vi "HandleObservationAsync.vi"(8 "error in (no error)":errorcluster, 10 "Acquisition.lvclass In":refnum<class "Acquisition.lvclass">, 11 "S4ACS_GUI in":refnum<class "S4GUI.lvclass">) -> (0 "error out":errorcluster, 2 "Acquisition.lvclass Out":refnum<class "Acquisition.lvclass">, 3 "S4ACS_GUI out":refnum<class "S4GUI.lvclass">)   [LabVIEW 2018, in "S4GUI.lvclass"]
uses:
  S4GUI.lvclass
  Acquisition/Acquisition.lvclass
  S4GUI.lvclass/S4GUI.ctl
  Instrument/Instrument.lvclass/Instrument.ctl
  Device/Optics/Optics.lvclass/Optics.ctl
  Interface/Interface.lvclass/Interface.ctl
  Server/Server.lvclass/Server.ctl
  Device/Optics/Opt_Selector/Opt_Selector.lvclass
  Instrument/Instrument.lvclass
  StateMachine/State Machine.lvclass
  SyncBox/Sync Box.lvclass
  Trigger/Trigger.lvclass
  Channel/Channel.lvclass
  Interface/Interface.lvclass
  TelFocus/TelFocus.lvclass
  SecMirror/SecMirror.lvclass
  Device/Optics/Optics.lvclass
  Server/Server.lvclass
panel:
  out "time308":u32
  out "time307":u32
  out "time9":u32
  out "delay 89":u32
  out "time 10":u32
  out "time elapsed 2":u32
  out "time 8":u32
  out "delay 78":u32
  out "time7":u32
  out "time6":u32
  out "time5":u32
  out "delay 3-4":u32
  out "time4":u32
  out "time3":u32
  out "time 2":u32
  out "time1":u32
  # "ACS DELAY"
  # "WAVEPLATE DURATION"
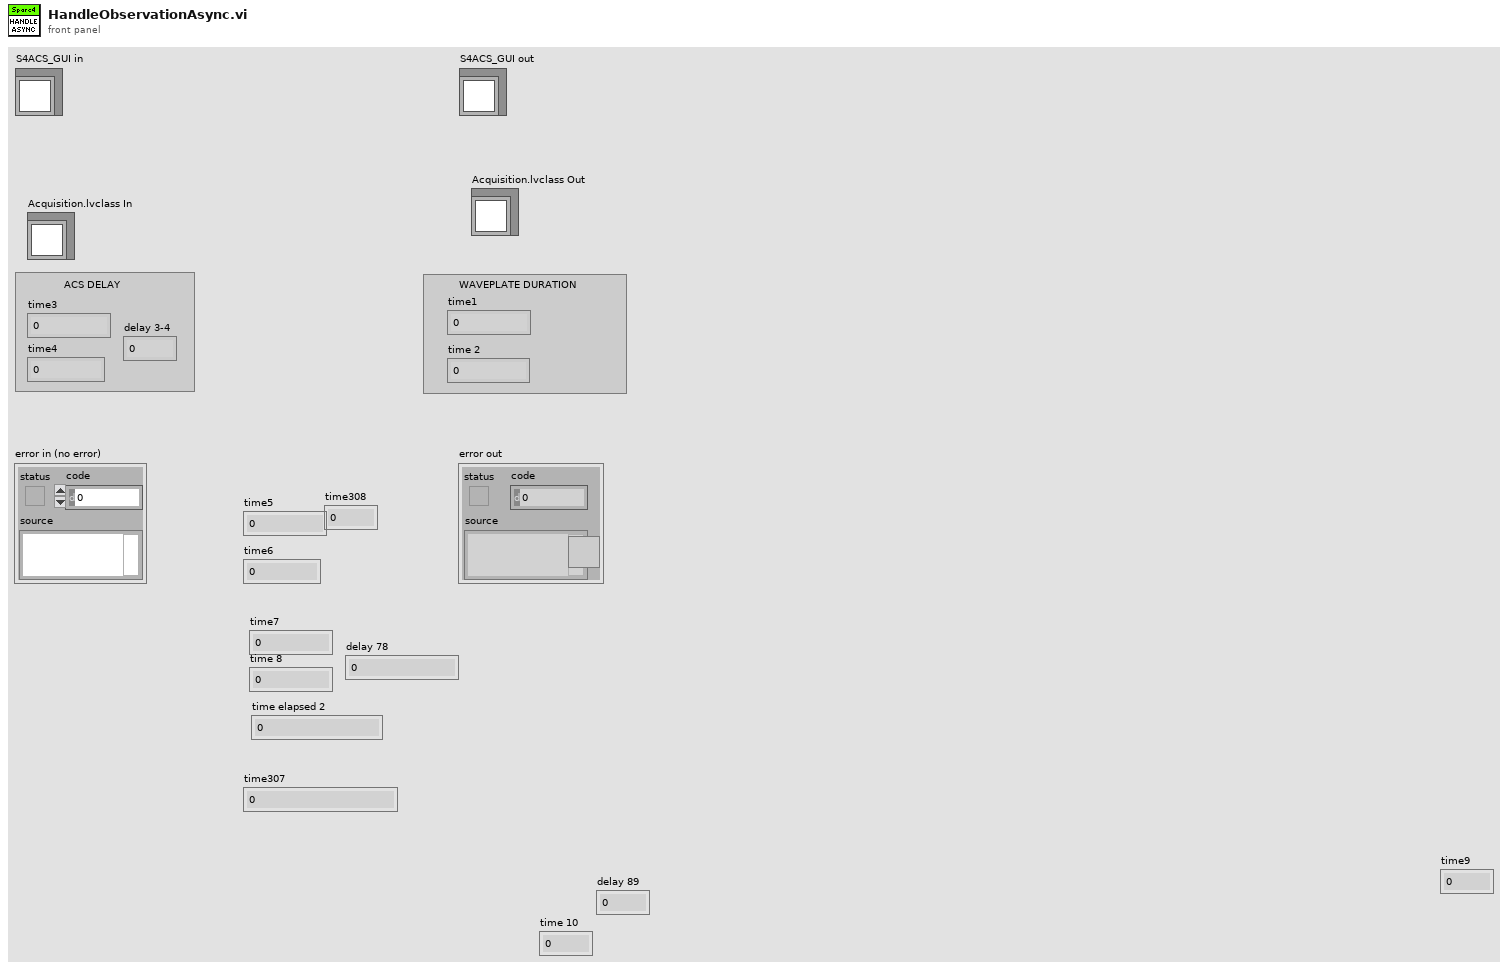
[diagram p1: front panel]
types:
  T1 = cluster{"ACQUISITION_MODE":u8, "TRIGGER_MODE":u8, "READ_MODE":u8, "PREAMP":u8, "READOUT_RATE":u8, "VERTICAL_SHIFT_SPEED":u8, "EM_MODE":u8, "EM_GAIN":u16, "SHUTTER_MODE":u8, "SHUTTER_TTL":u8, "SHUTTER_OPENING_TIME":u16, "SHUTTER_CLOSING_TIME":u16, "VBIN":u16, "HBIN":u16, "INITIAL_LINE":u16, "INITIAL_COLUMN":u16, "FINAL_LINE":u16, "FINAL_COLUMN":u16, "FRAME_TRANSFER":bool, "VERTICAL_CLOCK_VOLTAGE":u8, "AD_CHANNEL":u32}
  T2 = cluster{"Texp":dbl, "Nimages":u32, "InitialLine":u32, "FinalLine":u32, "InitialColumn":u32, "FinalColumn":u32, "EmGain":u32, "Cooler Off":bool, "CyclesDone":u32, "SequesDone":u32, "UsedDiskSpace":u16, "Error":bool}
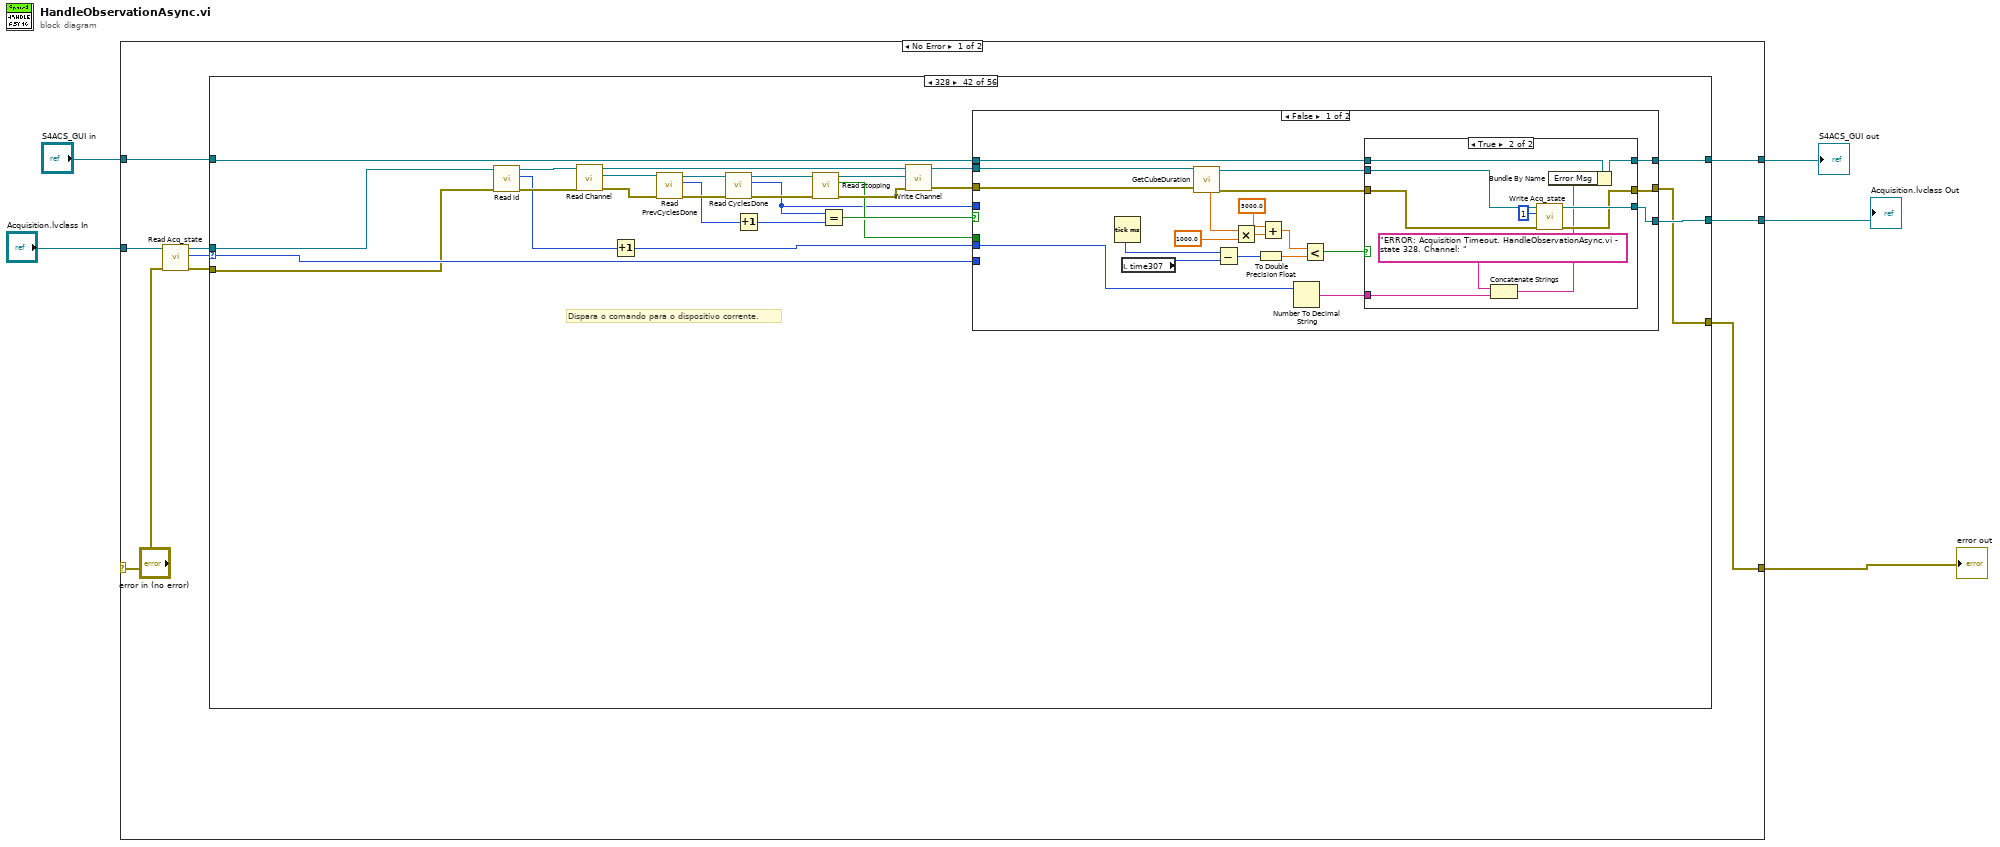
[diagram p0: block diagram]
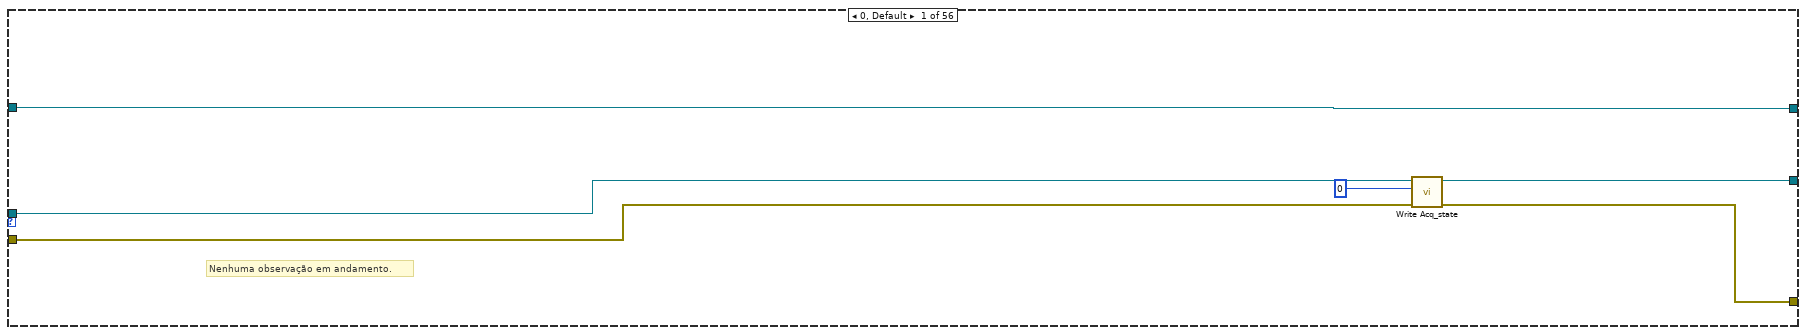
[diagram p2: hidden frame]
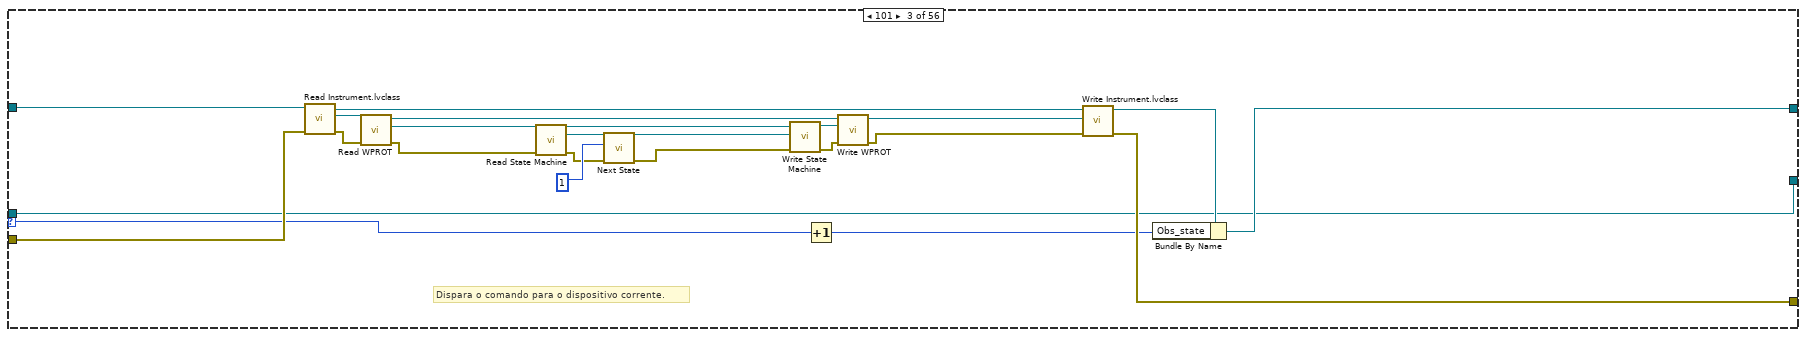
[diagram p4: hidden frame]
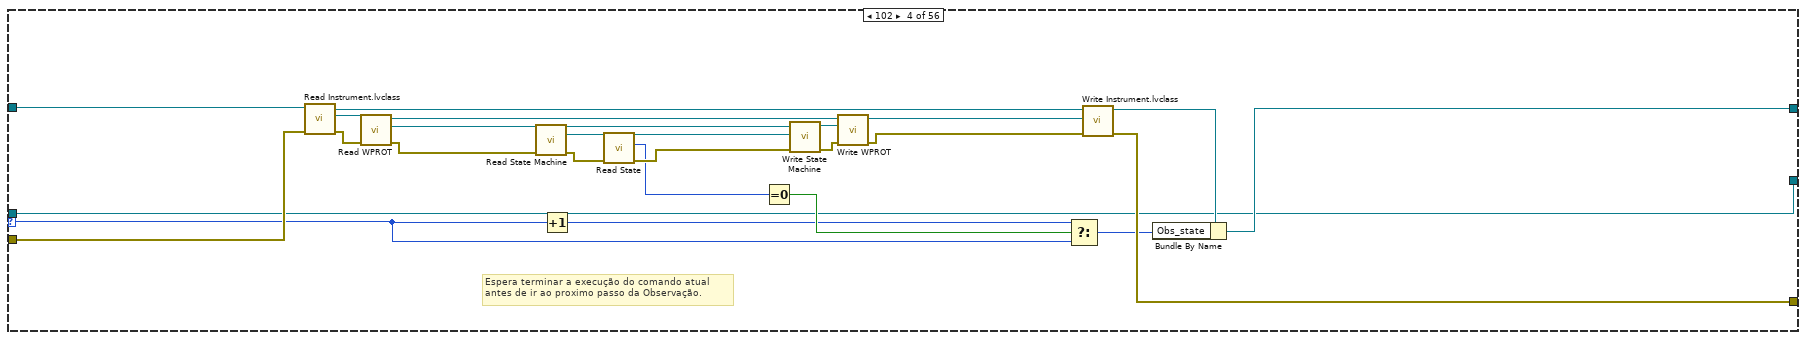
[diagram p5: hidden frame]
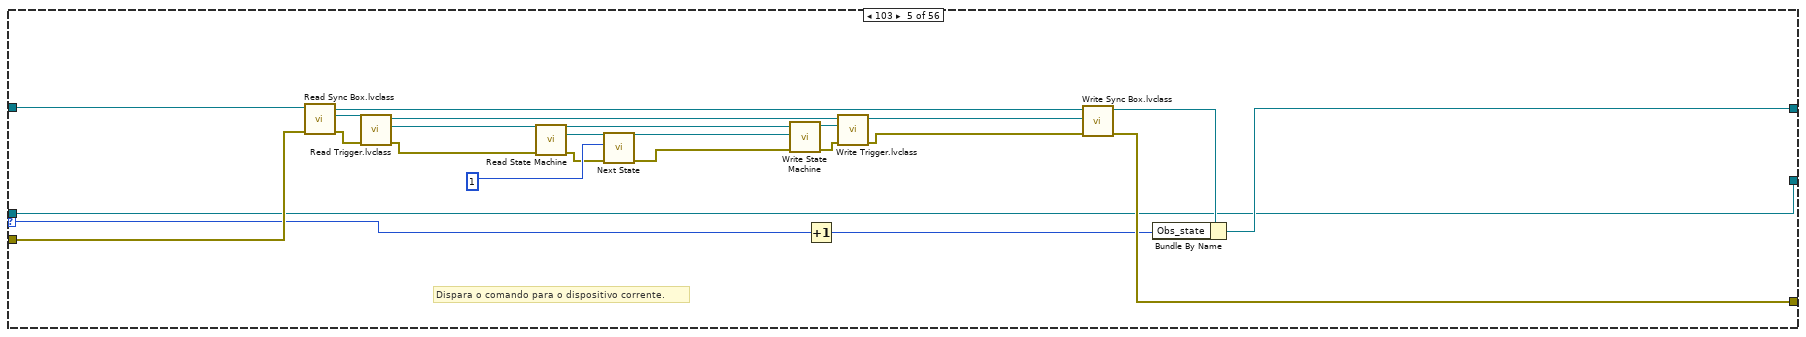
[diagram p6: hidden frame]
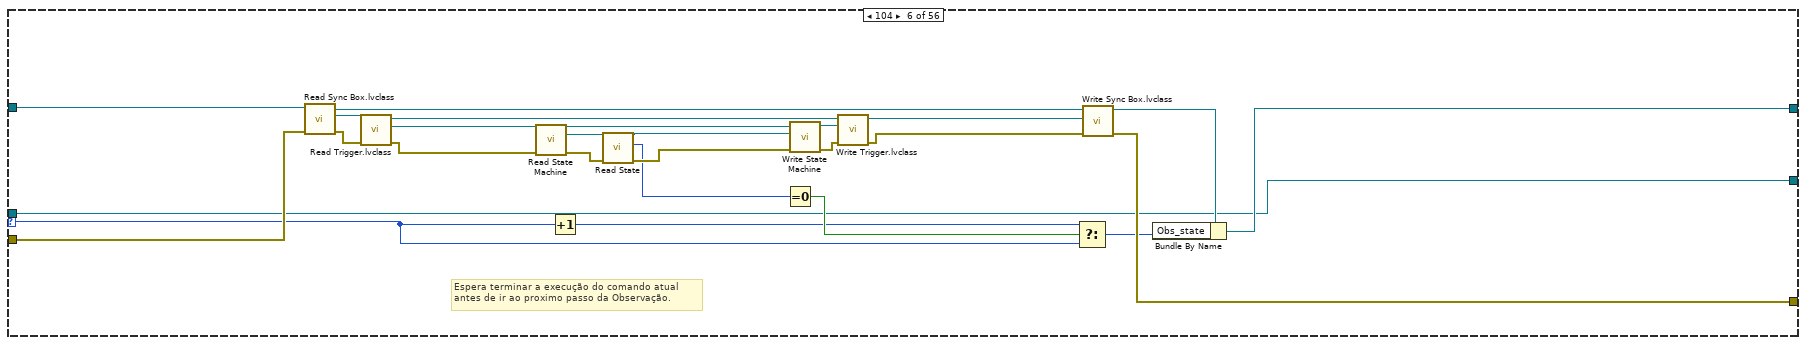
[diagram p7: hidden frame]
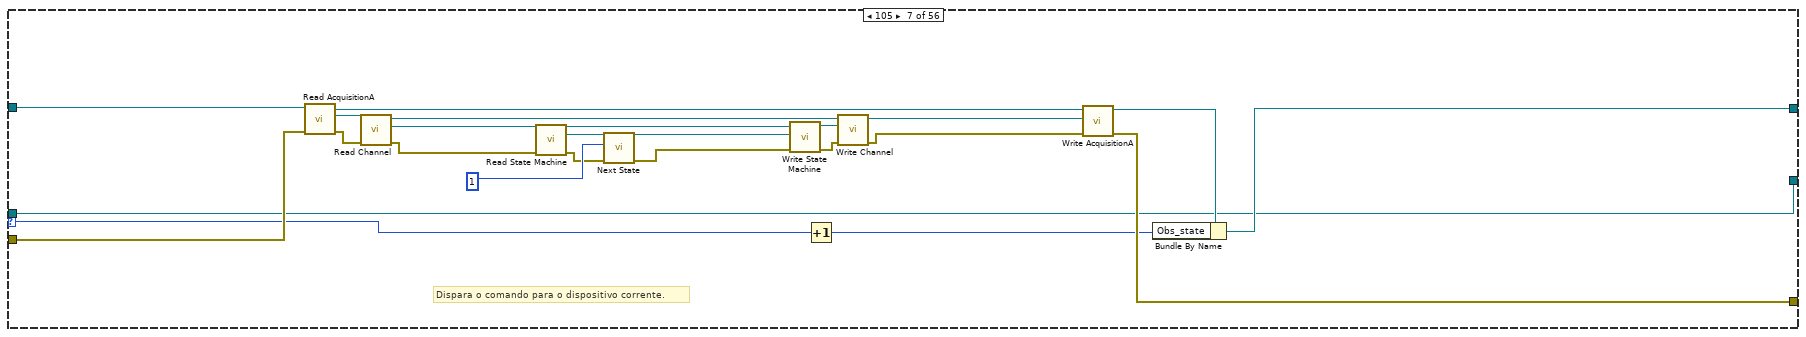
[diagram p8: hidden frame]
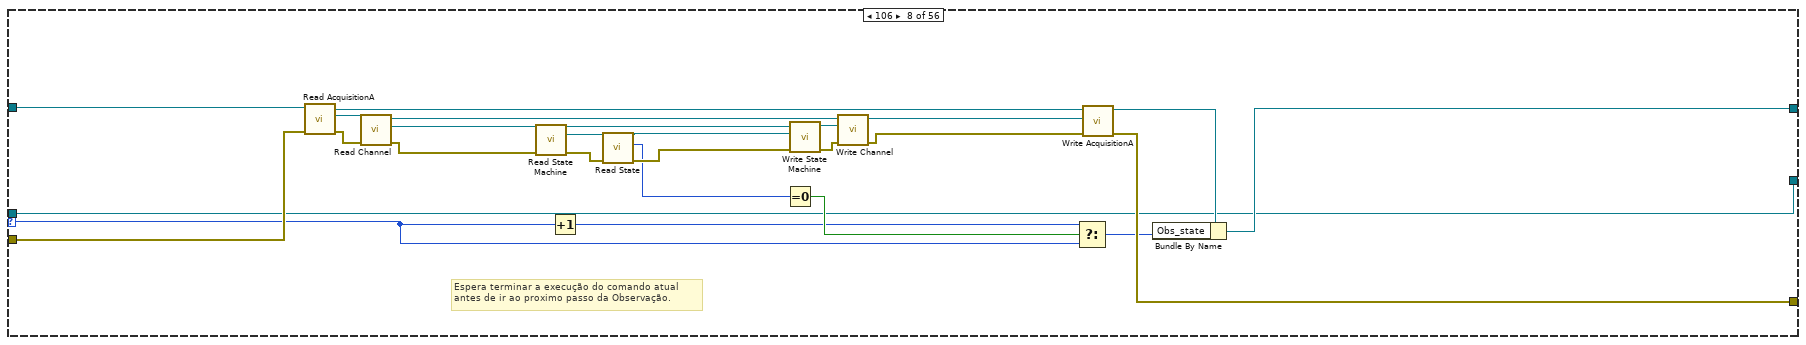
[diagram p9: hidden frame]
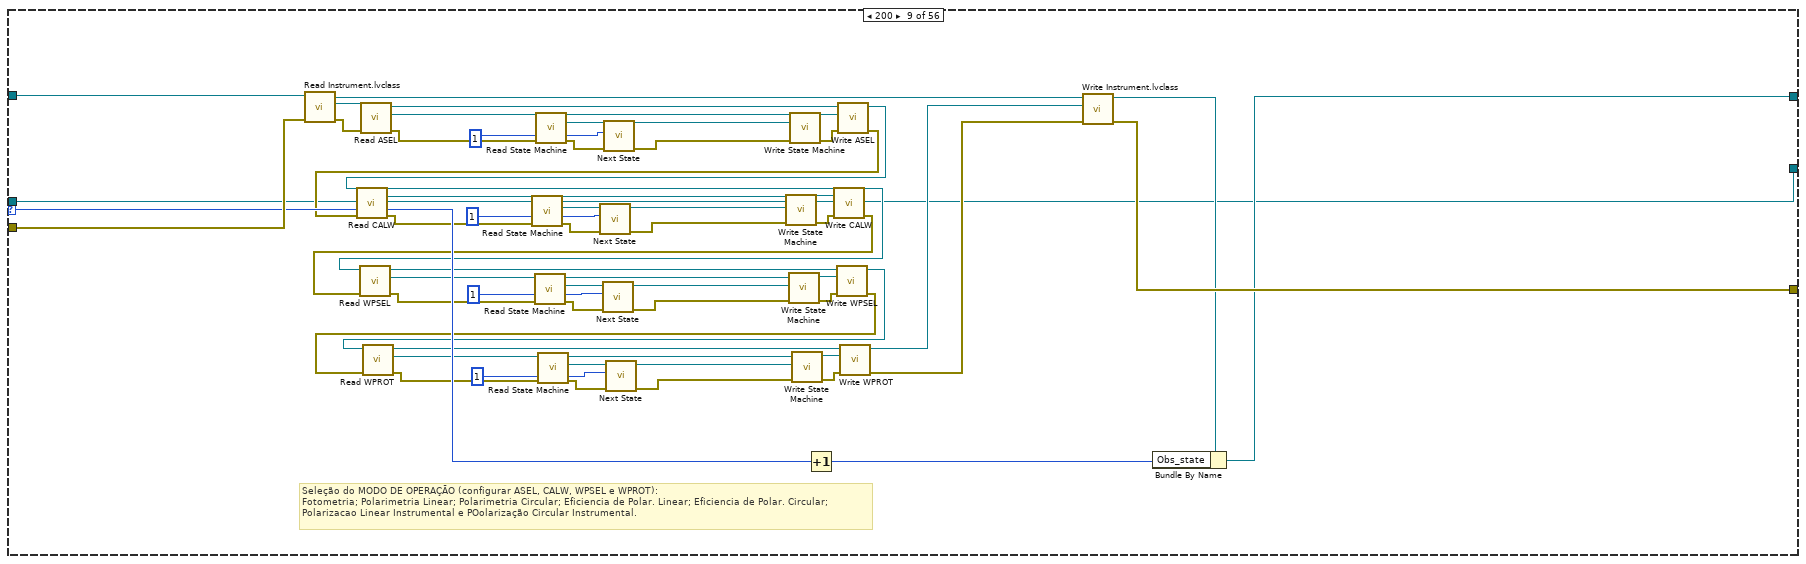
[diagram p10: hidden frame]
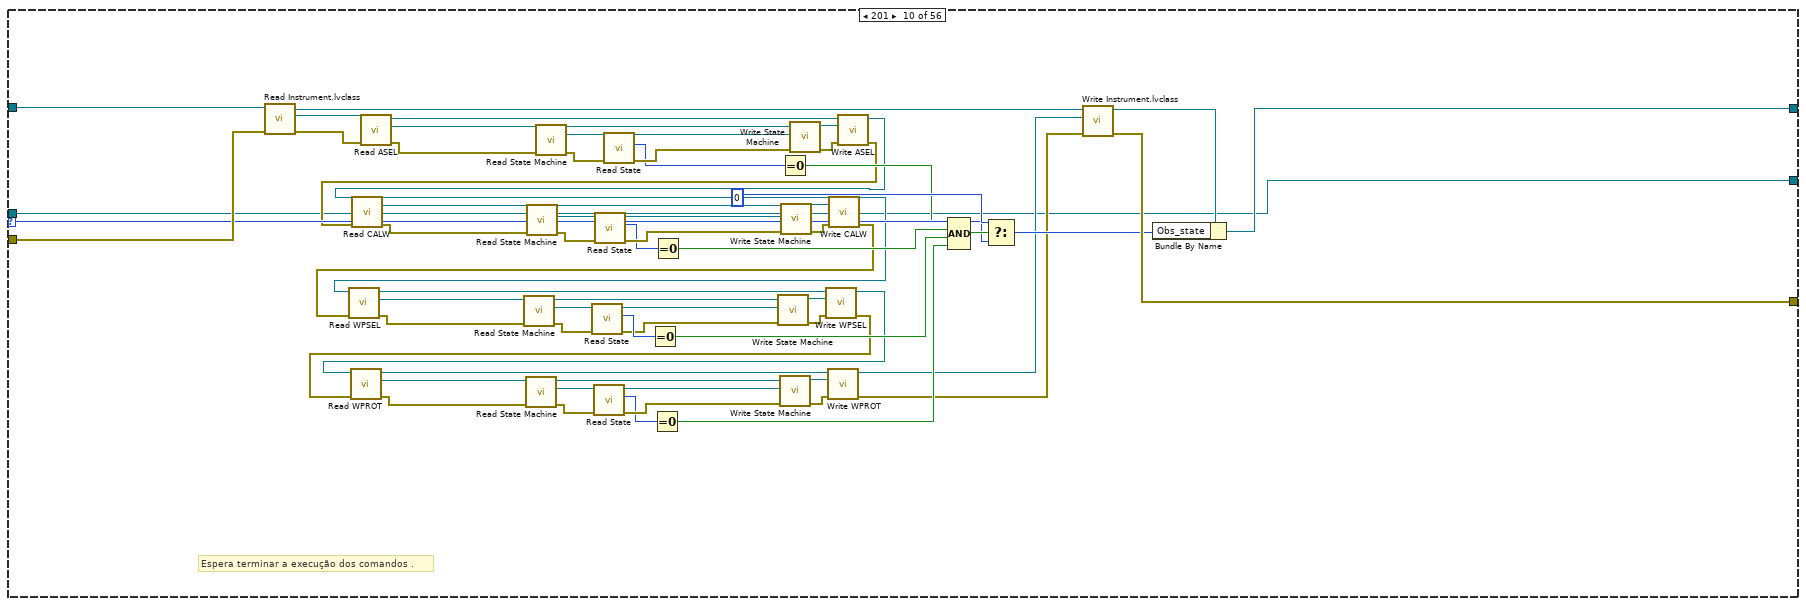
[diagram p11: hidden frame]
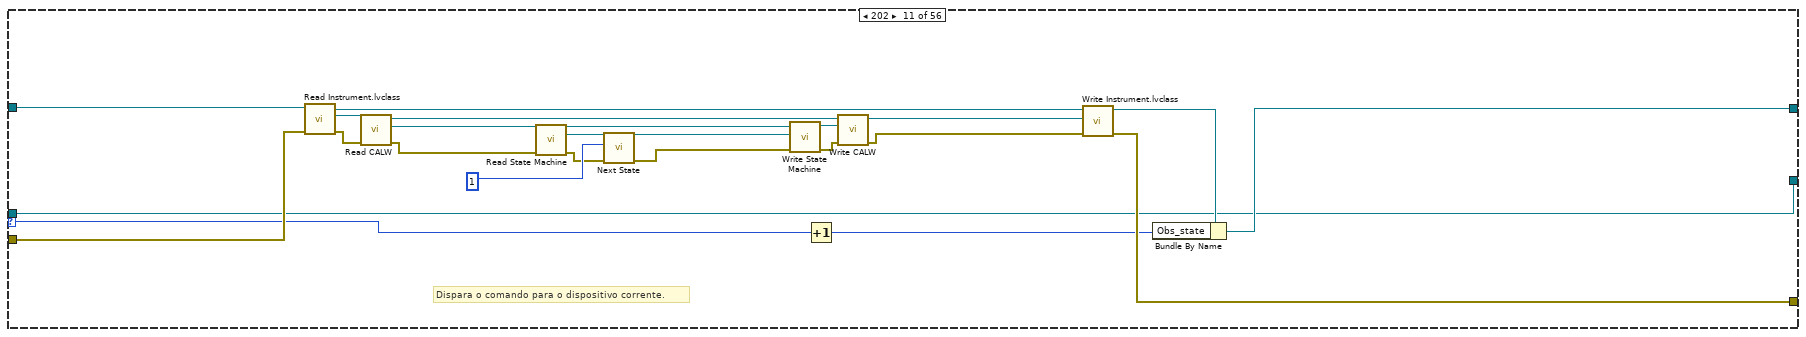
[diagram p12: hidden frame]
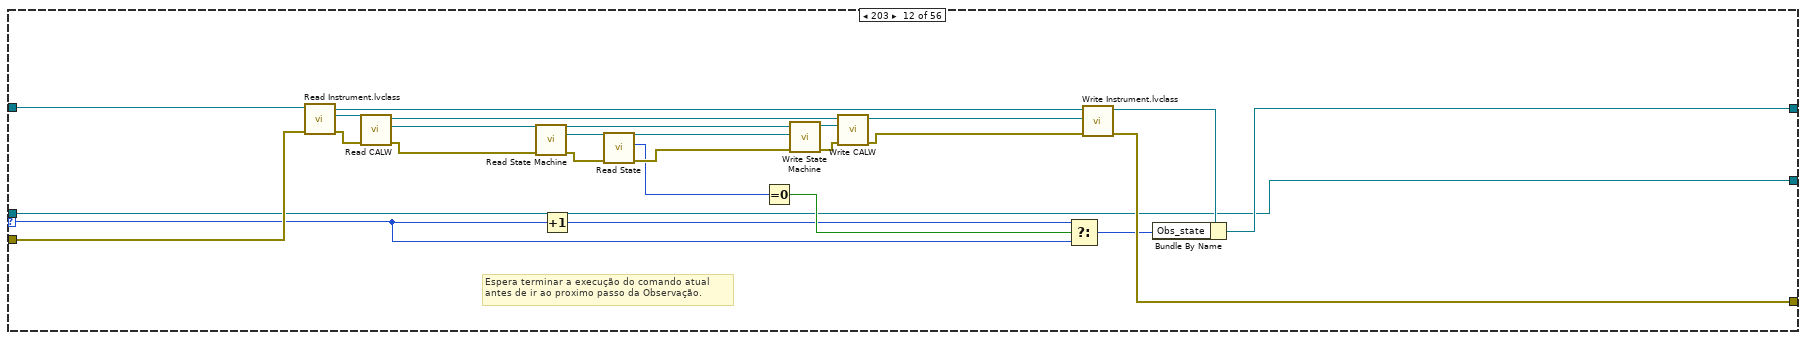
[diagram p13: hidden frame]
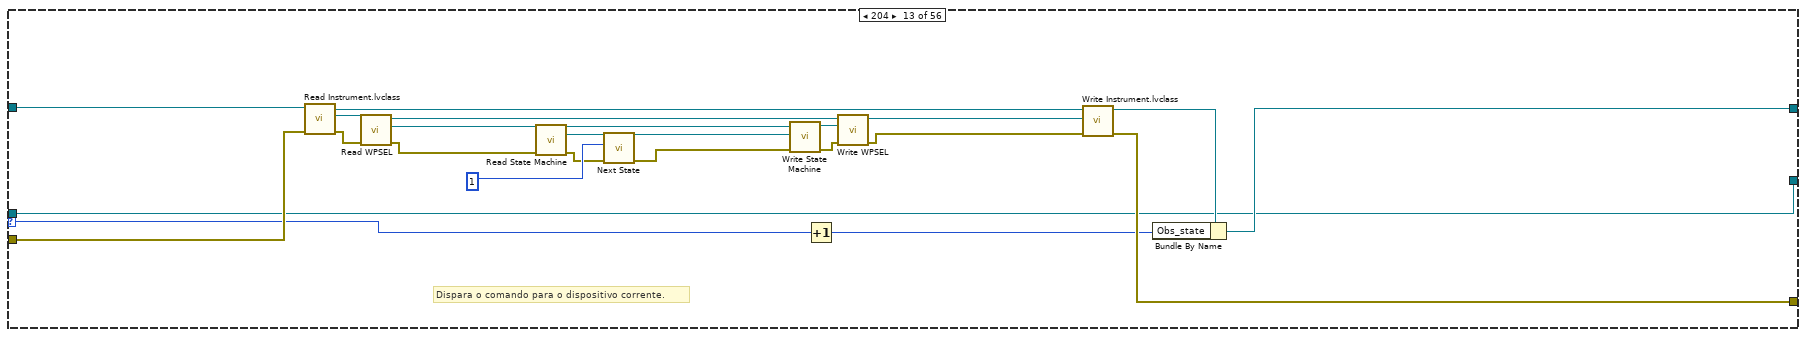
[diagram p14: hidden frame]
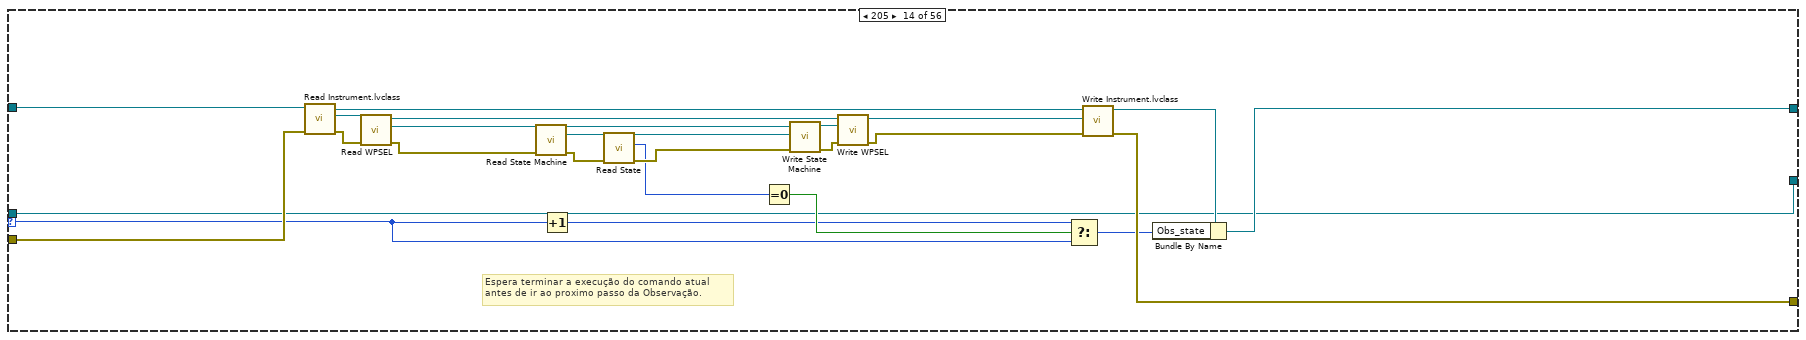
[diagram p15: hidden frame]
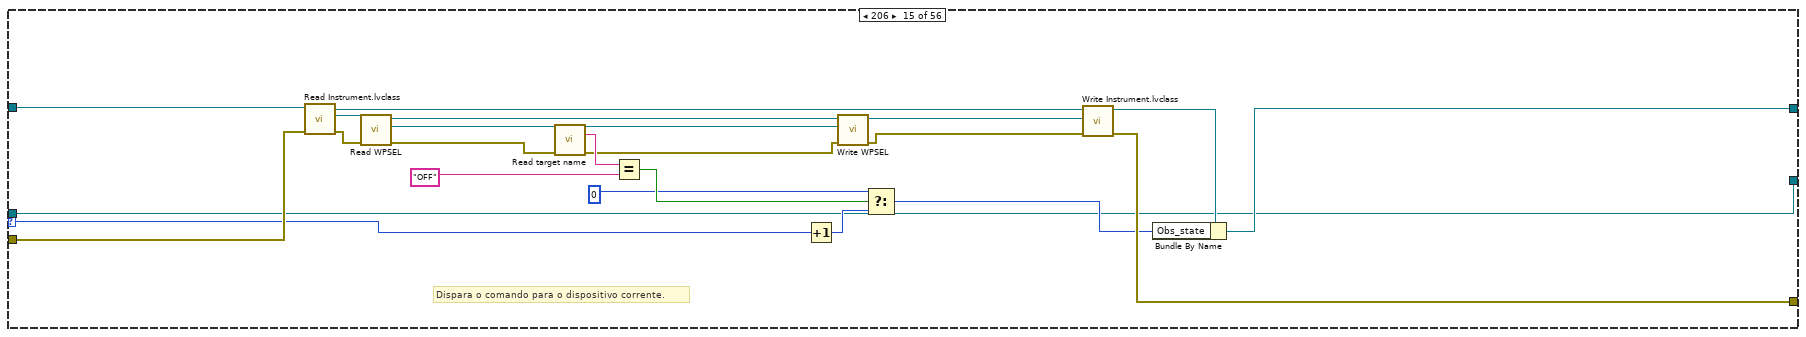
[diagram p16: hidden frame]
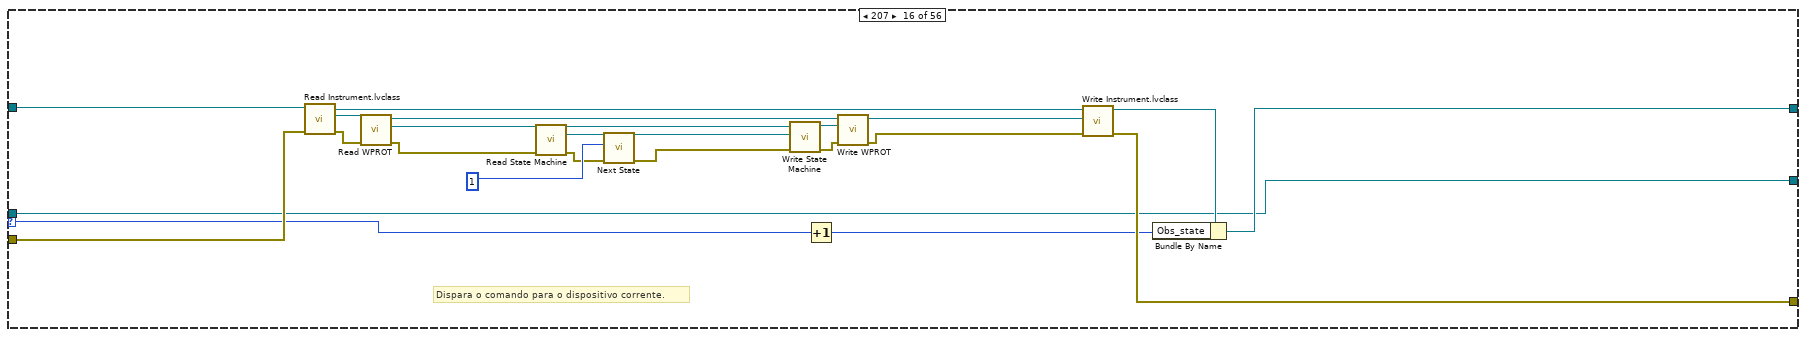
[diagram p17: hidden frame]
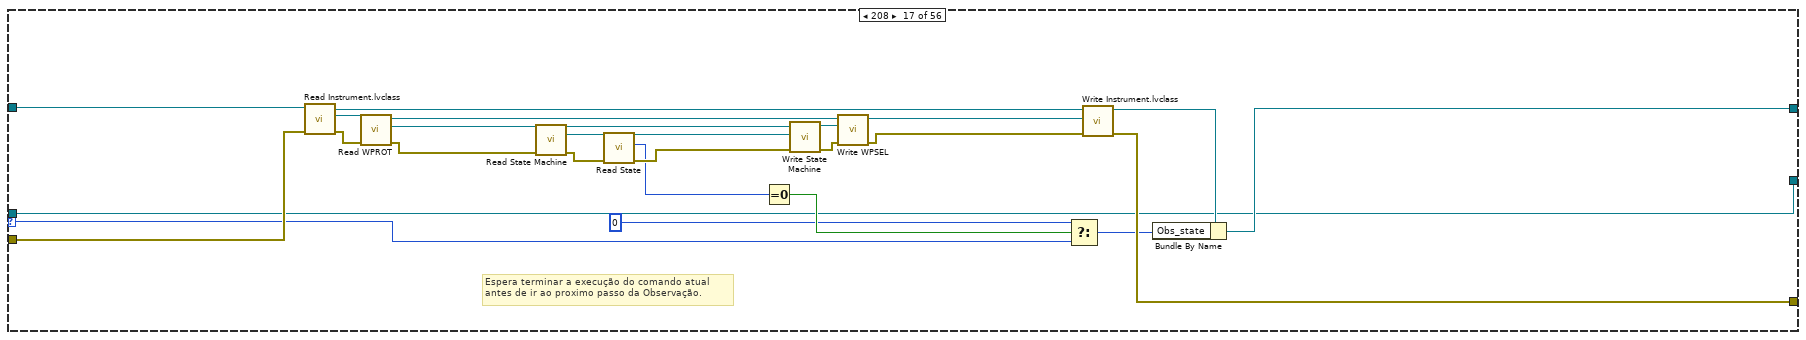
[diagram p18: hidden frame]
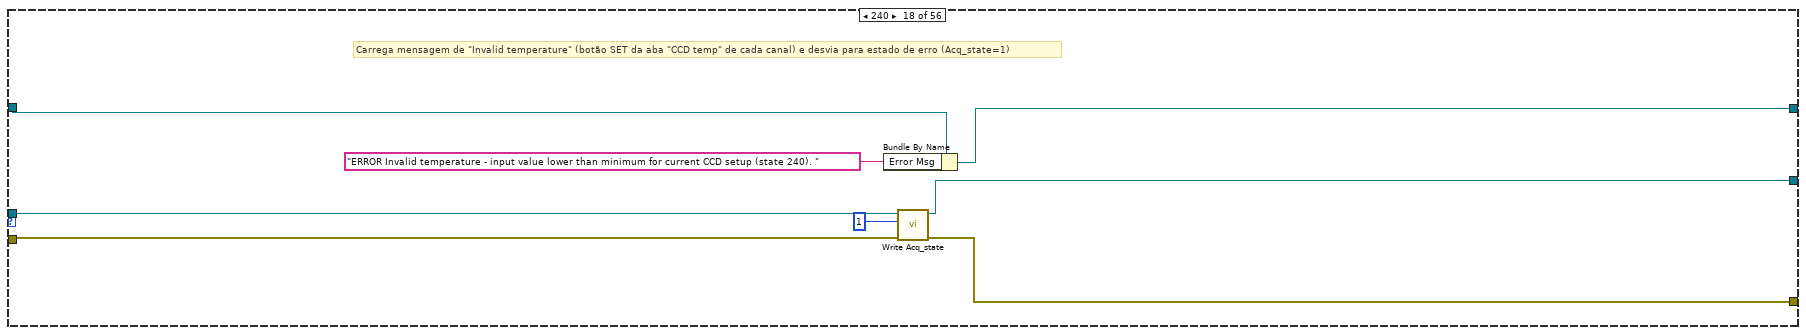
[diagram p19: hidden frame]
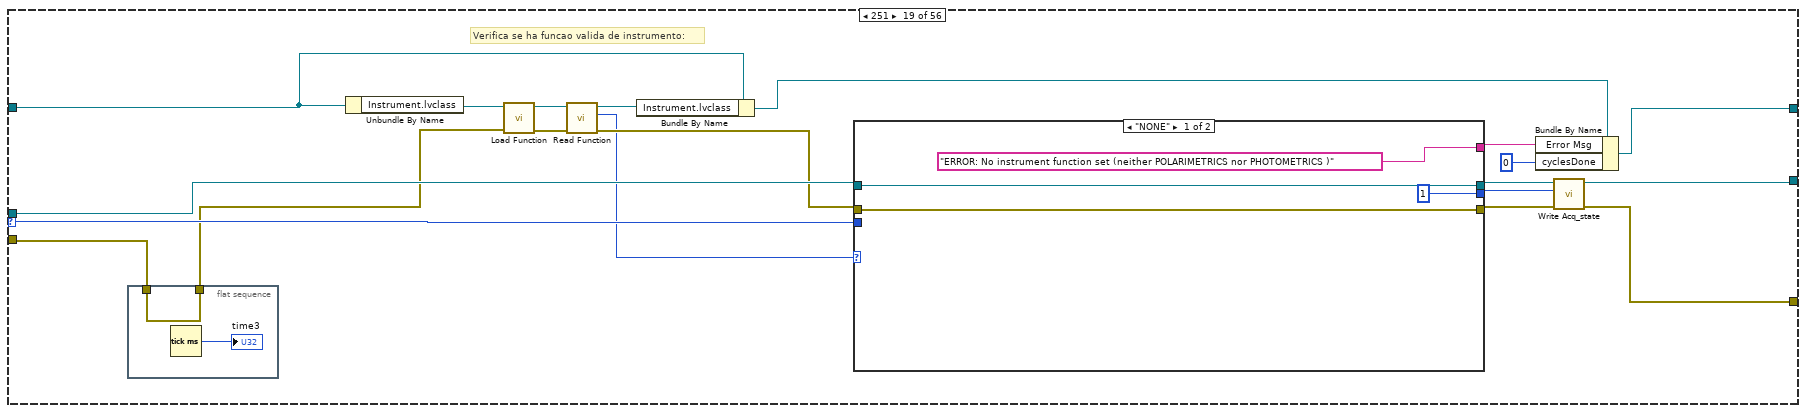
[diagram p20: hidden frame]
diagram:
  n1 = case shown="No Error" "error in (no error)" {
    selector: "error in (no error)" -> [w9 w1903]
    tunnel: [w15 w1903] -> w5
    tunnel: [w14 w1902] -> w3
    tunnel: "S4ACS_GUI in" -> [w13 w1902]
    tunnel: "Acquisition.lvclass In" -> [w12 w1901]
    tunnel: [w7 w1901] -> w1
    frame No Error {
      n2 = call-dynamic "Read Acq_state.vi"("error in (no error)"=w9, "Acquisition in"=w12) -> ("error out"=w8:errorcluster, "Acq_state"=w10:u32, "Acquisition out"=w11:refnum<class "Acquisition.lvclass">)  [unwired: 7 in]
      n3 = case shown="328" w10 {
        selector: w10 -> [_ _ w28 w51 w78 w101 w128 w151 w220 w284 w310 w333 w360 w383 w419 w433 w456 _ w507 w538 w611 w618 w661 w674 _ w766 w776 w840 w889 w951 w975 w1017 w1063 _ w1162 w1172 w1200 w1240 w1276 w1311 w1367 w1451 _ w1553 _ w1640 w1689 w1738 w1761 w1777 w1802 w1821 w1846 _ _ _]
        tunnel: w13 -> [w16 w24 w42 w68 w92 w118 w142 w168 w234 w302 w324 w350 w374 w400 w423 w447 w473 w482 w492 w536 w581 w625 w642 w672 w741 w751 w775 w841 w925 w947 w965 w1006 w1066 w1099 w1152 w1171 w1191 w1218 w1268 w1306 w1362 w1446 w1513 w1552 w1626 w1642 w1691 w1734 w1752 w1783 w1798 w1812 w1839 w1872 w1880 w1883]
        tunnel: [w16 w24 w26 w55 w76 w109 w126 w159 w218 w289 w308 w337 w358 w387 w418 w431 w460 w483 w498 w535 w581 w625 w645 w671 w727 w756 w775 w808 w898 w947 w963 w996 w1065 w1098 w1150 w1171 w1190 w1217 w1270 w1305 w1363 w1447 w1509 w1552 w1626 w1639 w1675 w1734 w1756 w1783 w1798 w1816 w1839 w1867 w1880 w1885] -> w14
        tunnel: w8 -> [w20 w23 w41 w67 w91 w117 w141 w167 w233 w301 w323 w349 w373 w399 w422 w446 w472 w484 w500 w548 w582 w619 w648 w684 w732 w750 w789 w805 w913 w952 w973 w1001 w1072 w1103 w1160 w1185 w1188 w1214 w1261 w1296 w1347 w1431 w1524 w1556 w1620 w1641 w1690 w1736 w1766 w1780 w1800 w1829 w1859 w1871 w1879 w1882]
        tunnel: [w17 w23 w40 w66 w90 w116 w140 w166 w232 w300 w322 w348 w372 w398 w421 w445 w471 w485 w501 w549 w615 w620 w649 w685 w734 w760 w787 w807 w917 w949 w968 w1020 w1070 w1100 w1155 w1183 w1194 w1238 w1271 w1316 w1350 w1434 w1529 w1554 w1627 w1633 w1671 w1727 w1762 w1781 w1794 w1825 w1855 w1865 w1879 w1884] -> w15
        tunnel: w11 -> [w19 w22 w25 w49 w75 w99 w125 w149 w175 w238 w307 w331 w357 w381 w407 w430 w454 w487 w506 w553 w614 w626 w653 w689 w726 w765 w790 w795 w897 w953 w974 w987 w1073 w1102 w1161 w1186 w1199 w1216 w1266 w1299 w1348 w1432 w1525 w1557 w1621 w1637 w1674 w1737 w1767 w1778 w1801 w1830 w1860 w1870 w1878 w1881]
        tunnel: [w18 w22 w25 w49 w75 w99 w125 w149 w175 w238 w307 w331 w357 w381 w407 w430 w454 w486 w503 w550 w616 w621 w650 w686 w733 w761 w788 w806 w916 w948 w969 w1021 w1071 w1101 w1156 w1184 w1198 w1239 w1275 w1317 w1366 w1450 w1530 w1555 w1628 w1636 w1672 w1731 w1763 w1782 w1795 w1826 w1856 w1866 w1878 w1881] -> w7
        frame 0, Default {
          # "Nenhuma observação em andamento."
          n4 = call-dynamic "Write Acq_state.vi"("error in (no error)"=w20, "Acq_state"=u32 0 ("Obs_state"), "Acquisition in"=w19) -> ("error out"=w17:errorcluster, "Acquisition out"=w18:refnum<class "Acquisition.lvclass">)  [unwired: 7 in]
        }
        frame 1 {
          # "Estado de erro!\nFica aqui até acionar STOP ou ABORT."
          # "Nenhuma observação em andamento."
        }
        frame 101 {
          # "Dispara o comando para o dispositivo corrente."
          n5 = call "Read Instrument.lvclass.vi"("error in (no error)"=w41, "S4ACS_GUI in"=w42) -> ("error out"=w47:errorcluster, "Instrument.lvclass"=w48:refnum<class "Instrument.lvclass">, "S4ACS_GUI out"=w44:refnum<class "S4GUI.lvclass">)  [unwired: 7 in]
          n6 = call "Read WPROT.vi"("error in (no error)"=w47, "Instrument in"=w48) -> ("error out"=w34:errorcluster, "Opt_Selector.lvclass"=w33:refnum<class "Opt_Selector.lvclass">, "Instrument out"=w46:refnum<class "Instrument.lvclass">)  [unwired: 7 in]
          n7 = call-dynamic "Read State Machine.vi"("error in (no error)"=w34, "Device in"=w33) -> ("error out"=w37:errorcluster, "State Machine.lvclass"=w39:refnum<class "State Machine.lvclass">, "Device out"=w31:refnum<class "Opt_Selector.lvclass">)  [unwired: 7 in]
          n8 = call "Next State.vi"("error in (no error)"=w37, "New_State"=1, "State Machine in"=w39) -> ("error out"=w36:errorcluster, "State Machine out"=w35:refnum<class "State Machine.lvclass">)  [unwired: 7 in]
          n9 = call-dynamic "Write State Machine.vi"("error in (no error)"=w36, "State Machine.lvclass"=w35, "Device in"=w31) -> ("error out"=w30:errorcluster, "Device out"=w32:refnum<class "Opt_Selector.lvclass">)  [unwired: 7 in]
          n10 = Increment(x=w28) -> (x+1=w27:u32)
          n11 = call "Write WPROT.vi"("error in (no error)"=w30, "Opt_Selector.lvclass"=w32, "Instrument in"=w46) -> ("error out"=w43:errorcluster, "Instrument out"=w45:refnum<class "Instrument.lvclass">)  [unwired: 7 in]
          n12 = call "Write Instrument.lvclass.vi"("error in (no error)"=w43, "Instrument.lvclass"=w45, "S4ACS_GUI in"=w44) -> ("error out"=w40:errorcluster, "S4ACS_GUI out"=w29:refnum<class "S4GUI.lvclass">)  [unwired: 7 in]
          n13 = Bundle By Name(cluster=w29, "Obs_state"=w27) -> (w26:refnum<class "S4GUI.lvclass">)
        }
        frame 102 {
          # "Espera terminar a execução do comando atual \nantes de ir ao proximo passo da Observação."
          n14 = call "Read Instrument.lvclass.vi"("error in (no error)"=w67, "S4ACS_GUI in"=w68) -> ("error out"=w73:errorcluster, "Instrument.lvclass"=w74:refnum<class "Instrument.lvclass">, "S4ACS_GUI out"=w70:refnum<class "S4GUI.lvclass">)  [unwired: 7 in]
          n15 = call "Read WPROT.vi"("error in (no error)"=w73, "Instrument in"=w74) -> ("error out"=w61:errorcluster, "Opt_Selector.lvclass"=w60:refnum<class "Opt_Selector.lvclass">, "Instrument out"=w72:refnum<class "Instrument.lvclass">)  [unwired: 7 in]
          n16 = call-dynamic "Read State Machine.vi"("error in (no error)"=w61, "Device in"=w60) -> ("error out"=w64:errorcluster, "State Machine.lvclass"=w65:refnum<class "State Machine.lvclass">, "Device out"=w58:refnum<class "Opt_Selector.lvclass">)  [unwired: 7 in]
          n17 = Increment(x=w51) -> (x+1=w50:u32)
          n18 = call-dynamic "Read State.vi"("error in (no error)"=w64, "State Machine in"=w65) -> ("error out"=w63:errorcluster, "State"=w53:i32, "State Machine out"=w62:refnum<class "State Machine.lvclass">)  [unwired: 7 in]
          n19 = Equal To 0?(x=w53) -> (x = 0?=w54:bool)
          n20 = call-dynamic "Write State Machine.vi"("error in (no error)"=w63, "State Machine.lvclass"=w62, "Device in"=w58) -> ("error out"=w57:errorcluster, "Device out"=w59:refnum<class "Opt_Selector.lvclass">)  [unwired: 7 in]
          n21 = call "Write WPROT.vi"("error in (no error)"=w57, "Opt_Selector.lvclass"=w59, "Instrument in"=w72) -> ("error out"=w69:errorcluster, "Instrument out"=w71:refnum<class "Instrument.lvclass">)  [unwired: 7 in]
          n22 = Select(t=w50, s=w54, f=w51) -> (s? t:f=w52:u32)
          n23 = call "Write Instrument.lvclass.vi"("error in (no error)"=w69, "Instrument.lvclass"=w71, "S4ACS_GUI in"=w70) -> ("error out"=w66:errorcluster, "S4ACS_GUI out"=w56:refnum<class "S4GUI.lvclass">)  [unwired: 7 in]
          n24 = Bundle By Name(cluster=w56, "Obs_state"=w52) -> (w55:refnum<class "S4GUI.lvclass">)
        }
        frame 103 {
          # "Dispara o comando para o dispositivo corrente."
          n25 = call-dynamic "Read Sync Box.lvclass.vi"("error in (no error)"=w91, "SPARC4_AC in"=w92) -> ("error out"=w97:errorcluster, "Sync Box.lvclass"=w98:refnum<class "Sync Box.lvclass">, "SPARC4_AC out"=w94:refnum<class "S4GUI.lvclass">)  [unwired: 7 in]
          n26 = call-dynamic "Read Trigger.lvclass.vi"("error in (no error)"=w97, "Sync Box in"=w98) -> ("error out"=w84:errorcluster, "Trigger.lvclass"=w83:refnum<class "Trigger.lvclass">, "Sync Box out"=w96:refnum<class "Sync Box.lvclass">)  [unwired: 7 in]
          n27 = call-dynamic "Read State Machine.vi"("error in (no error)"=w84, "Device in"=w83) -> ("error out"=w87:errorcluster, "State Machine.lvclass"=w89:refnum<class "State Machine.lvclass">, "Device out"=w81:refnum<class "Trigger.lvclass">)  [unwired: 7 in]
          n28 = call "Next State.vi"("error in (no error)"=w87, "New_State"=1, "State Machine in"=w89) -> ("error out"=w86:errorcluster, "State Machine out"=w85:refnum<class "State Machine.lvclass">)  [unwired: 7 in]
          n29 = call-dynamic "Write State Machine.vi"("error in (no error)"=w86, "State Machine.lvclass"=w85, "Device in"=w81) -> ("error out"=w80:errorcluster, "Device out"=w82:refnum<class "Trigger.lvclass">)  [unwired: 7 in]
          n30 = Increment(x=w78) -> (x+1=w77:u32)
          n31 = call-dynamic "Write Trigger.lvclass.vi"("error in (no error)"=w80, "Trigger.lvclass"=w82, "Sync Box in"=w96) -> ("error out"=w93:errorcluster, "Sync Box out"=w95:refnum<class "Sync Box.lvclass">)  [unwired: 7 in]
          n32 = call-dynamic "Write Sync Box.lvclass.vi"("error in (no error)"=w93, "Sync Box.lvclass"=w95, "SPARC4_AC in"=w94) -> ("error out"=w90:errorcluster, "SPARC4_AC out"=w79:refnum<class "S4GUI.lvclass">)  [unwired: 7 in]
          n33 = Bundle By Name(cluster=w79, "Obs_state"=w77) -> (w76:refnum<class "S4GUI.lvclass">)
        }
        frame 104 {
          # "Espera terminar a execução do comando atual \nantes de ir ao proximo passo da Observação."
          n34 = call-dynamic "Read Sync Box.lvclass.vi"("error in (no error)"=w117, "SPARC4_AC in"=w118) -> ("error out"=w123:errorcluster, "Sync Box.lvclass"=w124:refnum<class "Sync Box.lvclass">, "SPARC4_AC out"=w120:refnum<class "S4GUI.lvclass">)  [unwired: 7 in]
          n35 = call-dynamic "Read Trigger.lvclass.vi"("error in (no error)"=w123, "Sync Box in"=w124) -> ("error out"=w115:errorcluster, "Trigger.lvclass"=w114:refnum<class "Trigger.lvclass">, "Sync Box out"=w122:refnum<class "Sync Box.lvclass">)  [unwired: 7 in]
          n36 = call-dynamic "Read State Machine.vi"("error in (no error)"=w115, "Device in"=w114) -> ("error out"=w106:errorcluster, "State Machine.lvclass"=w108:refnum<class "State Machine.lvclass">, "Device out"=w112:refnum<class "Trigger.lvclass">)  [unwired: 7 in]
          n37 = Increment(x=w101) -> (x+1=w103:u32)
          n38 = call-dynamic "Read State.vi"("error in (no error)"=w106, "State Machine in"=w108) -> ("error out"=w105:errorcluster, "State"=w100:i32, "State Machine out"=w107:refnum<class "State Machine.lvclass">)  [unwired: 7 in]
          n39 = Equal To 0?(x=w100) -> (x = 0?=w104:bool)
          n40 = call-dynamic "Write State Machine.vi"("error in (no error)"=w105, "State Machine.lvclass"=w107, "Device in"=w112) -> ("error out"=w111:errorcluster, "Device out"=w113:refnum<class "Trigger.lvclass">)  [unwired: 7 in]
          n41 = call-dynamic "Write Trigger.lvclass.vi"("error in (no error)"=w111, "Trigger.lvclass"=w113, "Sync Box in"=w122) -> ("error out"=w119:errorcluster, "Sync Box out"=w121:refnum<class "Sync Box.lvclass">)  [unwired: 7 in]
          n42 = Select(t=w103, s=w104, f=w101) -> (s? t:f=w102:u32)
          n43 = call-dynamic "Write Sync Box.lvclass.vi"("error in (no error)"=w119, "Sync Box.lvclass"=w121, "SPARC4_AC in"=w120) -> ("error out"=w116:errorcluster, "SPARC4_AC out"=w110:refnum<class "S4GUI.lvclass">)  [unwired: 7 in]
          n44 = Bundle By Name(cluster=w110, "Obs_state"=w102) -> (w109:refnum<class "S4GUI.lvclass">)
        }
        frame 105 {
          # "Dispara o comando para o dispositivo corrente."
          n45 = call-dynamic "Read AcquisitionA.vi"("error in (no error)"=w141, "S4ACS_GUI in"=w142) -> ("error out"=w147:errorcluster, "Acquisition.lvclass"=w148:refnum<class "Acquisition.lvclass">, "S4ACS_GUI out"=w144:refnum<class "S4GUI.lvclass">)  [unwired: 7 in]
          n46 = call-dynamic "Read Channel.vi"("error in (no error)"=w147, "Acquisition in"=w148) -> ("error out"=w134:errorcluster, "Channel.lvclass"=w133:refnum<class "Channel.lvclass">, "Acquisition out"=w146:refnum<class "Acquisition.lvclass">)  [unwired: 7 in]
          n47 = call-dynamic "Read State Machine.vi"("error in (no error)"=w134, "Device in"=w133) -> ("error out"=w137:errorcluster, "State Machine.lvclass"=w139:refnum<class "State Machine.lvclass">, "Device out"=w131:refnum<class "Channel.lvclass">)  [unwired: 7 in]
          n48 = call "Next State.vi"("error in (no error)"=w137, "New_State"=1, "State Machine in"=w139) -> ("error out"=w136:errorcluster, "State Machine out"=w135:refnum<class "State Machine.lvclass">)  [unwired: 7 in]
          n49 = call-dynamic "Write State Machine.vi"("error in (no error)"=w136, "State Machine.lvclass"=w135, "Device in"=w131) -> ("error out"=w130:errorcluster, "Device out"=w132:refnum<class "Channel.lvclass">)  [unwired: 7 in]
          n50 = Increment(x=w128) -> (x+1=w127:u32)
          n51 = call-dynamic "Write Channel.vi"("error in (no error)"=w130, "Channel.lvclass"=w132, "Acquisition in"=w146) -> ("error out"=w143:errorcluster, "Acquisition out"=w145:refnum<class "Acquisition.lvclass">)  [unwired: 7 in]
          n52 = call-dynamic "Write AcquisitionA.vi"("error in (no error)"=w143, "Acquisition.lvclass"=w145, "S4ACS_GUI in"=w144) -> ("error out"=w140:errorcluster, "S4ACS_GUI out"=w129:refnum<class "S4GUI.lvclass">)  [unwired: 7 in]
          n53 = Bundle By Name(cluster=w129, "Obs_state"=w127) -> (w126:refnum<class "S4GUI.lvclass">)
        }
        frame 106 {
          # "Espera terminar a execução do comando atual \nantes de ir ao proximo passo da Observação."
          n54 = call-dynamic "Read AcquisitionA.vi"("error in (no error)"=w167, "S4ACS_GUI in"=w168) -> ("error out"=w173:errorcluster, "Acquisition.lvclass"=w174:refnum<class "Acquisition.lvclass">, "S4ACS_GUI out"=w170:refnum<class "S4GUI.lvclass">)  [unwired: 7 in]
          n55 = call-dynamic "Read Channel.vi"("error in (no error)"=w173, "Acquisition in"=w174) -> ("error out"=w165:errorcluster, "Channel.lvclass"=w164:refnum<class "Channel.lvclass">, "Acquisition out"=w172:refnum<class "Acquisition.lvclass">)  [unwired: 7 in]
          n56 = call-dynamic "Read State Machine.vi"("error in (no error)"=w165, "Device in"=w164) -> ("error out"=w156:errorcluster, "State Machine.lvclass"=w158:refnum<class "State Machine.lvclass">, "Device out"=w162:refnum<class "Channel.lvclass">)  [unwired: 7 in]
          n57 = Increment(x=w151) -> (x+1=w153:u32)
          n58 = call-dynamic "Read State.vi"("error in (no error)"=w156, "State Machine in"=w158) -> ("error out"=w155:errorcluster, "State"=w150:i32, "State Machine out"=w157:refnum<class "State Machine.lvclass">)  [unwired: 7 in]
          n59 = Equal To 0?(x=w150) -> (x = 0?=w154:bool)
          n60 = call-dynamic "Write State Machine.vi"("error in (no error)"=w155, "State Machine.lvclass"=w157, "Device in"=w162) -> ("error out"=w161:errorcluster, "Device out"=w163:refnum<class "Channel.lvclass">)  [unwired: 7 in]
          n61 = call-dynamic "Write Channel.vi"("error in (no error)"=w161, "Channel.lvclass"=w163, "Acquisition in"=w172) -> ("error out"=w169:errorcluster, "Acquisition out"=w171:refnum<class "Acquisition.lvclass">)  [unwired: 7 in]
          n62 = Select(t=w153, s=w154, f=w151) -> (s? t:f=w152:u32)
          n63 = call-dynamic "Write AcquisitionA.vi"("error in (no error)"=w169, "Acquisition.lvclass"=w171, "S4ACS_GUI in"=w170) -> ("error out"=w166:errorcluster, "S4ACS_GUI out"=w160:refnum<class "S4GUI.lvclass">)  [unwired: 7 in]
          n64 = Bundle By Name(cluster=w160, "Obs_state"=w152) -> (w159:refnum<class "S4GUI.lvclass">)
        }
        frame 200 {
          # "Seleção do MODO DE OPERAÇÃO (configurar ASEL, CALW, WPSEL e WPROT): \nFotometria; Polarimetria Linear; Polarimetria Circular; Eficiencia de Polar. Linear; Eficiencia de Polar. Circular;\nPolarizacao Linear Instrumental e POolarização Circular Instrumental."
          n65 = call "Read Instrument.lvclass.vi"("error in (no error)"=w233, "S4ACS_GUI in"=w234) -> ("error out"=w237:errorcluster, "Instrument.lvclass"=w197:refnum<class "Instrument.lvclass">, "S4ACS_GUI out"=w235:refnum<class "S4GUI.lvclass">)  [unwired: 7 in]
          n66 = call "Read ASEL.vi"("error in (no error)"=w237, "Instrument in"=w197) -> ("error out"=w226:errorcluster, "Opt_Selector.lvclass"=w225:refnum<class "Opt_Selector.lvclass">, "Instrument out"=w236:refnum<class "Instrument.lvclass">)  [unwired: 7 in]
          n67 = call-dynamic "Read State Machine.vi"("error in (no error)"=w226, "Device in"=w225) -> ("error out"=w229:errorcluster, "State Machine.lvclass"=w231:refnum<class "State Machine.lvclass">, "Device out"=w223:refnum<class "Opt_Selector.lvclass">)  [unwired: 7 in]
          n68 = call "Next State.vi"("error in (no error)"=w229, "New_State"=1, "State Machine in"=w231) -> ("error out"=w228:errorcluster, "State Machine out"=w227:refnum<class "State Machine.lvclass">)  [unwired: 7 in]
          n69 = call-dynamic "Write State Machine.vi"("error in (no error)"=w228, "State Machine.lvclass"=w227, "Device in"=w223) -> ("error out"=w222:errorcluster, "Device out"=w224:refnum<class "Opt_Selector.lvclass">)  [unwired: 7 in]
          n70 = Increment(x=w220) -> (x+1=w219:u32)
          n71 = call "Write ASEL.vi"("error in (no error)"=w222, "Opt_Selector.lvclass"=w224, "Instrument in"=w236) -> ("error out"=w178:errorcluster, "Instrument out"=w196:refnum<class "Instrument.lvclass">)  [unwired: 7 in]
          n72 = call "Read CALW.vi"("error in (no error)"=w178, "Instrument in"=w196) -> ("error out"=w213:errorcluster, "Opt_Selector.lvclass"=w214:refnum<class "Opt_Selector.lvclass">, "Instrument out"=w195:refnum<class "Instrument.lvclass">)  [unwired: 7 in]
          n73 = call-dynamic "Read State Machine.vi"("error in (no error)"=w213, "Device in"=w214) -> ("error out"=w210:errorcluster, "State Machine.lvclass"=w208:refnum<class "State Machine.lvclass">, "Device out"=w216:refnum<class "Opt_Selector.lvclass">)  [unwired: 7 in]
          n74 = call "Next State.vi"("error in (no error)"=w210, "New_State"=1, "State Machine in"=w208) -> ("error out"=w211:errorcluster, "State Machine out"=w212:refnum<class "State Machine.lvclass">)  [unwired: 7 in]
          n75 = call-dynamic "Write State Machine.vi"("error in (no error)"=w211, "State Machine.lvclass"=w212, "Device in"=w216) -> ("error out"=w217:errorcluster, "Device out"=w215:refnum<class "Opt_Selector.lvclass">)  [unwired: 7 in]
          n76 = call "Write CALW.vi"("error in (no error)"=w217, "Opt_Selector.lvclass"=w215, "Instrument in"=w195) -> ("error out"=w177:errorcluster, "Instrument out"=w194:refnum<class "Instrument.lvclass">)  [unwired: 7 in]
          n77 = call "Read WPSEL.vi"("error in (no error)"=w177, "Instrument in"=w194) -> ("error out"=w202:errorcluster, "Opt_Selector.lvclass"=w201:refnum<class "Opt_Selector.lvclass">, "Instrument out"=w193:refnum<class "Instrument.lvclass">)  [unwired: 7 in]
          n78 = call-dynamic "Read State Machine.vi"("error in (no error)"=w202, "Device in"=w201) -> ("error out"=w205:errorcluster, "State Machine.lvclass"=w207:refnum<class "State Machine.lvclass">, "Device out"=w199:refnum<class "Opt_Selector.lvclass">)  [unwired: 7 in]
          n79 = call "Next State.vi"("error in (no error)"=w205, "New_State"=1, "State Machine in"=w207) -> ("error out"=w204:errorcluster, "State Machine out"=w203:refnum<class "State Machine.lvclass">)  [unwired: 7 in]
          n80 = call-dynamic "Write State Machine.vi"("error in (no error)"=w204, "State Machine.lvclass"=w203, "Device in"=w199) -> ("error out"=w198:errorcluster, "Device out"=w200:refnum<class "Opt_Selector.lvclass">)  [unwired: 7 in]
          n81 = call "Write WPSEL.vi"("error in (no error)"=w198, "Opt_Selector.lvclass"=w200, "Instrument in"=w193) -> ("error out"=w176:errorcluster, "Instrument out"=w182:refnum<class "Instrument.lvclass">)  [unwired: 7 in]
          n82 = call "Read WPROT.vi"("error in (no error)"=w176, "Instrument in"=w182) -> ("error out"=w188:errorcluster, "Opt_Selector.lvclass"=w189:refnum<class "Opt_Selector.lvclass">, "Instrument out"=w181:refnum<class "Instrument.lvclass">)  [unwired: 7 in]
          n83 = call-dynamic "Read State Machine.vi"("error in (no error)"=w188, "Device in"=w189) -> ("error out"=w185:errorcluster, "State Machine.lvclass"=w183:refnum<class "State Machine.lvclass">, "Device out"=w191:refnum<class "Opt_Selector.lvclass">)  [unwired: 7 in]
          n84 = call "Next State.vi"("error in (no error)"=w185, "New_State"=1, "State Machine in"=w183) -> ("error out"=w186:errorcluster, "State Machine out"=w187:refnum<class "State Machine.lvclass">)  [unwired: 7 in]
          n85 = call-dynamic "Write State Machine.vi"("error in (no error)"=w186, "State Machine.lvclass"=w187, "Device in"=w191) -> ("error out"=w192:errorcluster, "Device out"=w190:refnum<class "Opt_Selector.lvclass">)  [unwired: 7 in]
          n86 = call "Write WPROT.vi"("error in (no error)"=w192, "Opt_Selector.lvclass"=w190, "Instrument in"=w181) -> ("error out"=w179:errorcluster, "Instrument out"=w180:refnum<class "Instrument.lvclass">)  [unwired: 7 in]
          n87 = call "Write Instrument.lvclass.vi"("error in (no error)"=w179, "Instrument.lvclass"=w180, "S4ACS_GUI in"=w235) -> ("error out"=w232:errorcluster, "S4ACS_GUI out"=w221:refnum<class "S4GUI.lvclass">)  [unwired: 7 in]
          n88 = Bundle By Name(cluster=w221, "Obs_state"=w219) -> (w218:refnum<class "S4GUI.lvclass">)
        }
        frame 201 {
          # "Espera terminar a execução dos comandos ."
          n89 = call "Read Instrument.lvclass.vi"("error in (no error)"=w301, "S4ACS_GUI in"=w302) -> ("error out"=w305:errorcluster, "Instrument.lvclass"=w306:refnum<class "Instrument.lvclass">, "S4ACS_GUI out"=w303:refnum<class "S4GUI.lvclass">)  [unwired: 7 in]
          n90 = call "Read ASEL.vi"("error in (no error)"=w305, "Instrument in"=w306) -> ("error out"=w295:errorcluster, "Opt_Selector.lvclass"=w294:refnum<class "Opt_Selector.lvclass">, "Instrument out"=w304:refnum<class "Instrument.lvclass">)  [unwired: 7 in]
          n91 = call-dynamic "Read State Machine.vi"("error in (no error)"=w295, "Device in"=w294) -> ("error out"=w298:errorcluster, "State Machine.lvclass"=w299:refnum<class "State Machine.lvclass">, "Device out"=w292:refnum<class "Opt_Selector.lvclass">)  [unwired: 7 in]
          n92 = call-dynamic "Read State.vi"("error in (no error)"=w298, "State Machine in"=w299) -> ("error out"=w297:errorcluster, "State"=w288:i32, "State Machine out"=w296:refnum<class "State Machine.lvclass">)  [unwired: 7 in]
          n93 = Equal To 0?(x=w288) -> (x = 0?=w283:bool)
          n94 = call-dynamic "Write State Machine.vi"("error in (no error)"=w297, "State Machine.lvclass"=w296, "Device in"=w292) -> ("error out"=w291:errorcluster, "Device out"=w293:refnum<class "Opt_Selector.lvclass">)  [unwired: 7 in]
          n95 = call "Write ASEL.vi"("error in (no error)"=w291, "Opt_Selector.lvclass"=w293, "Instrument in"=w304) -> ("error out"=w245:errorcluster, "Instrument out"=w246:refnum<class "Instrument.lvclass">)  [unwired: 7 in]
          n96 = call "Read CALW.vi"("error in (no error)"=w245, "Instrument in"=w246) -> ("error out"=w278:errorcluster, "Opt_Selector.lvclass"=w279:refnum<class "Opt_Selector.lvclass">, "Instrument out"=w249:refnum<class "Instrument.lvclass">)  [unwired: 7 in]
          n97 = call-dynamic "Read State Machine.vi"("error in (no error)"=w278, "Device in"=w279) -> ("error out"=w275:errorcluster, "State Machine.lvclass"=w274:refnum<class "State Machine.lvclass">, "Device out"=w281:refnum<class "Opt_Selector.lvclass">)  [unwired: 7 in]
          n98 = call-dynamic "Read State.vi"("error in (no error)"=w275, "State Machine in"=w274) -> ("error out"=w276:errorcluster, "State"=w273:i32, "State Machine out"=w277:refnum<class "State Machine.lvclass">)  [unwired: 7 in]
          n99 = Equal To 0?(x=w273) -> (x = 0?=w272:bool)
          n100 = call-dynamic "Write State Machine.vi"("error in (no error)"=w276, "State Machine.lvclass"=w277, "Device in"=w281) -> ("error out"=w282:errorcluster, "Device out"=w280:refnum<class "Opt_Selector.lvclass">)  [unwired: 7 in]
          n101 = call "Write CALW.vi"("error in (no error)"=w282, "Opt_Selector.lvclass"=w280, "Instrument in"=w249) -> ("error out"=w243:errorcluster, "Instrument out"=w244:refnum<class "Instrument.lvclass">)  [unwired: 7 in]
          n102 = call "Read WPSEL.vi"("error in (no error)"=w243, "Instrument in"=w244) -> ("error out"=w266:errorcluster, "Opt_Selector.lvclass"=w265:refnum<class "Opt_Selector.lvclass">, "Instrument out"=w248:refnum<class "Instrument.lvclass">)  [unwired: 7 in]
          n103 = call-dynamic "Read State Machine.vi"("error in (no error)"=w266, "Device in"=w265) -> ("error out"=w269:errorcluster, "State Machine.lvclass"=w270:refnum<class "State Machine.lvclass">, "Device out"=w263:refnum<class "Opt_Selector.lvclass">)  [unwired: 7 in]
          n104 = call-dynamic "Read State.vi"("error in (no error)"=w269, "State Machine in"=w270) -> ("error out"=w268:errorcluster, "State"=w271:i32, "State Machine out"=w267:refnum<class "State Machine.lvclass">)  [unwired: 7 in]
          n105 = Equal To 0?(x=w271) -> (x = 0?=w251:bool)
          n106 = call-dynamic "Write State Machine.vi"("error in (no error)"=w268, "State Machine.lvclass"=w267, "Device in"=w263) -> ("error out"=w262:errorcluster, "Device out"=w264:refnum<class "Opt_Selector.lvclass">)  [unwired: 7 in]
          n107 = call "Write WPSEL.vi"("error in (no error)"=w262, "Opt_Selector.lvclass"=w264, "Instrument in"=w248) -> ("error out"=w241:errorcluster, "Instrument out"=w242:refnum<class "Instrument.lvclass">)  [unwired: 7 in]
          n108 = call "Read WPROT.vi"("error in (no error)"=w241, "Instrument in"=w242) -> ("error out"=w257:errorcluster, "Opt_Selector.lvclass"=w258:refnum<class "Opt_Selector.lvclass">, "Instrument out"=w247:refnum<class "Instrument.lvclass">)  [unwired: 7 in]
          n109 = call-dynamic "Read State Machine.vi"("error in (no error)"=w257, "Device in"=w258) -> ("error out"=w254:errorcluster, "State Machine.lvclass"=w253:refnum<class "State Machine.lvclass">, "Device out"=w260:refnum<class "Opt_Selector.lvclass">)  [unwired: 7 in]
          n110 = call-dynamic "Read State.vi"("error in (no error)"=w254, "State Machine in"=w253) -> ("error out"=w255:errorcluster, "State"=w252:i32, "State Machine out"=w256:refnum<class "State Machine.lvclass">)  [unwired: 7 in]
          n111 = Equal To 0?(x=w252) -> (x = 0?=w250:bool)
          n112 = call-dynamic "Write State Machine.vi"("error in (no error)"=w255, "State Machine.lvclass"=w256, "Device in"=w260) -> ("error out"=w261:errorcluster, "Device out"=w259:refnum<class "Opt_Selector.lvclass">)  [unwired: 7 in]
          n113 = call "Write WPROT.vi"("error in (no error)"=w261, "Opt_Selector.lvclass"=w259, "Instrument in"=w247) -> ("error out"=w239:errorcluster, "Instrument out"=w240:refnum<class "Instrument.lvclass">)  [unwired: 7 in]
          n114 = Compound Arithmetic op=AND(w283, w272, w251, w250) -> (w285:bool)
          n115 = Select(t=u32 0, s=w285, f=w284) -> (s? t:f=w287:u32)
          n116 = call "Write Instrument.lvclass.vi"("error in (no error)"=w239, "Instrument.lvclass"=w240, "S4ACS_GUI in"=w303) -> ("error out"=w300:errorcluster, "S4ACS_GUI out"=w290:refnum<class "S4GUI.lvclass">)  [unwired: 7 in]
          n117 = Bundle By Name(cluster=w290, "Obs_state"=w287) -> (w289:refnum<class "S4GUI.lvclass">)
        }
        frame 202 {
          # "Dispara o comando para o dispositivo corrente."
          n118 = call "Read Instrument.lvclass.vi"("error in (no error)"=w323, "S4ACS_GUI in"=w324) -> ("error out"=w329:errorcluster, "Instrument.lvclass"=w330:refnum<class "Instrument.lvclass">, "S4ACS_GUI out"=w326:refnum<class "S4GUI.lvclass">)  [unwired: 7 in]
          n119 = call "Read CALW.vi"("error in (no error)"=w329, "Instrument in"=w330) -> ("error out"=w316:errorcluster, "Opt_Selector.lvclass"=w315:refnum<class "Opt_Selector.lvclass">, "Instrument out"=w328:refnum<class "Instrument.lvclass">)  [unwired: 7 in]
          n120 = call-dynamic "Read State Machine.vi"("error in (no error)"=w316, "Device in"=w315) -> ("error out"=w319:errorcluster, "State Machine.lvclass"=w321:refnum<class "State Machine.lvclass">, "Device out"=w313:refnum<class "Opt_Selector.lvclass">)  [unwired: 7 in]
          n121 = call "Next State.vi"("error in (no error)"=w319, "New_State"=1, "State Machine in"=w321) -> ("error out"=w318:errorcluster, "State Machine out"=w317:refnum<class "State Machine.lvclass">)  [unwired: 7 in]
          n122 = call-dynamic "Write State Machine.vi"("error in (no error)"=w318, "State Machine.lvclass"=w317, "Device in"=w313) -> ("error out"=w312:errorcluster, "Device out"=w314:refnum<class "Opt_Selector.lvclass">)  [unwired: 7 in]
          n123 = Increment(x=w310) -> (x+1=w309:u32)
          n124 = call "Write CALW.vi"("error in (no error)"=w312, "Opt_Selector.lvclass"=w314, "Instrument in"=w328) -> ("error out"=w325:errorcluster, "Instrument out"=w327:refnum<class "Instrument.lvclass">)  [unwired: 7 in]
          n125 = call "Write Instrument.lvclass.vi"("error in (no error)"=w325, "Instrument.lvclass"=w327, "S4ACS_GUI in"=w326) -> ("error out"=w322:errorcluster, "S4ACS_GUI out"=w311:refnum<class "S4GUI.lvclass">)  [unwired: 7 in]
          n126 = Bundle By Name(cluster=w311, "Obs_state"=w309) -> (w308:refnum<class "S4GUI.lvclass">)
        }
        frame 203 {
          # "Espera terminar a execução do comando atual \nantes de ir ao proximo passo da Observação."
          n127 = call "Read Instrument.lvclass.vi"("error in (no error)"=w349, "S4ACS_GUI in"=w350) -> ("error out"=w355:errorcluster, "Instrument.lvclass"=w356:refnum<class "Instrument.lvclass">, "S4ACS_GUI out"=w352:refnum<class "S4GUI.lvclass">)  [unwired: 7 in]
          n128 = call "Read CALW.vi"("error in (no error)"=w355, "Instrument in"=w356) -> ("error out"=w343:errorcluster, "Opt_Selector.lvclass"=w342:refnum<class "Opt_Selector.lvclass">, "Instrument out"=w354:refnum<class "Instrument.lvclass">)  [unwired: 7 in]
          n129 = call-dynamic "Read State Machine.vi"("error in (no error)"=w343, "Device in"=w342) -> ("error out"=w346:errorcluster, "State Machine.lvclass"=w347:refnum<class "State Machine.lvclass">, "Device out"=w340:refnum<class "Opt_Selector.lvclass">)  [unwired: 7 in]
          n130 = Increment(x=w333) -> (x+1=w332:u32)
          n131 = call-dynamic "Read State.vi"("error in (no error)"=w346, "State Machine in"=w347) -> ("error out"=w345:errorcluster, "State"=w335:i32, "State Machine out"=w344:refnum<class "State Machine.lvclass">)  [unwired: 7 in]
          n132 = Equal To 0?(x=w335) -> (x = 0?=w336:bool)
          n133 = call-dynamic "Write State Machine.vi"("error in (no error)"=w345, "State Machine.lvclass"=w344, "Device in"=w340) -> ("error out"=w339:errorcluster, "Device out"=w341:refnum<class "Opt_Selector.lvclass">)  [unwired: 7 in]
          n134 = call "Write CALW.vi"("error in (no error)"=w339, "Opt_Selector.lvclass"=w341, "Instrument in"=w354) -> ("error out"=w351:errorcluster, "Instrument out"=w353:refnum<class "Instrument.lvclass">)  [unwired: 7 in]
          n135 = Select(t=w332, s=w336, f=w333) -> (s? t:f=w334:u32)
          n136 = call "Write Instrument.lvclass.vi"("error in (no error)"=w351, "Instrument.lvclass"=w353, "S4ACS_GUI in"=w352) -> ("error out"=w348:errorcluster, "S4ACS_GUI out"=w338:refnum<class "S4GUI.lvclass">)  [unwired: 7 in]
          n137 = Bundle By Name(cluster=w338, "Obs_state"=w334) -> (w337:refnum<class "S4GUI.lvclass">)
        }
        frame 204 {
          # "Dispara o comando para o dispositivo corrente."
          n138 = call "Read Instrument.lvclass.vi"("error in (no error)"=w373, "S4ACS_GUI in"=w374) -> ("error out"=w379:errorcluster, "Instrument.lvclass"=w380:refnum<class "Instrument.lvclass">, "S4ACS_GUI out"=w376:refnum<class "S4GUI.lvclass">)  [unwired: 7 in]
          n139 = call "Read WPSEL.vi"("error in (no error)"=w379, "Instrument in"=w380) -> ("error out"=w366:errorcluster, "Opt_Selector.lvclass"=w365:refnum<class "Opt_Selector.lvclass">, "Instrument out"=w378:refnum<class "Instrument.lvclass">)  [unwired: 7 in]
          n140 = call-dynamic "Read State Machine.vi"("error in (no error)"=w366, "Device in"=w365) -> ("error out"=w369:errorcluster, "State Machine.lvclass"=w371:refnum<class "State Machine.lvclass">, "Device out"=w363:refnum<class "Opt_Selector.lvclass">)  [unwired: 7 in]
          n141 = call "Next State.vi"("error in (no error)"=w369, "New_State"=1, "State Machine in"=w371) -> ("error out"=w368:errorcluster, "State Machine out"=w367:refnum<class "State Machine.lvclass">)  [unwired: 7 in]
          n142 = call-dynamic "Write State Machine.vi"("error in (no error)"=w368, "State Machine.lvclass"=w367, "Device in"=w363) -> ("error out"=w362:errorcluster, "Device out"=w364:refnum<class "Opt_Selector.lvclass">)  [unwired: 7 in]
          n143 = Increment(x=w360) -> (x+1=w359:u32)
          n144 = call "Write WPSEL.vi"("error in (no error)"=w362, "Opt_Selector.lvclass"=w364, "Instrument in"=w378) -> ("error out"=w375:errorcluster, "Instrument out"=w377:refnum<class "Instrument.lvclass">)  [unwired: 7 in]
          n145 = call "Write Instrument.lvclass.vi"("error in (no error)"=w375, "Instrument.lvclass"=w377, "S4ACS_GUI in"=w376) -> ("error out"=w372:errorcluster, "S4ACS_GUI out"=w361:refnum<class "S4GUI.lvclass">)  [unwired: 7 in]
          n146 = Bundle By Name(cluster=w361, "Obs_state"=w359) -> (w358:refnum<class "S4GUI.lvclass">)
        }
        frame 205 {
          # "Espera terminar a execução do comando atual \nantes de ir ao proximo passo da Observação."
          n147 = call "Read Instrument.lvclass.vi"("error in (no error)"=w399, "S4ACS_GUI in"=w400) -> ("error out"=w405:errorcluster, "Instrument.lvclass"=w406:refnum<class "Instrument.lvclass">, "S4ACS_GUI out"=w402:refnum<class "S4GUI.lvclass">)  [unwired: 7 in]
          n148 = call "Read WPSEL.vi"("error in (no error)"=w405, "Instrument in"=w406) -> ("error out"=w393:errorcluster, "Opt_Selector.lvclass"=w392:refnum<class "Opt_Selector.lvclass">, "Instrument out"=w404:refnum<class "Instrument.lvclass">)  [unwired: 7 in]
          n149 = call-dynamic "Read State Machine.vi"("error in (no error)"=w393, "Device in"=w392) -> ("error out"=w396:errorcluster, "State Machine.lvclass"=w397:refnum<class "State Machine.lvclass">, "Device out"=w390:refnum<class "Opt_Selector.lvclass">)  [unwired: 7 in]
          n150 = Increment(x=w383) -> (x+1=w382:u32)
          n151 = call-dynamic "Read State.vi"("error in (no error)"=w396, "State Machine in"=w397) -> ("error out"=w395:errorcluster, "State"=w385:i32, "State Machine out"=w394:refnum<class "State Machine.lvclass">)  [unwired: 7 in]
          n152 = Equal To 0?(x=w385) -> (x = 0?=w386:bool)
          n153 = call-dynamic "Write State Machine.vi"("error in (no error)"=w395, "State Machine.lvclass"=w394, "Device in"=w390) -> ("error out"=w389:errorcluster, "Device out"=w391:refnum<class "Opt_Selector.lvclass">)  [unwired: 7 in]
          n154 = call "Write WPSEL.vi"("error in (no error)"=w389, "Opt_Selector.lvclass"=w391, "Instrument in"=w404) -> ("error out"=w401:errorcluster, "Instrument out"=w403:refnum<class "Instrument.lvclass">)  [unwired: 7 in]
          n155 = Select(t=w382, s=w386, f=w383) -> (s? t:f=w384:u32)
          n156 = call "Write Instrument.lvclass.vi"("error in (no error)"=w401, "Instrument.lvclass"=w403, "S4ACS_GUI in"=w402) -> ("error out"=w398:errorcluster, "S4ACS_GUI out"=w388:refnum<class "S4GUI.lvclass">)  [unwired: 7 in]
          n157 = Bundle By Name(cluster=w388, "Obs_state"=w384) -> (w387:refnum<class "S4GUI.lvclass">)
        }
        frame 206 {
          # "Dispara o comando para o dispositivo corrente."
          n158 = call "Read Instrument.lvclass.vi"("error in (no error)"=w422, "S4ACS_GUI in"=w423) -> ("error out"=w428:errorcluster, "Instrument.lvclass"=w429:refnum<class "Instrument.lvclass">, "S4ACS_GUI out"=w425:refnum<class "S4GUI.lvclass">)  [unwired: 7 in]
          n159 = call "Read WPSEL.vi"("error in (no error)"=w428, "Instrument in"=w429) -> ("error out"=w416:errorcluster, "Opt_Selector.lvclass"=w417:refnum<class "Opt_Selector.lvclass">, "Instrument out"=w427:refnum<class "Instrument.lvclass">)  [unwired: 7 in]
          n160 = call "Read target name.vi"("error in (no error)"=w416, "Optics in"=w417) -> ("error out"=w410:errorcluster, "target name"=w415:string, "Optics out"=w409:refnum<class "Opt_Selector.lvclass">)  [unwired: 7 in]
          n161 = Equal?(x=w415, y="OFF") -> (x = y?=w413:bool)
          n162 = Increment(x=w419) -> (x+1=w411:u32)
          n163 = call "Write WPSEL.vi"("error in (no error)"=w410, "Opt_Selector.lvclass"=w409, "Instrument in"=w427) -> ("error out"=w424:errorcluster, "Instrument out"=w426:refnum<class "Instrument.lvclass">)  [unwired: 7 in]
          n164 = Select(t=u32 0, s=w413, f=w411) -> (s? t:f=w408:u32)
          n165 = call "Write Instrument.lvclass.vi"("error in (no error)"=w424, "Instrument.lvclass"=w426, "S4ACS_GUI in"=w425) -> ("error out"=w421:errorcluster, "S4ACS_GUI out"=w420:refnum<class "S4GUI.lvclass">)  [unwired: 7 in]
          n166 = Bundle By Name(cluster=w420, "Obs_state"=w408) -> (w418:refnum<class "S4GUI.lvclass">)
        }
        frame 207 {
          # "Dispara o comando para o dispositivo corrente."
          n167 = call "Read Instrument.lvclass.vi"("error in (no error)"=w446, "S4ACS_GUI in"=w447) -> ("error out"=w452:errorcluster, "Instrument.lvclass"=w453:refnum<class "Instrument.lvclass">, "S4ACS_GUI out"=w449:refnum<class "S4GUI.lvclass">)  [unwired: 7 in]
          n168 = call "Read WPROT.vi"("error in (no error)"=w452, "Instrument in"=w453) -> ("error out"=w439:errorcluster, "Opt_Selector.lvclass"=w438:refnum<class "Opt_Selector.lvclass">, "Instrument out"=w451:refnum<class "Instrument.lvclass">)  [unwired: 7 in]
          n169 = call-dynamic "Read State Machine.vi"("error in (no error)"=w439, "Device in"=w438) -> ("error out"=w442:errorcluster, "State Machine.lvclass"=w444:refnum<class "State Machine.lvclass">, "Device out"=w436:refnum<class "Opt_Selector.lvclass">)  [unwired: 7 in]
          n170 = call "Next State.vi"("error in (no error)"=w442, "New_State"=1, "State Machine in"=w444) -> ("error out"=w441:errorcluster, "State Machine out"=w440:refnum<class "State Machine.lvclass">)  [unwired: 7 in]
          n171 = call-dynamic "Write State Machine.vi"("error in (no error)"=w441, "State Machine.lvclass"=w440, "Device in"=w436) -> ("error out"=w435:errorcluster, "Device out"=w437:refnum<class "Opt_Selector.lvclass">)  [unwired: 7 in]
          n172 = Increment(x=w433) -> (x+1=w432:u32)
          n173 = call "Write WPROT.vi"("error in (no error)"=w435, "Opt_Selector.lvclass"=w437, "Instrument in"=w451) -> ("error out"=w448:errorcluster, "Instrument out"=w450:refnum<class "Instrument.lvclass">)  [unwired: 7 in]
          n174 = call "Write Instrument.lvclass.vi"("error in (no error)"=w448, "Instrument.lvclass"=w450, "S4ACS_GUI in"=w449) -> ("error out"=w445:errorcluster, "S4ACS_GUI out"=w434:refnum<class "S4GUI.lvclass">)  [unwired: 7 in]
          n175 = Bundle By Name(cluster=w434, "Obs_state"=w432) -> (w431:refnum<class "S4GUI.lvclass">)
        }
        frame 208 {
          # "Espera terminar a execução do comando atual \nantes de ir ao proximo passo da Observação."
          n176 = call "Read Instrument.lvclass.vi"("error in (no error)"=w472, "S4ACS_GUI in"=w473) -> ("error out"=w478:errorcluster, "Instrument.lvclass"=w479:refnum<class "Instrument.lvclass">, "S4ACS_GUI out"=w475:refnum<class "S4GUI.lvclass">)  [unwired: 7 in]
          n177 = call "Read WPROT.vi"("error in (no error)"=w478, "Instrument in"=w479) -> ("error out"=w466:errorcluster, "Opt_Selector.lvclass"=w465:refnum<class "Opt_Selector.lvclass">, "Instrument out"=w477:refnum<class "Instrument.lvclass">)  [unwired: 7 in]
          n178 = call-dynamic "Read State Machine.vi"("error in (no error)"=w466, "Device in"=w465) -> ("error out"=w469:errorcluster, "State Machine.lvclass"=w470:refnum<class "State Machine.lvclass">, "Device out"=w463:refnum<class "Opt_Selector.lvclass">)  [unwired: 7 in]
          n179 = call-dynamic "Read State.vi"("error in (no error)"=w469, "State Machine in"=w470) -> ("error out"=w468:errorcluster, "State"=w458:i32, "State Machine out"=w467:refnum<class "State Machine.lvclass">)  [unwired: 7 in]
          n180 = Equal To 0?(x=w458) -> (x = 0?=w459:bool)
          n181 = call-dynamic "Write State Machine.vi"("error in (no error)"=w468, "State Machine.lvclass"=w467, "Device in"=w463) -> ("error out"=w462:errorcluster, "Device out"=w464:refnum<class "Opt_Selector.lvclass">)  [unwired: 7 in]
          n182 = call "Write WPSEL.vi"("error in (no error)"=w462, "Opt_Selector.lvclass"=w464, "Instrument in"=w477) -> ("error out"=w474:errorcluster, "Instrument out"=w476:refnum<class "Instrument.lvclass">)  [unwired: 7 in]
          n183 = Select(t=u32 0, s=w459, f=w456) -> (s? t:f=w457:u32)
          n184 = call "Write Instrument.lvclass.vi"("error in (no error)"=w474, "Instrument.lvclass"=w476, "S4ACS_GUI in"=w475) -> ("error out"=w471:errorcluster, "S4ACS_GUI out"=w461:refnum<class "S4GUI.lvclass">)  [unwired: 7 in]
          n185 = Bundle By Name(cluster=w461, "Obs_state"=w457) -> (w460:refnum<class "S4GUI.lvclass">)
        }
        frame 240 {
          # "Carrega mensagem de \"Invalid temperature\" (botão SET da aba \"CCD temp\" de cada canal) e desvia para estado de erro (Acq_state=1)"
          n186 = Bundle By Name(cluster=w482, "Error Msg"="ERROR Invalid temperature - input value lower than minimum for current CCD setup (state 240). " ("f")) -> (w483:refnum<class "S4GUI.lvclass">)
          n187 = call-dynamic "Write Acq_state.vi"("error in (no error)"=w484, "Acq_state"=u32 1, "Acquisition in"=w487) -> ("error out"=w485:errorcluster, "Acquisition out"=w486:refnum<class "Acquisition.lvclass">)  [unwired: 7 in]
        }
        frame 251 {
          # "Verifica se ha funcao valida de instrumento:"
          n188 = flat-sequence {
            tunnel: [w534] -> w490
            tunnel: w500 -> [w534]
            frame #0 {
              n189 = Tick Count (ms)() -> (millisecond timer value=→"time3":u32)
            }
          }
          n190 = Unbundle By Name(w492) -> ("Instrument.lvclass"=w496:refnum<class "Instrument.lvclass">)
          n191 = call-dynamic "Load Function.vi"("error in (no error)"=w490, "Instrument in"=w496) -> ("error out"=w493:errorcluster, "Instrument out"=w495:refnum<class "Instrument.lvclass">)  [unwired: 8 in]
          n192 = call-dynamic "Read Function.vi"("error in (no error)"=w493, "Instrument in"=w495) -> ("error out"=w489:errorcluster, "Function"=w488:enum16{"PHOTO", "POLAR", "NONE"}, "Instrument out"=w494:refnum<class "Instrument.lvclass">)  [unwired: 7 in]
          n193 = Bundle By Name(cluster=w492, "Instrument.lvclass"=w494) -> (w491:refnum<class "S4GUI.lvclass">)
          n194 = case shown="\"NONE\"" w488 {
            tunnel: w507 -> [_ w525]
            tunnel: w506 -> [w511 w517]
            tunnel: [u32 1 w516] -> w505
            tunnel: [w511 w515] -> w504
            tunnel: [w509 w514] -> w502
            tunnel: w489 -> [w509 w513]
            tunnel: ["ERROR: No instrument function set (neither POLARIMETRICS nor PHOTOMETRICS )" ("Error Msg") "" ("Error Msg")] -> w499
            frame "NONE" {
            }
            frame Default {
              # "configura o canal,\nmas não dispara\na exposicao."
              # "Dispara o comando para o dispositivo corrente."
              n195 = call-dynamic "Read Channel.vi"("error in (no error)"=w513, "Acquisition in"=w517) -> ("error out"=w522:errorcluster, "Channel.lvclass"=w524:refnum<class "Channel.lvclass">, "Acquisition out"=w532:refnum<class "Acquisition.lvclass">)  [unwired: 7 in]
              n196 = call-dynamic "Write expose.vi"("error in (no error)"=w522, "expose"=FALSE, "Channel in"=w524) -> ("error out"=w521:errorcluster, "Channel out"=w523:refnum<class "Channel.lvclass">)  [unwired: 7 in]
              n197 = call-dynamic "Read State Machine.vi"("error in (no error)"=w521, "Device in"=w523) -> ("error out"=w529:errorcluster, "State Machine.lvclass"=w531:refnum<class "State Machine.lvclass">, "Device out"=w527:refnum<class "Channel.lvclass">)  [unwired: 7 in]
              n198 = call "Next State.vi"("error in (no error)"=w529, "New_State"=1, "State Machine in"=w531) -> ("error out"=w518:errorcluster, "State Machine out"=w519:refnum<class "State Machine.lvclass">)  [unwired: 7 in]
              n199 = call-dynamic "Write State Machine.vi"("error in (no error)"=w518, "State Machine.lvclass"=w519, "Device in"=w527) -> ("error out"=w526:errorcluster, "Device out"=w528:refnum<class "Channel.lvclass">)  [unwired: 7 in]
              n200 = call-dynamic "Write Channel.vi"("error in (no error)"=w526, "Channel.lvclass"=w528, "Acquisition in"=w532) -> ("error out"=w514:errorcluster, "Acquisition out"=w515:refnum<class "Acquisition.lvclass">)  [unwired: 7 in]
              n201 = Increment(x=w525) -> (x+1=w516:u32)
            }
          }
          n202 = Bundle By Name(cluster=w491, "Error Msg"=w499, "cyclesDone"=u32 0) -> (w498:refnum<class "S4GUI.lvclass">)
          n203 = call-dynamic "Write Acq_state.vi"("error in (no error)"=w502, "Acq_state"=w505, "Acquisition in"=w504) -> ("error out"=w501:errorcluster, "Acquisition out"=w503:refnum<class "Acquisition.lvclass">)  [unwired: 7 in]
        }
        frame 252 {
          # "Erro no Texp."
          # "Erro no setup\ninicial do ACS."
          # "Espera terminar a execução do comando atual \nantes de ir ao proximo passo da Observação."
          n204 = flat-sequence {
            tunnel: [w579] -> w547
            tunnel: w548 -> [w579]
            frame #0 {
              n205 = Tick Count (ms)() -> (millisecond timer value=→"time4":u32)
            }
          }
          n206 = call-dynamic "Read Channel.vi"("error in (no error)"=w547, "Acquisition in"=w553) -> ("error out"=w562:errorcluster, "Channel.lvclass"=w561:refnum<class "Channel.lvclass">, "Acquisition out"=w563:refnum<class "Acquisition.lvclass">)  [unwired: 7 in]
          n207 = call-dynamic "Read State Machine.vi"("error in (no error)"=w562, "Device in"=w561) -> ("error out"=w555:errorcluster, "State Machine.lvclass"=w557:refnum<class "State Machine.lvclass">, "Device out"=w559:refnum<class "Channel.lvclass">)  [unwired: 7 in]
          n208 = call-dynamic "Read State.vi"("error in (no error)"=w555, "State Machine in"=w557) -> ("error out"=w554:errorcluster, "State"=w545:i32, "State Machine out"=w556:refnum<class "State Machine.lvclass">)  [unwired: 7 in]
          n209 = Equal To 0?(x=w545) -> (x = 0?=w543:bool)
          n210 = call-dynamic "Write State Machine.vi"("error in (no error)"=w554, "State Machine.lvclass"=w556, "Device in"=w559) -> ("error out"=w558:errorcluster, "Device out"=w560:refnum<class "Channel.lvclass">)  [unwired: 7 in]
          n211 = Equal?(x=28, y=w545) -> (x = y?=w542:bool)
          n212 = Equal?(x=38, y=w545) -> (x = y?=w541:bool)
          n213 = call-dynamic "Write Channel.vi"("error in (no error)"=w558, "Channel.lvclass"=w560, "Acquisition in"=w563) -> ("error out"=w552:errorcluster, "Acquisition out"=w551:refnum<class "Acquisition.lvclass">)  [unwired: 7 in]
          n214 = Build Array(w543, w542, w541) -> (w540:bool[])
          n215 = Boolean Array To Number(Boolean array=w540) -> (number=w539:u32)
          n216 = case shown="0, Default" w539 {
            tunnel: w538 -> [w565 _ _ _]
            tunnel: [w565 u32 300 ("t") u32 1 ("t") u32 1 ("t")] -> w537
            tunnel: w536 -> [w564 w568 w573 w577]
            tunnel: [w564 w567 w572 w576] -> w535
            frame 0, Default {
            }
            frame 1 {
              n217 = Tick Count (ms)() -> (millisecond timer value=→"time307":u32)
              n218 = Bundle By Name(cluster=w568, "Error Msg"="") -> (w567:refnum<class "S4GUI.lvclass">)
            }
            frame 2 {
              n219 = Bundle By Name(cluster=w573, "Error Msg"="ERROR: Some channel initialization failed. S4GUI:HandleObservationAsync.vi state 252.") -> (w572:refnum<class "S4GUI.lvclass">)
            }
            frame 4 {
              n220 = Bundle By Name(cluster=w577, "Error Msg"="ERROR: Some channel with invalid Exposure Time. S4GUI:HandleObservationAsync.vi state 252.") -> (w576:refnum<class "S4GUI.lvclass">)
            }
          }
          n221 = call-dynamic "Write Acq_state.vi"("error in (no error)"=w552, "Acq_state"=w537, "Acquisition in"=w551) -> ("error out"=w549:errorcluster, "Acquisition out"=w550:refnum<class "Acquisition.lvclass">)  [unwired: 7 in]
        }
        frame 253 {
          # "Sem syncbox, \ntrigger mode = 0 (internal)"
          n222 = call-dynamic "Read Channel.vi"("error in (no error)"=w582, "Acquisition in"=w614) -> ("error out"=w587:errorcluster, "Channel.lvclass"=w586:refnum<class "Channel.lvclass">, "Acquisition out"=w609:refnum<class "Acquisition.lvclass">)  [unwired: 7 in]
          n223 = call-dynamic "Read Interface.vi"("error in (no error)"=w587, "Channel in"=w586) -> ("error out"=w585:errorcluster, "Interface.lvclass"=w591:refnum<class "Interface.lvclass">, "Channel out"=w590:refnum<class "Channel.lvclass">)  [unwired: 7 in]
          n224 = call-dynamic "Get CCD_Config.vi"("error in (no error)"=w585, "Interface in"=w591) -> ("error out"=w598:errorcluster, "output cluster"=w600:T1, "Interface out"=w597:refnum<class "Interface.lvclass">)  [unwired: 7 in]
          n225 = Bundle By Name(cluster=w600, "TRIGGER_MODE"=u8 0) -> (w596:T1)
          n226 = call-dynamic "Set CCD_Config.vi"("error in (no error)"=w598, "input cluster"=w596, "Interface in"=w597) -> ("error out"=w594:errorcluster, "Interface out"=w592:refnum<class "Interface.lvclass">)  [unwired: 7 in]
          n227 = Flatten To String(anything=w596, error in (no error)=w594) -> (data string=w595:string, error out=w593:errorcluster)  [unwired: 2 in, 1 out]
          n228 = call "Write flatted cluster.vi"("error in (no error)"=w593, "flatted cluster"=w595, "Interface in"=w592) -> ("error out"=w588:errorcluster, "Interface out"=w589:refnum<class "Interface.lvclass">)  [unwired: 7 in]
          n229 = call-dynamic "Write Interface.vi"("error in (no error)"=w588, "Interface.lvclass"=w589, "Channel in"=w590) -> ("error out"=w584:errorcluster, "Channel out"=w583:refnum<class "Channel.lvclass">)  [unwired: 7 in]
          n230 = call-dynamic "Read State Machine.vi"("error in (no error)"=w584, "Device in"=w583) -> ("error out"=w606:errorcluster, "State Machine.lvclass"=w608:refnum<class "State Machine.lvclass">, "Device out"=w604:refnum<class "Channel.lvclass">)  [unwired: 7 in]
          n231 = Increment(x=w611) -> (x+1=w612:u32)
          n232 = call "Next State.vi"("error in (no error)"=w606, "New_State"=60, "State Machine in"=w608) -> ("error out"=w601:errorcluster, "State Machine out"=w602:refnum<class "State Machine.lvclass">)  [unwired: 7 in]
          n233 = call-dynamic "Write State Machine.vi"("error in (no error)"=w601, "State Machine.lvclass"=w602, "Device in"=w604) -> ("error out"=w603:errorcluster, "Device out"=w605:refnum<class "Channel.lvclass">)  [unwired: 7 in]
          n234 = call-dynamic "Write Channel.vi"("error in (no error)"=w603, "Channel.lvclass"=w605, "Acquisition in"=w609) -> ("error out"=w610:errorcluster, "Acquisition out"=w613:refnum<class "Acquisition.lvclass">)  [unwired: 7 in]
          n235 = call-dynamic "Write Acq_state.vi"("error in (no error)"=w610, "Acq_state"=w612, "Acquisition in"=w613) -> ("error out"=w615:errorcluster, "Acquisition out"=w616:refnum<class "Acquisition.lvclass">)  [unwired: 7 in]
        }
        frame 254 {
          # "Espera terminar a execução do comando atual \nantes de ir ao proximo passo da Observação."
          n236 = call-dynamic "Read Channel.vi"("error in (no error)"=w619, "Acquisition in"=w626) -> ("error out"=w637:errorcluster, "Channel.lvclass"=w636:refnum<class "Channel.lvclass">, "Acquisition out"=w638:refnum<class "Acquisition.lvclass">)  [unwired: 7 in]
          n237 = call-dynamic "Read State Machine.vi"("error in (no error)"=w637, "Device in"=w636) -> ("error out"=w630:errorcluster, "State Machine.lvclass"=w632:refnum<class "State Machine.lvclass">, "Device out"=w634:refnum<class "Channel.lvclass">)  [unwired: 7 in]
          n238 = call-dynamic "Read State.vi"("error in (no error)"=w630, "State Machine in"=w632) -> ("error out"=w629:errorcluster, "State"=w627:i32, "State Machine out"=w631:refnum<class "State Machine.lvclass">)  [unwired: 7 in]
          n239 = Equal To 0?(x=w627) -> (x = 0?=w628:bool)
          n240 = call-dynamic "Write State Machine.vi"("error in (no error)"=w629, "State Machine.lvclass"=w631, "Device in"=w634) -> ("error out"=w633:errorcluster, "Device out"=w635:refnum<class "Channel.lvclass">)  [unwired: 7 in]
          n241 = call-dynamic "Write Channel.vi"("error in (no error)"=w633, "Channel.lvclass"=w635, "Acquisition in"=w638) -> ("error out"=w623:errorcluster, "Acquisition out"=w622:refnum<class "Acquisition.lvclass">)  [unwired: 7 in]
          n242 = Select(t=u32 299, s=w628, f=w618) -> (s? t:f=w624:u32)
          n243 = call-dynamic "Write Acq_state.vi"("error in (no error)"=w623, "Acq_state"=w624, "Acquisition in"=w622) -> ("error out"=w620:errorcluster, "Acquisition out"=w621:refnum<class "Acquisition.lvclass">)  [unwired: 7 in]
        }
        frame 271 {
          # "configura o canal,\nmas não dispara\na exposicao."
          # "Dispara o comando para o dispositivo corrente."
          n244 = flat-sequence {
            tunnel: [w670] -> w647
            tunnel: w648 -> [w670]
            frame #0 {
              n245 = Tick Count (ms)() -> (millisecond timer value=→"time5":u32)
            }
          }
          n246 = call-dynamic "Read Channel.vi"("error in (no error)"=w647, "Acquisition in"=w653) -> ("error out"=w658:errorcluster, "Channel.lvclass"=w660:refnum<class "Channel.lvclass">, "Acquisition out"=w668:refnum<class "Acquisition.lvclass">)  [unwired: 7 in]
          n247 = call-dynamic "Write expose.vi"("error in (no error)"=w658, "expose"=FALSE, "Channel in"=w660) -> ("error out"=w657:errorcluster, "Channel out"=w659:refnum<class "Channel.lvclass">)  [unwired: 7 in]
          n248 = call-dynamic "Read State Machine.vi"("error in (no error)"=w657, "Device in"=w659) -> ("error out"=w665:errorcluster, "State Machine.lvclass"=w667:refnum<class "State Machine.lvclass">, "Device out"=w663:refnum<class "Channel.lvclass">)  [unwired: 7 in]
          n249 = call "Next State.vi"("error in (no error)"=w665, "New_State"=1, "State Machine in"=w667) -> ("error out"=w654:errorcluster, "State Machine out"=w655:refnum<class "State Machine.lvclass">)  [unwired: 7 in]
          n250 = call-dynamic "Write State Machine.vi"("error in (no error)"=w654, "State Machine.lvclass"=w655, "Device in"=w663) -> ("error out"=w662:errorcluster, "Device out"=w664:refnum<class "Channel.lvclass">)  [unwired: 7 in]
          n251 = call-dynamic "Write Channel.vi"("error in (no error)"=w662, "Channel.lvclass"=w664, "Acquisition in"=w668) -> ("error out"=w640:errorcluster, "Acquisition out"=w651:refnum<class "Acquisition.lvclass">)  [unwired: 7 in]
          n252 = Increment(x=w661) -> (x+1=w652:u32)
          n253 = Unbundle By Name(w642) -> ("TelFocus.lvclass"=w644:refnum<class "TelFocus.lvclass">)
          n254 = call-dynamic "Write focus #stepsdone.vi"("error in (no error)"=w640, "focus #stepsdone"=u32 0, "TelFocus in"=w644) -> ("error out"=w639:errorcluster, "TelFocus out"=w641:refnum<class "TelFocus.lvclass">)  [unwired: 7 in]
          n255 = Bundle By Name(cluster=w642, "TelFocus.lvclass"=w641, "Error Msg"="") -> (w645:refnum<class "S4GUI.lvclass">)
          n256 = call-dynamic "Write Acq_state.vi"("error in (no error)"=w639, "Acq_state"=w652, "Acquisition in"=w651) -> ("error out"=w649:errorcluster, "Acquisition out"=w650:refnum<class "Acquisition.lvclass">)  [unwired: 7 in]
        }
        frame 272 {
          # "Erro no Texp."
          # "Erro no setup\ninicial do ACS."
          # "Espera terminar a execução do comando atual \nantes de ir ao proximo passo da Observação."
          n257 = flat-sequence {
            tunnel: [w714] -> w683
            tunnel: w684 -> [w714]
            frame #0 {
              n258 = Tick Count (ms)() -> (millisecond timer value=→"time6":u32)
            }
          }
          n259 = call-dynamic "Read Channel.vi"("error in (no error)"=w683, "Acquisition in"=w689) -> ("error out"=w698:errorcluster, "Channel.lvclass"=w697:refnum<class "Channel.lvclass">, "Acquisition out"=w699:refnum<class "Acquisition.lvclass">)  [unwired: 7 in]
          n260 = call-dynamic "Read State Machine.vi"("error in (no error)"=w698, "Device in"=w697) -> ("error out"=w691:errorcluster, "State Machine.lvclass"=w693:refnum<class "State Machine.lvclass">, "Device out"=w695:refnum<class "Channel.lvclass">)  [unwired: 7 in]
          n261 = call-dynamic "Read State.vi"("error in (no error)"=w691, "State Machine in"=w693) -> ("error out"=w690:errorcluster, "State"=w681:i32, "State Machine out"=w692:refnum<class "State Machine.lvclass">)  [unwired: 7 in]
          n262 = Equal To 0?(x=w681) -> (x = 0?=w679:bool)
          n263 = call-dynamic "Write State Machine.vi"("error in (no error)"=w690, "State Machine.lvclass"=w692, "Device in"=w695) -> ("error out"=w694:errorcluster, "Device out"=w696:refnum<class "Channel.lvclass">)  [unwired: 7 in]
          n264 = Equal?(x=28, y=w681) -> (x = y?=w678:bool)
          n265 = Equal?(x=38, y=w681) -> (x = y?=w677:bool)
          n266 = call-dynamic "Write Channel.vi"("error in (no error)"=w694, "Channel.lvclass"=w696, "Acquisition in"=w699) -> ("error out"=w688:errorcluster, "Acquisition out"=w687:refnum<class "Acquisition.lvclass">)  [unwired: 7 in]
          n267 = Build Array(w679, w678, w677) -> (w676:bool[])
          n268 = Boolean Array To Number(Boolean array=w676) -> (number=w675:u32)
          n269 = case shown="0, Default" w675 {
            tunnel: w674 -> [w700 _ _ _]
            tunnel: [w700 u32 360 ("t") u32 0 ("t") u32 0 ("t")] -> w673
            tunnel: w672 -> [w701 w703 w708 w712]
            tunnel: [w701 w702 w707 w711] -> w671
            frame 0, Default {
            }
            frame 1 {
              n270 = Bundle By Name(cluster=w703, "Error Msg"="") -> (w702:refnum<class "S4GUI.lvclass">)
            }
            frame 2 {
              n271 = Bundle By Name(cluster=w708, "Error Msg"="ERROR: Some channel initialization failed. S4GUI:HandleObservationAsync.vi state 272.") -> (w707:refnum<class "S4GUI.lvclass">)
            }
            frame 4 {
              n272 = Bundle By Name(cluster=w712, "Error Msg"="ERROR: Some channel with invalid Exposition Time. S4GUI:HandleObservationAsync.vi state 272.") -> (w711:refnum<class "S4GUI.lvclass">)
            }
          }
          n273 = call-dynamic "Write Acq_state.vi"("error in (no error)"=w688, "Acq_state"=w673, "Acquisition in"=w687) -> ("error out"=w685:errorcluster, "Acquisition out"=w686:refnum<class "Acquisition.lvclass">)  [unwired: 7 in]
        }
        frame 300 {
          # "Verifica se é modo fotometria ou polarimetria:\nTrue = polarimetria (estado 301)\nFalse = fotometria (estado 321)"
          n274 = flat-sequence {
            tunnel: [w742] -> w731
            tunnel: w732 -> [w742]
            frame #0 {
              n275 = local read "time4"() -> (w744:u32)
              n276 = local read "time3"() -> (w743:u32)
              n277 = Subtract(x=w744, y=w743) -> (x-y=→"delay 3-4":u32)
            }
          }
          n278 = call "Read Instrument.lvclass.vi"("error in (no error)"=w731, "S4ACS_GUI in"=w741) -> ("error out"=w738:errorcluster, "Instrument.lvclass"=w739:refnum<class "Instrument.lvclass">, "S4ACS_GUI out"=w728:refnum<class "S4GUI.lvclass">)  [unwired: 7 in]
          n279 = call-dynamic "Read mode.vi"("error in (no error)"=w738, "Instrument in"=w739) -> ("error out"=w718:errorcluster, "mode"=w737:bool)  [unwired: 7 in, 1 out]
          n280 = call-dynamic "Read Channel.vi"("error in (no error)"=w718, "Acquisition in"=w726) -> ("error out"=w720:errorcluster, "Channel.lvclass"=w722:refnum<class "Channel.lvclass">, "Acquisition out"=w725:refnum<class "Acquisition.lvclass">)  [unwired: 7 in]
          n281 = call-dynamic "Write PrevCyclesDone.vi"("error in (no error)"=w720, "PrevCyclesDone"=u32 0, "Channel in"=w722) -> ("error out"=w719:errorcluster, "Channel out"=w721:refnum<class "Channel.lvclass">)  [unwired: 7 in]
          n282 = call-dynamic "Write Channel.vi"("error in (no error)"=w719, "Channel.lvclass"=w721, "Acquisition in"=w725) -> ("error out"=w717:errorcluster, "Acquisition out"=w724:refnum<class "Acquisition.lvclass">)  [unwired: 7 in]
          n283 = Select(t=u32 301, s=w737, f=u32 321 ("t")) -> (s? t:f=w735:u32)
          n284 = call-dynamic "Write Acq_state.vi"("error in (no error)"=w717, "Acq_state"=w735, "Acquisition in"=w724) -> ("error out"=w734:errorcluster, "Acquisition out"=w733:refnum<class "Acquisition.lvclass">)  [unwired: 7 in]
          n285 = Bundle By Name(cluster=w728, "cyclesDone"=u32 0, "sequesDone"=u32 0, "seqAtual"=u32 0) -> (w727:refnum<class "S4GUI.lvclass">)
        }
        frame 301 {
          # "Se for polarimetria com 1 pos,\ndesabilita WAIT EXPOSE no ACS."
          # "Envia WAIT_EXPOSE_COMMAND ...\nON (se forem varias posicoes) ou\nOFF (se for uma única posição da lâmina.)"
          n286 = call-dynamic "VerifWavePlate.vi"("error in (no error)"=w750, "S4GUI in"=w751) -> ("error out"=w749:errorcluster, "One Position"=w747:bool, "S4GUI out"=w748:refnum<class "S4GUI.lvclass">)  [unwired: 7 in]
          n287 = Not(x=w747) -> (.not. x?=w746:bool)
          n288 = call-dynamic "Read Channel.vi"("error in (no error)"=w749, "Acquisition in"=w765) -> ("error out"=w753:errorcluster, "Channel.lvclass"=w755:refnum<class "Channel.lvclass">, "Acquisition out"=w773:refnum<class "Acquisition.lvclass">)  [unwired: 7 in]
          n289 = call-dynamic "Write wait_expose.vi"("error in (no error)"=w753, "wait_expose"=w746, "Channel in"=w755) -> ("error out"=w752:errorcluster, "Channel out"=w754:refnum<class "Channel.lvclass">)  [unwired: 7 in]
          n290 = call-dynamic "Read State Machine.vi"("error in (no error)"=w752, "Device in"=w754) -> ("error out"=w770:errorcluster, "State Machine.lvclass"=w772:refnum<class "State Machine.lvclass">, "Device out"=w768:refnum<class "Channel.lvclass">)  [unwired: 7 in]
          n291 = call "Next State.vi"("error in (no error)"=w770, "New_State"=40, "State Machine in"=w772) -> ("error out"=w758:errorcluster, "State Machine out"=w759:refnum<class "State Machine.lvclass">)  [unwired: 7 in]
          n292 = call-dynamic "Write State Machine.vi"("error in (no error)"=w758, "State Machine.lvclass"=w759, "Device in"=w768) -> ("error out"=w767:errorcluster, "Device out"=w769:refnum<class "Channel.lvclass">)  [unwired: 7 in]
          n293 = Increment(x=w766) -> (x+1=w764:u32)
          n294 = call-dynamic "Write Channel.vi"("error in (no error)"=w767, "Channel.lvclass"=w769, "Acquisition in"=w773) -> ("error out"=w763:errorcluster, "Acquisition out"=w762:refnum<class "Acquisition.lvclass">)  [unwired: 7 in]
          n295 = call-dynamic "Write Acq_state.vi"("error in (no error)"=w763, "Acq_state"=w764, "Acquisition in"=w762) -> ("error out"=w760:errorcluster, "Acquisition out"=w761:refnum<class "Acquisition.lvclass">)  [unwired: 7 in]
          n296 = Bundle By Name(cluster=w748, "Error Msg"="") -> (w756:refnum<class "S4GUI.lvclass">)
        }
        frame 302 {
          # "Espera canal voltar para IDLE"
          n297 = call-dynamic "Read Channel.vi"("error in (no error)"=w789, "Acquisition in"=w790) -> ("error out"=w780:errorcluster, "Channel.lvclass"=w781:refnum<class "Channel.lvclass">, "Acquisition out"=w782:refnum<class "Acquisition.lvclass">)  [unwired: 7 in]
          n298 = call-dynamic "Read State Machine.vi"("error in (no error)"=w780, "Device in"=w781) -> ("error out"=w783:errorcluster, "State Machine.lvclass"=w785:refnum<class "State Machine.lvclass">)  [unwired: 7 in, 1 out]
          n299 = call-dynamic "Read State.vi"("error in (no error)"=w783, "State Machine in"=w785) -> ("error out"=w778:errorcluster, "State"=w784:i32)  [unwired: 7 in, 1 out]
          n300 = Equal?(x=0, y=w784) -> (x = y?=w774:bool)
          n301 = Increment(x=w776) -> (x+1=w777:u32)
          n302 = Select(t=w777, s=w774, f=w776) -> (s? t:f=w779:u32)
          n303 = call-dynamic "Write Acq_state.vi"("error in (no error)"=w778, "Acq_state"=w779, "Acquisition in"=w782) -> ("error out"=w787:errorcluster, "Acquisition out"=w788:refnum<class "Acquisition.lvclass">)  [unwired: 7 in]
        }
        frame 303 {
          # "2024 04 26: ATEN敲O: NO MODO POLARIMETRIA ASYNC, APENAS 1 CANAL POR VEZ PODE FAZER AQUISI敲O!\nO atributo S4GUI:SeqAtual pode se perder se mais de um canal rodar aqui..."
          n304 = flat-sequence {
            tunnel: w805 -> [w845]
            tunnel: [w845] -> w804
            frame #0 {
              n305 = Tick Count (ms)() -> (millisecond timer value=→"time1":u32)
            }
          }
          n306 = call "Read Instrument.lvclass.vi"("error in (no error)"=w804, "S4ACS_GUI in"=w841) -> ("error out"=w843:errorcluster, "Instrument.lvclass"=w844:refnum<class "Instrument.lvclass">, "S4ACS_GUI out"=w802:refnum<class "S4GUI.lvclass">)  [unwired: 7 in]
          n307 = call "Read WPROT.vi"("error in (no error)"=w843, "Instrument in"=w844) -> ("error out"=w838:errorcluster, "Opt_Selector.lvclass"=w839:refnum<class "Opt_Selector.lvclass">, "Instrument out"=w842:refnum<class "Instrument.lvclass">)  [unwired: 7 in]
          n308 = call-dynamic "getTargetPos.vi"("error in (no error)"=w838, "Opt_Selector in"=w839) -> ("error out"=w837:errorcluster, "Target Pos"=w817:u16, "Opt_Selector out"=w836:refnum<class "Opt_Selector.lvclass">)  [unwired: 7 in]
          n309 = Build Array(-1.0 ("element"), 0.0 ("element"), 22.5 ("element"), 45.0 ("element"), 67.5 ("element"), 90.0 ("element"), 112.5 ("element"), 135.0 ("element"), 157.5 ("element"), 180.0 ("element"), 202.5 ("element"), 225.0 ("element"), 247.5 ("element"), 270.0 ("element"), 292.5 ("element"), 315.0 ("element"), 337.5 ("element")) -> (w829:dbl[])
          n310 = Unbundle By Name(w802) -> ("seqAtual"=w803:u32)
          n311 = Index Array(array=w829, index=w817) -> (element=w816:dbl)
          n312 = case shown="1..16" w817 {
            selector: w817 -> [_ w879]
            tunnel: w842 -> [w855 w867]
            tunnel: [w855 w867] -> w812
            tunnel: [w852 w866] -> w811
            tunnel: w840 -> [_ w881]
            tunnel: [u32 314 w880] -> w810
            tunnel: w837 -> [w853 w875]
            tunnel: w836 -> [w854 w874]
            tunnel: w816 -> [_ w869]
            tunnel: [w850 w868] -> w813
            tunnel: [u32 0 ("seqAtual") w857] -> w799
            tunnel: w803 -> [_ w858]
            frame 0, Default {
              # "Verifica os ciclos"
              # "Recupera a sequencia anterior para o caso \nde repetição da sequencia (sem precisar clicar \nnas posicoes desejadas novamente)."
              n313 = call-dynamic "Read sequencia_ant.vi"("error in (no error)"=w853, "Opt_Selector in"=w854) -> ("error out"=w849:errorcluster, "sequencia_ant"=w848:u16, "Opt_Selector out"=w851:refnum<class "Opt_Selector.lvclass">)  [unwired: 7 in]
              n314 = call-dynamic "Write sequencia.vi"("error in (no error)"=w849, "sequencia"=w848, "Opt_Selector in"=w851) -> ("error out"=w852:errorcluster, "Opt_Selector out"=w850:refnum<class "Opt_Selector.lvclass">)  [unwired: 7 in]
            }
            frame 1..16 {
              # "Inicia o Ticks com\nvalor do relogio atual"
              # "Espera até 40 x 0.25s (= 10s) para\nmecanismo entrar em READY"
              n315 = Number To Decimal String(number=w879) -> (decimal integer string=w878:string)  [unwired: 1 in]
              n316 = Concatenate Strings("WP" ("string"), w878) -> (w876:string)
              n317 = call "Write target name.vi"("error in (no error)"=w875, "target name"=w876, "Optics in"=w874) -> ("error out"=w872:errorcluster, "Optics out"=w873:refnum<class "Opt_Selector.lvclass">)  [unwired: 7 in]
              n318 = call "Write target.vi"("error in (no error)"=w872, "target"=w869, "Optics in"=w873) -> ("error out"=w871:errorcluster, "Optics out"=w870:refnum<class "Opt_Selector.lvclass">)  [unwired: 7 in]
              n319 = call-dynamic "Read State Machine.vi"("error in (no error)"=w871, "Device in"=w870) -> ("error out"=w883:errorcluster, "State Machine.lvclass"=w885:refnum<class "State Machine.lvclass">, "Device out"=w882:refnum<class "Opt_Selector.lvclass">)  [unwired: 7 in]
              n320 = Increment(x=w881) -> (x+1=w880:u32)
              n321 = Increment(x=w858) -> (x+1=w857:u32)
              n322 = call "Next State.vi"("error in (no error)"=w883, "New_State"=1, "State Machine in"=w885) -> ("error out"=w864:errorcluster, "State Machine out"=w865:refnum<class "State Machine.lvclass">)  [unwired: 7 in]
              n323 = call-dynamic "Write Timer.vi"("error in (no error)"=w864, "Timer"=u32 40, "State Machine in"=w865) -> ("error out"=w861:errorcluster, "State Machine out"=w862:refnum<class "State Machine.lvclass">)  [unwired: 7 in]
              n324 = call-dynamic "Init Ticks.vi"("error in (no error)"=w861, "State Machine in"=w862) -> ("error out"=w859:errorcluster, "State Machine out"=w860:refnum<class "State Machine.lvclass">)  [unwired: 8 in]
              n325 = call-dynamic "Write State Machine.vi"("error in (no error)"=w859, "State Machine.lvclass"=w860, "Device in"=w882) -> ("error out"=w866:errorcluster, "Device out"=w868:refnum<class "Opt_Selector.lvclass">)  [unwired: 7 in]
            }
          }
          n326 = call "Read id.vi"("Server in"=w795) -> ("id"=w797:u32)  [unwired: 8 in, 2 out]
          n327 = Increment(x=w797) -> (x+1=w796:u32)
          n328 = Number To Decimal String(number=w796) -> (decimal integer string=w793:string)  [unwired: 1 in]
          n329 = call "Write WPROT.vi"("error in (no error)"=w811, "Opt_Selector.lvclass"=w813, "Instrument in"=w812) -> ("error out"=w815:errorcluster, "Instrument out"=w814:refnum<class "Instrument.lvclass">)  [unwired: 7 in]
          n330 = Number To Decimal String(number=w799) -> (decimal integer string=w800:string)  [unwired: 1 in]
          n331 = Concatenate Strings("SeqAtual=" ("string"), w800, " CH=" ("string"), w793, " - S4GUI:HandleObservationAsync.vi (state=303)" ("string")) -> (w791:string)
          n332 = Bundle By Name(cluster=w802, "seqAtual"=w799, "App Event"=w791) -> (w801:refnum<class "S4GUI.lvclass">)
          n333 = call "Write Instrument.lvclass.vi"("error in (no error)"=w815, "Instrument.lvclass"=w814, "S4ACS_GUI in"=w801) -> ("error out"=w809:errorcluster, "S4ACS_GUI out"=w808:refnum<class "S4GUI.lvclass">)  [unwired: 7 in]
          n334 = call-dynamic "Write Acq_state.vi"("error in (no error)"=w809, "Acq_state"=w810, "Acquisition in"=w795) -> ("error out"=w807:errorcluster, "Acquisition out"=w806:refnum<class "Acquisition.lvclass">)  [unwired: 7 in]
        }
        frame 304 {
          # "Para inserir Pausa antes do\nEXPOSE, ir para 305."
          # "Espera terminar o movimento para a posição \"target\" do waveplate\nantes de ir para o estado que dispara a aquisição de imagens.\n\n20230424: Não precisa mais atualizar o valor de WPPOS com o\ncomando WRITE_HEADER porque o ACS já recebeu a sequência de\nposições da lâmina"
          n335 = flat-sequence {
            tunnel: [w945] -> w912
            tunnel: w913 -> [w945]
            frame #0 {
              n336 = Tick Count (ms)() -> (millisecond timer value=→"time 2":u32)
            }
          }
          n337 = call "Read Instrument.lvclass.vi"("error in (no error)"=w912, "S4ACS_GUI in"=w925) -> ("error out"=w930:errorcluster, "Instrument.lvclass"=w931:refnum<class "Instrument.lvclass">, "S4ACS_GUI out"=w927:refnum<class "S4GUI.lvclass">)  [unwired: 7 in]
          n338 = call "Read WPROT.vi"("error in (no error)"=w930, "Instrument in"=w931) -> ("error out"=w895:errorcluster, "Opt_Selector.lvclass"=w924:refnum<class "Opt_Selector.lvclass">, "Instrument out"=w929:refnum<class "Instrument.lvclass">)  [unwired: 7 in]
          n339 = call-dynamic "Read Channel.vi"("error in (no error)"=w895, "Acquisition in"=w897) -> ("error out"=w891:errorcluster, "Channel.lvclass"=w892:refnum<class "Channel.lvclass">, "Acquisition out"=w896:refnum<class "Acquisition.lvclass">)  [unwired: 7 in]
          n340 = call-dynamic "Read wait_expose.vi"("error in (no error)"=w891, "Channel in"=w892) -> ("error out"=w894:errorcluster, "wait_expose"=w893:bool)  [unwired: 7 in, 1 out]
          n341 = call-dynamic "Read State Machine.vi"("error in (no error)"=w894, "Device in"=w924) -> ("error out"=w901:errorcluster, "State Machine.lvclass"=w904:refnum<class "State Machine.lvclass">, "Device out"=w922:refnum<class "Opt_Selector.lvclass">)  [unwired: 7 in]
          n342 = call-dynamic "Verif Clock.vi"("error in (no error)"=w901, "period (ms)"=u32 20000 ("period"), "State Machine in"=w904) -> ("error out"=w905:errorcluster, "State Machine out"=w903:refnum<class "State Machine.lvclass">)  [unwired: 6 in, 1 out]
          n343 = call-dynamic "Read Timeout.vi"("error in (no error)"=w905, "State Machine in"=w903) -> ("error out"=w900:errorcluster, "Timeout"=w899:bool, "State Machine out"=w902:refnum<class "State Machine.lvclass">)  [unwired: 7 in]
          n344 = call-dynamic "Read State.vi"("error in (no error)"=w900, "State Machine in"=w902) -> ("error out"=w914:errorcluster, "State"=w920:i32, "State Machine out"=w915:refnum<class "State Machine.lvclass">)  [unwired: 7 in]
          n345 = call-dynamic "Write State Machine.vi"("error in (no error)"=w914, "State Machine.lvclass"=w915, "Device in"=w922) -> ("error out"=w921:errorcluster, "Device out"=w923:refnum<class "Opt_Selector.lvclass">)  [unwired: 7 in]
          n346 = Equal To 0?(x=w920) -> (x = 0?=w888:bool)
          n347 = call "Write WPROT.vi"("error in (no error)"=w921, "Opt_Selector.lvclass"=w923, "Instrument in"=w929) -> ("error out"=w926:errorcluster, "Instrument out"=w928:refnum<class "Instrument.lvclass">)  [unwired: 7 in]
          n348 = call "Write Instrument.lvclass.vi"("error in (no error)"=w926, "Instrument.lvclass"=w928, "S4ACS_GUI in"=w927) -> ("error out"=w918:errorcluster, "S4ACS_GUI out"=w907:refnum<class "S4GUI.lvclass">)  [unwired: 7 in]
          n349 = case shown="False" w899 {
            tunnel: w889 -> [w934 _]
            tunnel: [w934 u32 1 ("Obs_state")] -> w908
            tunnel: w907 -> [w933 w939]
            tunnel: [w933 w938] -> w898
            tunnel: [w932 FALSE] -> w887
            tunnel: w888 -> [w932 _]
            frame False {
            }
            frame True {
              n350 = Bundle By Name(cluster=w939, "Error Msg"="ERROR: moving waveplate (S4GUI:HandleObservationAsync.vi - state 304)") -> (w938:refnum<class "S4GUI.lvclass">)
            }
          }
          n351 = Unbundle By Name(w907) -> ("cyclesDone"=w910:u32, "sequesDone"=w909:u32)
          n352 = Add(x=w910, y=w909) -> (x+y=w911:u32)
          n353 = Equal To 0?(x=w911) -> ()  [unwired: 1 out]
          n354 = case shown="True" TRUE {
            tunnel: [w940 u32 308 ("t")] -> w886
            tunnel: w893 -> [w942 _]
            frame False {
              # "2a seq. em diante: depende\nde Channel.wait_expose"
              n355 = Select(t=u32 308, s=w942, f=u32 326 ("t")) -> (s? t:f=w940:u32)
            }
            frame True {
              # "1a. seq.: Envia EXPOSE"
            }
          }
          n356 = Increment(x=w889) -> ()  [unwired: 1 out]
          n357 = Select(t=w886, s=w887, f=w908) -> (s? t:f=w919:u32)
          n358 = call-dynamic "Write Acq_state.vi"("error in (no error)"=w918, "Acq_state"=w919, "Acquisition in"=w896) -> ("error out"=w917:errorcluster, "Acquisition out"=w916:refnum<class "Acquisition.lvclass">)  [unwired: 7 in]
        }
        frame 305 {
          # "Pausa de 200ms entre posicio-\nnamento da lamina e o envio de\nEXPOSE."
          n359 = Tick Count (ms)() -> (millisecond timer value=w954:u32)
          n360 = local read "time 2"() -> (w956:u32)
          n361 = Subtract(x=w954, y=w956) -> (x-y=w958:u32)
          n362 = To Double Precision Float(number=w958) -> (double precision float=w959:dbl)
          n363 = Less?(x=200.0 ("y"), y=w959) -> (x < y?=w955:bool)
          n364 = case shown="True" w955 {
            tunnel: [w960 u32 308 ("t")] -> w950
            tunnel: w954 -> [_ w961]
            tunnel: w951 -> [w960 _]
            frame False {
            }
            frame True {
              # "1a sequencia:\nenvia EXPOSE"
              n365 = local write "time 2"(w961) -> ()
            }
          }
          n366 = call-dynamic "Write Acq_state.vi"("error in (no error)"=w952, "Acq_state"=w950, "Acquisition in"=w953) -> ("error out"=w949:errorcluster, "Acquisition out"=w948:refnum<class "Acquisition.lvclass">)  [unwired: 7 in]
        }
        frame 308 {
          # "Dispara o comando para o dispositivo corrente."
          n367 = call-dynamic "Read Channel.vi"("error in (no error)"=w973, "Acquisition in"=w974) -> ("error out"=w980:errorcluster, "Channel.lvclass"=w979:refnum<class "Channel.lvclass">, "Acquisition out"=w984:refnum<class "Acquisition.lvclass">)  [unwired: 7 in]
          n368 = call-dynamic "Read State Machine.vi"("error in (no error)"=w980, "Device in"=w979) -> ("error out"=w981:errorcluster, "State Machine.lvclass"=w983:refnum<class "State Machine.lvclass">, "Device out"=w977:refnum<class "Channel.lvclass">)  [unwired: 7 in]
          n369 = call "Next State.vi"("error in (no error)"=w981, "New_State"=50, "State Machine in"=w983) -> ("error out"=w966:errorcluster, "State Machine out"=w967:refnum<class "State Machine.lvclass">)  [unwired: 7 in]
          n370 = call-dynamic "Write State Machine.vi"("error in (no error)"=w966, "State Machine.lvclass"=w967, "Device in"=w977) -> ("error out"=w976:errorcluster, "Device out"=w978:refnum<class "Channel.lvclass">)  [unwired: 7 in]
          n371 = Increment(x=w975) -> (x+1=w972:u32)
          n372 = call-dynamic "Write Channel.vi"("error in (no error)"=w976, "Channel.lvclass"=w978, "Acquisition in"=w984) -> ("error out"=w971:errorcluster, "Acquisition out"=w970:refnum<class "Acquisition.lvclass">)  [unwired: 7 in]
          n373 = call-dynamic "Write Acq_state.vi"("error in (no error)"=w971, "Acq_state"=w972, "Acquisition in"=w970) -> ("error out"=w968:errorcluster, "Acquisition out"=w969:refnum<class "Acquisition.lvclass">)  [unwired: 7 in]
          n374 = Bundle By Name(cluster=w965, "Error Msg"="") -> (w963:refnum<class "S4GUI.lvclass">)
        }
        frame 309 {
          # "OV 20241016 -Cancelada a verificacao do \nSeqsDone incrementar, pois agora o ACS garante as\ntransicoes Detector Status:  IDLE->ACTIVE->WAITING..."
          # "Se wait_expose=T, não envia\no EXPOSE do estado 308\n(1o EXPOSE já foi enviado).\n\nNeste caso, vai para:\n* 312 se houver mais \n   de 1 posição da lamina ou para \n* 326 se houver apenas 1 posição\n   da lâmina"
          # "OV 20240821 -Espera ACTIVE ou SeqsDone incrementar."
          n375 = Unbundle By Name(w1006) -> ("seqAtual"=w1005:u32)
          n376 = flat-sequence {
            tunnel: [w1047] -> w989
            tunnel: w1001 -> [w1047]
            frame #0 {
              n377 = Tick Count (ms)() -> (millisecond timer value=→"time308":u32)
            }
          }
          n378 = call "Read id.vi"("error in (no error)"=w989, "Server in"=w987) -> ("error out"=w988:errorcluster, "id"=w985:u32, "Server out"=w986:refnum<class "Acquisition.lvclass">)  [unwired: 7 in]
          n379 = call-dynamic "Read Channel.vi"("error in (no error)"=w988, "Acquisition in"=w986) -> ("error out"=w993:errorcluster, "Channel.lvclass"=w995:refnum<class "Channel.lvclass">, "Acquisition out"=w1030:refnum<class "Acquisition.lvclass">)  [unwired: 7 in]
          n380 = call-dynamic "Read Status.vi"("error in (no error)"=w993, "Channel in"=w995) -> ("error out"=w992:errorcluster, "Status"=w991:T2, "Channel out"=w994:refnum<class "Channel.lvclass">)  [unwired: 7 in]
          n381 = Unbundle By Name(w991) -> ("Error"=w990:bool)
          n382 = call-dynamic "Read SequesDone.vi"("error in (no error)"=w992, "Channel in"=w994) -> ("error out"=w1007:errorcluster, "SequesDoneRaw"=w1008:u32, "Channel out"=w1009:refnum<class "Channel.lvclass">)  [unwired: 6 in, 1 out]
          n383 = call-dynamic "Read wait_expose.vi"("error in (no error)"=w1007, "Channel in"=w1009) -> ("error out"=w1015:errorcluster, "Channel out"=w1016:refnum<class "Channel.lvclass">)  [unwired: 7 in, 1 out]
          n384 = Equal?(x=w1008, y=w1005) -> (x = y?=w1002:bool)
          n385 = call-dynamic "Read State Machine.vi"("error in (no error)"=w1015, "Device in"=w1016) -> ("error out"=w1024:errorcluster, "State Machine.lvclass"=w1026:refnum<class "State Machine.lvclass">, "Device out"=w1028:refnum<class "Channel.lvclass">)  [unwired: 7 in]
          n386 = call-dynamic "Read State.vi"("error in (no error)"=w1024, "State Machine in"=w1026) -> ("error out"=w1023:errorcluster, "State"=w1018:i32, "State Machine out"=w1025:refnum<class "State Machine.lvclass">)  [unwired: 7 in]
          n387 = call-dynamic "Write State Machine.vi"("error in (no error)"=w1023, "State Machine.lvclass"=w1025, "Device in"=w1028) -> ("error out"=w1027:errorcluster, "Device out"=w1029:refnum<class "Channel.lvclass">)  [unwired: 7 in]
          n388 = Greater?(x=w1018, y=53) -> (0:w1004:bool)
          n389 = disable-structure shown="Enabled" {
            disable-tunnel: w1004 -> [w1045 w1046]
            disable-tunnel: [w1044 w1046] -> w1003
            disable-tunnel: w1002 -> [w1043 _]
            frame Disabled {
              n390 = Or(x=w1045, y=w1043) -> (x .or. y?=w1044:bool)
            }
            frame Enabled {
            }
          }
          n391 = call-dynamic "Write Channel.vi"("error in (no error)"=w1027, "Channel.lvclass"=w1029, "Acquisition in"=w1030) -> ("error out"=w1014:errorcluster, "Acquisition out"=w1022:refnum<class "Acquisition.lvclass">)  [unwired: 7 in]
          n392 = call-dynamic "VerifWavePlate.vi"("error in (no error)"=w1014, "S4GUI in"=w1006) -> ("error out"=w1013:errorcluster, "One Position"=w1012:bool, "S4GUI out"=w997:refnum<class "S4GUI.lvclass">)  [unwired: 7 in]
          n393 = Select(t=u32 328, s=w1012, f=u32 312 ("t")) -> (s? t:f=w1000:u32)
          n394 = Select(t=w1000, s=w1003, f=w1017) -> (s? t:f=w999:u32)
          n395 = case shown="True" w990 {
            tunnel: [w1033 u32 1 ("Acq_state")] -> w998
            tunnel: w999 -> [w1033 _]
            tunnel: w997 -> [w1032 w1037]
            tunnel: [w1032 w1036] -> w996
            tunnel: w985 -> [_ w1035]
            frame False {
              n396 = Tick Count (ms)() -> (millisecond timer value=w1031:u32)
              n397 = local write "time307"(w1031) -> ()
            }
            frame True {
              n398 = Increment(x=w1035) -> (x+1=w1034:u32)
              n399 = Number To Decimal String(number=w1034) -> (decimal integer string=w1040:string)  [unwired: 1 in]
              n400 = Concatenate Strings("CHANNEL ", w1040, ": Error flag TRUE - see ACS panel.  HandleObservationAsync.vi - state 309.") -> (w1042:string)
              n401 = Bundle By Name(cluster=w1037, "Error Msg"=w1042) -> (w1036:refnum<class "S4GUI.lvclass">)
            }
          }
          n402 = call-dynamic "Write Acq_state.vi"("error in (no error)"=w1013, "Acq_state"=w998, "Acquisition in"=w1022) -> ("error out"=w1020:errorcluster, "Acquisition out"=w1021:refnum<class "Acquisition.lvclass">)  [unwired: 7 in]
        }
        frame 312 {
          # "Exemplo:\nSET #CYCLES 3\nSET #SEQ 4\ntotal de sequencias: 3 x 4 = 12\n\nseq.        CYCLES_DONE           SEQS_DONE\n1a.                     0                                 0\n2a.                     0                                 1 \n3a.                     0                                 2 \n4a.                     0                                 3 \n\n5a.                     1                                 4->0 \n6a.                     1                                 1 \n7a.                     1                                 2 \n8a.                     1                                 3 \n\n9a.                     2                                 4->0 \n10a.                   2                                 1 \n11a.                   2                                 2 \n12a.                   2                                 3 \n\nfim                    3                                 4"
          # "SEQS_DONE = 0,1,2,...,n,0,1,..."
          n403 = Unbundle By Name(w1066) -> ("seqAtual"=w1067:u32)
          n404 = call-dynamic "Read Channel.vi"("error in (no error)"=w1072, "Acquisition in"=w1073) -> ("error out"=w1059:errorcluster, "Channel.lvclass"=w1061:refnum<class "Channel.lvclass">, "Acquisition out"=w1074:refnum<class "Acquisition.lvclass">)  [unwired: 7 in]
          n405 = call-dynamic "Read stopping.vi"("error in (no error)"=w1059, "Channel in"=w1061) -> ("error out"=w1058:errorcluster, "stopping"=w1057:bool, "Channel out"=w1060:refnum<class "Channel.lvclass">)  [unwired: 7 in]
          n406 = call-dynamic "Read SequesDone.vi"("error in (no error)"=w1058, "Channel in"=w1060) -> ("error out"=w1068:errorcluster, "SequesDoneRaw"=w1049:u32, "Channel out"=w1069:refnum<class "Channel.lvclass">)  [unwired: 6 in, 1 out]
          n407 = Equal?(x=w1049, y=w1067) -> (x = y?=w1062:bool)
          n408 = call-dynamic "Write Channel.vi"("error in (no error)"=w1068, "Channel.lvclass"=w1069, "Acquisition in"=w1074) -> ("error out"=w1055:errorcluster, "Acquisition out"=w1056:refnum<class "Acquisition.lvclass">)  [unwired: 7 in]
          n409 = call-dynamic "GetCubeDuration.vi"("error in (no error)"=w1055, "Acquisition in"=w1056) -> ("error out"=w1054:errorcluster, "Acquisition out"=w1053:refnum<class "Acquisition.lvclass">, "CubeDuration"=w1052:dbl)  [unwired: 7 in]
          n410 = Multiply(x=w1052, y=1000.0) -> (x*y=w1051:dbl)
          n411 = case shown="False" w1062 {
            tunnel: w1066 -> [w1076 w1093]
            tunnel: [w1075 w1093] -> w1065
            tunnel: [w1077 w1095] -> w1064
            tunnel: w1063 -> [w1078 _]
            tunnel: w1057 -> [_ w1094]
            tunnel: w1051 -> [w1084 _]
            frame False {
              n412 = Add(x=5000.0, y=w1084) -> (x+y=w1082:dbl)
              n413 = local read "time307"() -> (w1085:u32)
              n414 = Tick Count (ms)() -> (millisecond timer value=w1086:u32)
              n415 = Subtract(x=w1086, y=w1085) -> (x-y=w1081:u32)
              n416 = To Double Precision Float(number=w1081) -> (double precision float=w1080:dbl)
              n417 = Less?(x=w1082, y=w1080) -> (x < y?=w1079:bool)
              n418 = case shown="True" w1079 {
                tunnel: w1078 -> [w1088 _]
                tunnel: [w1088 u32 1 ("Acq_state")] -> w1077
                tunnel: [w1087 w1090] -> w1075
                tunnel: w1076 -> [w1087 w1091]
                frame False {
                }
                frame True {
                  n419 = Bundle By Name(cluster=w1091, "Error Msg"="ERROR: Acquisition Timeout - HandleObservationAsync.vi - state 312.") -> (w1090:refnum<class "S4GUI.lvclass">)
                }
              }
            }
            frame True {
              n420 = case shown="False" w1094 {
                tunnel: [u32 303 ("Obs_state") u32 0 ("Obs_state")] -> w1095
                frame False {
                }
                frame True {
                }
              }
            }
          }
          n421 = call-dynamic "Write Acq_state.vi"("error in (no error)"=w1054, "Acq_state"=w1064, "Acquisition in"=w1053) -> ("error out"=w1070:errorcluster, "Acquisition out"=w1071:refnum<class "Acquisition.lvclass">)  [unwired: 7 in]
        }
        frame 314 {
          n422 = disable-structure shown="Enabled" {
            disable-tunnel: w1103 -> [w1120 w1136]
            disable-tunnel: w1102 -> [w1119 w1137]
            disable-tunnel: [w1108 w1135] -> w1101
            disable-tunnel: [w1107 w1134] -> w1100
            disable-tunnel: w1099 -> [w1104 w1131]
            disable-tunnel: [w1104 w1130] -> w1098
            frame Disabled {
              n423 = call-dynamic "Read Channel.vi"("error in (no error)"=w1120, "Acquisition in"=w1119) -> ("error out"=w1118:errorcluster, "Channel.lvclass"=w1117:refnum<class "Channel.lvclass">, "Acquisition out"=w1105:refnum<class "Acquisition.lvclass">)  [unwired: 7 in]
              n424 = call-dynamic "Read ciclos.vi"("error in (no error)"=w1118, "Channel in"=w1117) -> ("error out"=w1114:errorcluster, "ciclos"=w1116:u32, "Channel out"=w1106:refnum<class "Channel.lvclass">)  [unwired: 7 in]
              n425 = Decrement(x=w1116) -> (x-1=w1121:u32)
              n426 = Greater Than 0?(x=w1121) -> (x > 0?=w1125:bool)
              n427 = case shown="True" w1125 {
                selector: w1125 -> [w1127 w1129]
                tunnel: w1121 -> [_ w1128]
                tunnel: [w1127 w1129] -> w1124
                tunnel: [u32 0 w1128] -> w1111
                frame False {
                }
                frame True {
                }
              }
              n428 = call-dynamic "Write ciclos.vi"("error in (no error)"=w1114, "ciclos"=w1111, "Channel in"=w1106) -> ("error out"=w1113:errorcluster, "Channel out"=w1112:refnum<class "Channel.lvclass">)  [unwired: 7 in]
              n429 = Select(t=u32 301, s=w1124, f=u32 0) -> (s? t:f=w1115:u32)
              n430 = call-dynamic "Write Channel.vi"("error in (no error)"=w1113, "Channel.lvclass"=w1112, "Acquisition in"=w1105) -> ("error out"=w1109:errorcluster, "Acquisition out"=w1110:refnum<class "Acquisition.lvclass">)  [unwired: 7 in]
              n431 = call-dynamic "Write Acq_state.vi"("error in (no error)"=w1109, "Acq_state"=w1115, "Acquisition in"=w1110) -> ("error out"=w1107:errorcluster, "Acquisition out"=w1108:refnum<class "Acquisition.lvclass">)  [unwired: 7 in]
            }
            frame Enabled {
              n432 = Unbundle By Name(w1131) -> ("cyclesDone"=w1133:u32)
              n433 = Increment(x=w1133) -> (x+1=w1132:u32)
              n434 = Bundle By Name(cluster=w1131, "cyclesDone"=w1132) -> (w1130:refnum<class "S4GUI.lvclass">)
              n435 = Unbundle By Name(w1130) -> ("TotalCiclos"=w1144:u32, "cyclesDone"=w1143:u32)
              n436 = Subtract(x=w1144, y=w1143) -> (x-y=w1142:u32)
              n437 = Greater Than 0?(x=w1142) -> (x > 0?=w1141:bool)
              n438 = Select(t=u32 303, s=w1141, f=u32 0) -> (s? t:f=w1138:u32)
              n439 = call-dynamic "Write Acq_state.vi"("error in (no error)"=w1136, "Acq_state"=w1138, "Acquisition in"=w1137) -> ("error out"=w1134:errorcluster, "Acquisition out"=w1135:refnum<class "Acquisition.lvclass">)  [unwired: 7 in]
            }
          }
        }
        frame 321 {
          # "Envia: WAIT_EXPOSE_COMMAND  OFF"
          # "Para Fotometria Async -> DESABILITA comando EXPOSE para os ACS."
          n440 = call-dynamic "Read Channel.vi"("error in (no error)"=w1160, "Acquisition in"=w1161) -> ("error out"=w1147:errorcluster, "Channel.lvclass"=w1149:refnum<class "Channel.lvclass">, "Acquisition out"=w1169:refnum<class "Acquisition.lvclass">)  [unwired: 7 in]
          n441 = call-dynamic "Write wait_expose.vi"("error in (no error)"=w1147, "wait_expose"=FALSE, "Channel in"=w1149) -> ("error out"=w1146:errorcluster, "Channel out"=w1148:refnum<class "Channel.lvclass">)  [unwired: 7 in]
          n442 = call-dynamic "Read State Machine.vi"("error in (no error)"=w1146, "Device in"=w1148) -> ("error out"=w1166:errorcluster, "State Machine.lvclass"=w1168:refnum<class "State Machine.lvclass">, "Device out"=w1164:refnum<class "Channel.lvclass">)  [unwired: 7 in]
          n443 = call "Next State.vi"("error in (no error)"=w1166, "New_State"=40, "State Machine in"=w1168) -> ("error out"=w1153:errorcluster, "State Machine out"=w1154:refnum<class "State Machine.lvclass">)  [unwired: 7 in]
          n444 = call-dynamic "Write State Machine.vi"("error in (no error)"=w1153, "State Machine.lvclass"=w1154, "Device in"=w1164) -> ("error out"=w1163:errorcluster, "Device out"=w1165:refnum<class "Channel.lvclass">)  [unwired: 7 in]
          n445 = Increment(x=w1162) -> (x+1=w1159:u32)
          n446 = call-dynamic "Write Channel.vi"("error in (no error)"=w1163, "Channel.lvclass"=w1165, "Acquisition in"=w1169) -> ("error out"=w1158:errorcluster, "Acquisition out"=w1157:refnum<class "Acquisition.lvclass">)  [unwired: 7 in]
          n447 = call-dynamic "Write Acq_state.vi"("error in (no error)"=w1158, "Acq_state"=w1159, "Acquisition in"=w1157) -> ("error out"=w1155:errorcluster, "Acquisition out"=w1156:refnum<class "Acquisition.lvclass">)  [unwired: 7 in]
          n448 = Bundle By Name(cluster=w1152, "Error Msg"="") -> (w1150:refnum<class "S4GUI.lvclass">)
        }
        frame 322 {
          # "Espera canal voltar para IDLE"
          n449 = call-dynamic "Read Channel.vi"("error in (no error)"=w1185, "Acquisition in"=w1186) -> ("error out"=w1176:errorcluster, "Channel.lvclass"=w1177:refnum<class "Channel.lvclass">, "Acquisition out"=w1178:refnum<class "Acquisition.lvclass">)  [unwired: 7 in]
          n450 = call-dynamic "Read State Machine.vi"("error in (no error)"=w1176, "Device in"=w1177) -> ("error out"=w1179:errorcluster, "State Machine.lvclass"=w1181:refnum<class "State Machine.lvclass">)  [unwired: 7 in, 1 out]
          n451 = call-dynamic "Read State.vi"("error in (no error)"=w1179, "State Machine in"=w1181) -> ("error out"=w1174:errorcluster, "State"=w1180:i32)  [unwired: 7 in, 1 out]
          n452 = Equal?(x=0, y=w1180) -> (x = y?=w1170:bool)
          n453 = Increment(x=w1172) -> (x+1=w1173:u32)
          n454 = Select(t=w1173, s=w1170, f=w1172) -> (s? t:f=w1175:u32)
          n455 = call-dynamic "Write Acq_state.vi"("error in (no error)"=w1174, "Acq_state"=w1175, "Acquisition in"=w1178) -> ("error out"=w1183:errorcluster, "Acquisition out"=w1184:refnum<class "Acquisition.lvclass">)  [unwired: 7 in]
        }
        frame 323 {
          # "Envia: EXPOSE para o ACS"
          # "Dispara o comando para o dispositivo corrente."
          n456 = flat-sequence {
            tunnel: w1188 -> [w1210]
            tunnel: [w1210] -> w1187
            frame #0 {
              n457 = Tick Count (ms)() -> (millisecond timer value=w1211:u32)
              n458 = local write "time 2"(w1211) -> ()
            }
          }
          n459 = call-dynamic "Read Channel.vi"("error in (no error)"=w1187, "Acquisition in"=w1199) -> ("error out"=w1205:errorcluster, "Channel.lvclass"=w1204:refnum<class "Channel.lvclass">, "Acquisition out"=w1209:refnum<class "Acquisition.lvclass">)  [unwired: 7 in]
          n460 = call-dynamic "Read State Machine.vi"("error in (no error)"=w1205, "Device in"=w1204) -> ("error out"=w1206:errorcluster, "State Machine.lvclass"=w1208:refnum<class "State Machine.lvclass">, "Device out"=w1202:refnum<class "Channel.lvclass">)  [unwired: 7 in]
          n461 = call "Next State.vi"("error in (no error)"=w1206, "New_State"=50, "State Machine in"=w1208) -> ("error out"=w1192:errorcluster, "State Machine out"=w1193:refnum<class "State Machine.lvclass">)  [unwired: 7 in]
          n462 = call-dynamic "Write State Machine.vi"("error in (no error)"=w1192, "State Machine.lvclass"=w1193, "Device in"=w1202) -> ("error out"=w1201:errorcluster, "Device out"=w1203:refnum<class "Channel.lvclass">)  [unwired: 7 in]
          n463 = Increment(x=w1200) -> (x+1=w1196:u32)
          n464 = call-dynamic "Write Channel.vi"("error in (no error)"=w1201, "Channel.lvclass"=w1203, "Acquisition in"=w1209) -> ("error out"=w1195:errorcluster, "Acquisition out"=w1197:refnum<class "Acquisition.lvclass">)  [unwired: 7 in]
          n465 = call-dynamic "Write Acq_state.vi"("error in (no error)"=w1195, "Acq_state"=w1196, "Acquisition in"=w1197) -> ("error out"=w1194:errorcluster, "Acquisition out"=w1198:refnum<class "Acquisition.lvclass">)  [unwired: 7 in]
          n466 = Bundle By Name(cluster=w1191, "Error Msg"="") -> (w1190:refnum<class "S4GUI.lvclass">)
        }
        frame 324 {
          # "Espera Status Detector entrar em ACTIVE"
          n467 = call "Read id.vi"("error in (no error)"=w1214, "Server in"=w1216) -> ("error out"=w1213:errorcluster, "id"=w1212:u32, "Server out"=w1215:refnum<class "Acquisition.lvclass">)  [unwired: 7 in]
          n468 = call-dynamic "Read Channel.vi"("error in (no error)"=w1213, "Acquisition in"=w1215) -> ("error out"=w1225:errorcluster, "Channel.lvclass"=w1226:refnum<class "Channel.lvclass">, "Acquisition out"=w1248:refnum<class "Acquisition.lvclass">)  [unwired: 7 in]
          n469 = call-dynamic "Read Status.vi"("error in (no error)"=w1225, "Channel in"=w1226) -> ("error out"=w1223:errorcluster, "Status"=w1224:T2, "Channel out"=w1222:refnum<class "Channel.lvclass">)  [unwired: 7 in]
          n470 = Unbundle By Name(w1224) -> ("Error"=w1219:bool)
          n471 = call-dynamic "Read wait_expose.vi"("error in (no error)"=w1223, "Channel in"=w1222) -> ("error out"=w1232:errorcluster, "wait_expose"=w1230:bool, "Channel out"=w1233:refnum<class "Channel.lvclass">)  [unwired: 7 in]
          n472 = call-dynamic "Read State Machine.vi"("error in (no error)"=w1232, "Device in"=w1233) -> ("error out"=w1242:errorcluster, "State Machine.lvclass"=w1244:refnum<class "State Machine.lvclass">, "Device out"=w1246:refnum<class "Channel.lvclass">)  [unwired: 7 in]
          n473 = call-dynamic "Read State.vi"("error in (no error)"=w1242, "State Machine in"=w1244) -> ("error out"=w1241:errorcluster, "State"=w1235:i32, "State Machine out"=w1243:refnum<class "State Machine.lvclass">)  [unwired: 7 in]
          n474 = Greater?(x=w1235, y=53) -> (0:w1227:bool)
          n475 = call-dynamic "Write State Machine.vi"("error in (no error)"=w1241, "State Machine.lvclass"=w1243, "Device in"=w1246) -> ("error out"=w1245:errorcluster, "Device out"=w1247:refnum<class "Channel.lvclass">)  [unwired: 7 in]
          n476 = call-dynamic "Write Channel.vi"("error in (no error)"=w1245, "Channel.lvclass"=w1247, "Acquisition in"=w1248) -> ("error out"=w1236:errorcluster, "Acquisition out"=w1237:refnum<class "Acquisition.lvclass">)  [unwired: 7 in]
          n477 = Increment(x=w1240) -> (x+1=w1229:u32)
          n478 = Select(t=327 ("y"), s=w1230, f=w1229) -> (s? t:f=w1228:u32)
          n479 = Select(t=w1228, s=w1227, f=w1240) -> (s? t:f=w1220:u32)
          n480 = case shown="True" w1219 {
            tunnel: [w1251 u32 1 ("Acq_state")] -> w1221
            tunnel: w1220 -> [w1251 _]
            tunnel: w1218 -> [w1250 w1255]
            tunnel: [w1250 w1254] -> w1217
            tunnel: w1212 -> [_ w1253]
            frame False {
              n481 = Tick Count (ms)() -> (millisecond timer value=w1249:u32)
              n482 = local write "time307"(w1249) -> ()
            }
            frame True {
              n483 = Increment(x=w1253) -> (x+1=w1252:u32)
              n484 = Number To Decimal String(number=w1252) -> (decimal integer string=w1258:string)  [unwired: 1 in]
              n485 = Concatenate Strings("CHANNEL ", w1258, ": Error flag TRUE - see ACS panel.  HandleObservationAsync.vi - state 324.") -> (w1260:string)
              n486 = Bundle By Name(cluster=w1255, "Error Msg"=w1260) -> (w1254:refnum<class "S4GUI.lvclass">)
            }
          }
          n487 = call-dynamic "Write Acq_state.vi"("error in (no error)"=w1236, "Acq_state"=w1221, "Acquisition in"=w1237) -> ("error out"=w1238:errorcluster, "Acquisition out"=w1239:refnum<class "Acquisition.lvclass">)  [unwired: 7 in]
        }
        frame 325 {
          # "Dispara o comando para o dispositivo corrente."
          n488 = call-dynamic "Read Channel.vi"("error in (no error)"=w1261, "Acquisition in"=w1266) -> ("error out"=w1267:errorcluster, "Channel.lvclass"=w1262:refnum<class "Channel.lvclass">, "Acquisition out"=w1264:refnum<class "Acquisition.lvclass">)  [unwired: 7 in]
          n489 = call-dynamic "Read wait_expose.vi"("error in (no error)"=w1267, "Channel in"=w1262) -> ("error out"=w1263:errorcluster, "wait_expose"=w1265:bool)  [unwired: 7 in, 1 out]
          n490 = case shown="False" w1265 {
            tunnel: w1264 -> [w1278 w1284]
            tunnel: w1263 -> [w1277 w1283]
            tunnel: [w1278 w1282] -> w1274
            tunnel: [w1277 w1281] -> w1272
            frame False {
            }
            frame True {
              n491 = call-dynamic "Read Channel.vi"("error in (no error)"=w1283, "Acquisition in"=w1284) -> ("error out"=w1289:errorcluster, "Channel.lvclass"=w1288:refnum<class "Channel.lvclass">, "Acquisition out"=w1293:refnum<class "Acquisition.lvclass">)  [unwired: 7 in]
              n492 = call-dynamic "Read State Machine.vi"("error in (no error)"=w1289, "Device in"=w1288) -> ("error out"=w1290:errorcluster, "State Machine.lvclass"=w1292:refnum<class "State Machine.lvclass">, "Device out"=w1286:refnum<class "Channel.lvclass">)  [unwired: 7 in]
              n493 = call "Next State.vi"("error in (no error)"=w1290, "New_State"=50, "State Machine in"=w1292) -> ("error out"=w1279:errorcluster, "State Machine out"=w1280:refnum<class "State Machine.lvclass">)  [unwired: 7 in]
              n494 = call-dynamic "Write State Machine.vi"("error in (no error)"=w1279, "State Machine.lvclass"=w1280, "Device in"=w1286) -> ("error out"=w1285:errorcluster, "Device out"=w1287:refnum<class "Channel.lvclass">)  [unwired: 7 in]
              n495 = call-dynamic "Write Channel.vi"("error in (no error)"=w1285, "Channel.lvclass"=w1287, "Acquisition in"=w1293) -> ("error out"=w1281:errorcluster, "Acquisition out"=w1282:refnum<class "Acquisition.lvclass">)  [unwired: 7 in]
            }
          }
          n496 = Increment(x=w1276) -> (x+1=w1273:u32)
          n497 = call-dynamic "Write Acq_state.vi"("error in (no error)"=w1272, "Acq_state"=w1273, "Acquisition in"=w1274) -> ("error out"=w1271:errorcluster, "Acquisition out"=w1275:refnum<class "Acquisition.lvclass">)  [unwired: 7 in]
          n498 = Bundle By Name(cluster=w1268, "Error Msg"="") -> (w1270:refnum<class "S4GUI.lvclass">)
        }
        frame 326 {
          # "Espera Status Detector entrar em ACTIVE"
          n499 = call "Read id.vi"("error in (no error)"=w1296, "Server in"=w1299) -> ("error out"=w1297:errorcluster, "id"=w1295:u32, "Server out"=w1298:refnum<class "Acquisition.lvclass">)  [unwired: 7 in]
          n500 = call-dynamic "Read Channel.vi"("error in (no error)"=w1297, "Acquisition in"=w1298) -> ("error out"=w1301:errorcluster, "Channel.lvclass"=w1304:refnum<class "Channel.lvclass">, "Acquisition out"=w1326:refnum<class "Acquisition.lvclass">)  [unwired: 7 in]
          n501 = call-dynamic "Read Status.vi"("error in (no error)"=w1301, "Channel in"=w1304) -> ("error out"=w1300:errorcluster, "Status"=w1302:T2, "Channel out"=w1303:refnum<class "Channel.lvclass">)  [unwired: 7 in]
          n502 = Unbundle By Name(w1302) -> ("Error"=w1294:bool)
          n503 = call-dynamic "Read State Machine.vi"("error in (no error)"=w1300, "Device in"=w1303) -> ("error out"=w1320:errorcluster, "State Machine.lvclass"=w1322:refnum<class "State Machine.lvclass">, "Device out"=w1324:refnum<class "Channel.lvclass">)  [unwired: 7 in]
          n504 = call-dynamic "Read State.vi"("error in (no error)"=w1320, "State Machine in"=w1322) -> ("error out"=w1319:errorcluster, "State"=w1313:i32, "State Machine out"=w1321:refnum<class "State Machine.lvclass">)  [unwired: 7 in]
          n505 = disable-structure shown="Enabled" {
            disable-tunnel: w1311 -> [w1328 w1329]
            disable-tunnel: [w1327 w1329] -> w1310
            frame Disabled {
              n506 = Increment(x=w1328) -> (x+1=w1327:u32)
            }
            frame Enabled {
              # "OV20241108:\nNão espera mais \nCyclesDone>0 em 327"
            }
          }
          n507 = Greater?(x=w1313, y=53) -> (0:w1318:bool)
          n508 = call-dynamic "Write State Machine.vi"("error in (no error)"=w1319, "State Machine.lvclass"=w1321, "Device in"=w1324) -> ("error out"=w1323:errorcluster, "Device out"=w1325:refnum<class "Channel.lvclass">)  [unwired: 7 in]
          n509 = call-dynamic "Write Channel.vi"("error in (no error)"=w1323, "Channel.lvclass"=w1325, "Acquisition in"=w1326) -> ("error out"=w1314:errorcluster, "Acquisition out"=w1315:refnum<class "Acquisition.lvclass">)  [unwired: 7 in]
          n510 = Select(t=u32 328, s=w1318, f=w1310) -> (s? t:f=w1308:u32)
          n511 = case shown="False" w1294 {
            tunnel: [w1332 u32 1 ("Acq_state")] -> w1307
            tunnel: w1308 -> [w1332 _]
            tunnel: w1306 -> [w1331 w1336]
            tunnel: [w1331 w1335] -> w1305
            tunnel: w1295 -> [_ w1334]
            frame False {
              n512 = Tick Count (ms)() -> (millisecond timer value=w1330:u32)
              n513 = local write "time307"(w1330) -> ()
            }
            frame True {
              n514 = Increment(x=w1334) -> (x+1=w1333:u32)
              n515 = Number To Decimal String(number=w1333) -> (decimal integer string=w1339:string)  [unwired: 1 in]
              n516 = Concatenate Strings("CHANNEL ", w1339, ": Error flag TRUE - see ACS panel.  HandleObservationAsync.vi - state 326.") -> (w1341:string)
              n517 = Bundle By Name(cluster=w1336, "Error Msg"=w1341) -> (w1335:refnum<class "S4GUI.lvclass">)
            }
          }
          n518 = call-dynamic "Write Acq_state.vi"("error in (no error)"=w1314, "Acq_state"=w1307, "Acquisition in"=w1315) -> ("error out"=w1316:errorcluster, "Acquisition out"=w1317:refnum<class "Acquisition.lvclass">)  [unwired: 7 in]
        }
        frame 327 {
          # "Verifica se CyclesDone lido do STATUS igualou ao PrevCycles+1"
          n519 = call "Read id.vi"("error in (no error)"=w1347, "Server in"=w1348) -> ("error out"=w1345:errorcluster, "id"=w1344:u32, "Server out"=w1346:refnum<class "Acquisition.lvclass">)  [unwired: 7 in]
          n520 = call-dynamic "Read Channel.vi"("error in (no error)"=w1345, "Acquisition in"=w1346) -> ("error out"=w1357:errorcluster, "Channel.lvclass"=w1358:refnum<class "Channel.lvclass">, "Acquisition out"=w1368:refnum<class "Acquisition.lvclass">)  [unwired: 7 in]
          n521 = Increment(x=w1344) -> (x+1=w1343:u32)
          n522 = call-dynamic "Read PrevCyclesDone.vi"("error in (no error)"=w1357, "Channel in"=w1358) -> ("error out"=w1360:errorcluster, "PrevCyclesDone"=w1359:u32, "Channel out"=w1361:refnum<class "Channel.lvclass">)  [unwired: 7 in]
          n523 = call-dynamic "Read CyclesDone.vi"("error in (no error)"=w1360, "Channel in"=w1361) -> ("error out"=w1354:errorcluster, "CyclesDone"=w1349:u32, "Channel out"=w1356:refnum<class "Channel.lvclass">)  [unwired: 7 in]
          n524 = Increment(x=w1359) -> (x+1=w1342:u32)
          n525 = call-dynamic "Read stopping.vi"("error in (no error)"=w1354, "Channel in"=w1356) -> ("error out"=w1353:errorcluster, "stopping"=w1351:bool, "Channel out"=w1355:refnum<class "Channel.lvclass">)  [unwired: 7 in]
          n526 = Equal?(x=w1349, y=w1342) -> (x = y?=w1352:bool)
          n527 = call-dynamic "Write Channel.vi"("error in (no error)"=w1353, "Channel.lvclass"=w1355, "Acquisition in"=w1368) -> ("error out"=w1364:errorcluster, "Acquisition out"=w1365:refnum<class "Acquisition.lvclass">)  [unwired: 7 in]
          n528 = case shown="True" w1352 {
            tunnel: [w1377 w1421] -> w1366
            tunnel: w1365 -> [w1373 w1409]
            tunnel: w1367 -> [w1371 w1420]
            tunnel: w1364 -> [w1374 w1408]
            tunnel: [w1379 w1418] -> w1363
            tunnel: w1362 -> [w1380 w1416]
            tunnel: w1351 -> [_ w1414]
            tunnel: [w1378 w1419] -> w1350
            tunnel: w1349 -> [_ w1413]
            tunnel: w1343 -> [w1376 _]
            frame False {
              # "Aguardando iniciar exposição por 5s"
              n529 = local read "time 2"() -> (w1370:u32)
              n530 = Tick Count (ms)() -> (millisecond timer value=w1383:u32)
              n531 = Subtract(x=w1383, y=w1370) -> (x-y=w1382:u32)
              n532 = To Double Precision Float(number=w1382) -> (double precision float=w1381:dbl)
              n533 = Number To Decimal String(number=w1376) -> (decimal integer string=w1375:string)  [unwired: 1 in]
              n534 = Less?(x=5000.0, y=w1381) -> (x < y?=w1369:bool)
              n535 = case shown="False" w1369 {
                tunnel: w1380 -> [w1390 w1403]
                tunnel: [w1390 w1402] -> w1379
                tunnel: [w1385 w1399] -> w1378
                tunnel: w1374 -> [w1386 w1398]
                tunnel: w1373 -> [w1389 w1401]
                tunnel: [w1387 w1400] -> w1377
                tunnel: w1375 -> [_ w1395]
                tunnel: w1371 -> [w1388 _]
                frame False {
                  n536 = disable-structure shown="Enabled" {
                    disable-tunnel: w1388 -> [w1392 w1393]
                    disable-tunnel: [w1391 w1393] -> w1384
                    frame Disabled {
                      # "Volta para \nesperar ACTIVE."
                      n537 = Decrement(x=w1392) -> (x-1=w1391:u32)
                    }
                    frame Enabled {
                      # "OV20241108:\nNão volta mais pra 326.\nSó verifica CyclesDone."
                    }
                  }
                  n538 = call-dynamic "Write Acq_state.vi"("error in (no error)"=w1386, "Acq_state"=w1384, "Acquisition in"=w1389) -> ("error out"=w1385:errorcluster, "Acquisition out"=w1387:refnum<class "Acquisition.lvclass">)  [unwired: 7 in]
                }
                frame True {
                  n539 = Concatenate Strings("ERROR: Init Acquisition Timeout. HandleObservationAsync.vi - state 327. Channel: ", w1395) -> (w1394:string)
                  n540 = call-dynamic "Write Acq_state.vi"("error in (no error)"=w1398, "Acq_state"=u32 1, "Acquisition in"=w1401) -> ("error out"=w1399:errorcluster, "Acquisition out"=w1400:refnum<class "Acquisition.lvclass">)  [unwired: 7 in]
                  n541 = Bundle By Name(cluster=w1403, "Error Msg"=w1394) -> (w1402:refnum<class "S4GUI.lvclass">)
                }
              }
            }
            frame True {
              # "STOP?"
              # "Avançou o ciclo."
              n542 = call-dynamic "Read Channel.vi"("error in (no error)"=w1408, "Acquisition in"=w1409) -> ("error out"=w1407:errorcluster, "Channel.lvclass"=w1412:refnum<class "Channel.lvclass">, "Acquisition out"=w1410:refnum<class "Acquisition.lvclass">)  [unwired: 7 in]
              n543 = call-dynamic "Write PrevCyclesDone.vi"("error in (no error)"=w1407, "PrevCyclesDone"=w1413, "Channel in"=w1412) -> ("error out"=w1406:errorcluster, "Channel out"=w1411:refnum<class "Channel.lvclass">)  [unwired: 7 in]
              n544 = call-dynamic "Write Channel.vi"("error in (no error)"=w1406, "Channel.lvclass"=w1411, "Acquisition in"=w1410) -> ("error out"=w1404:errorcluster, "Acquisition out"=w1405:refnum<class "Acquisition.lvclass">)  [unwired: 7 in]
              n545 = case shown="False" w1414 {
                tunnel: w1420 -> [w1424 _]
                tunnel: [w1422 u32 0] -> w1415
                frame False {
                  n546 = Increment(x=w1424) -> (x+1=w1423:u32)
                  n547 = Increment(x=w1423) -> (x+1=w1422:u32)
                }
                frame True {
                }
              }
              n548 = call-dynamic "Write Acq_state.vi"("error in (no error)"=w1404, "Acq_state"=w1415, "Acquisition in"=w1405) -> ("error out"=w1419:errorcluster, "Acquisition out"=w1421:refnum<class "Acquisition.lvclass">)  [unwired: 7 in]
              n549 = Bundle By Name(cluster=w1416, "Error Msg"="") -> (w1418:refnum<class "S4GUI.lvclass">)
            }
          }
        }
        frame 328 {
          # "Dispara o comando para o dispositivo corrente."
          n550 = call "Read id.vi"("error in (no error)"=w1431, "Server in"=w1432) -> ("error out"=w1429:errorcluster, "id"=w1428:u32, "Server out"=w1430:refnum<class "Acquisition.lvclass">)  [unwired: 7 in]
          n551 = call-dynamic "Read Channel.vi"("error in (no error)"=w1429, "Acquisition in"=w1430) -> ("error out"=w1441:errorcluster, "Channel.lvclass"=w1442:refnum<class "Channel.lvclass">, "Acquisition out"=w1452:refnum<class "Acquisition.lvclass">)  [unwired: 7 in]
          n552 = Increment(x=w1428) -> (x+1=w1427:u32)
          n553 = call-dynamic "Read PrevCyclesDone.vi"("error in (no error)"=w1441, "Channel in"=w1442) -> ("error out"=w1444:errorcluster, "PrevCyclesDone"=w1443:u32, "Channel out"=w1445:refnum<class "Channel.lvclass">)  [unwired: 7 in]
          n554 = call-dynamic "Read CyclesDone.vi"("error in (no error)"=w1444, "Channel in"=w1445) -> ("error out"=w1438:errorcluster, "CyclesDone"=w1433:u32, "Channel out"=w1440:refnum<class "Channel.lvclass">)  [unwired: 7 in]
          n555 = Increment(x=w1443) -> (x+1=w1426:u32)
          n556 = call-dynamic "Read stopping.vi"("error in (no error)"=w1438, "Channel in"=w1440) -> ("error out"=w1437:errorcluster, "stopping"=w1435:bool, "Channel out"=w1439:refnum<class "Channel.lvclass">)  [unwired: 7 in]
          n557 = Equal?(x=w1433, y=w1426) -> (x = y?=w1436:bool)
          n558 = call-dynamic "Write Channel.vi"("error in (no error)"=w1437, "Channel.lvclass"=w1439, "Acquisition in"=w1452) -> ("error out"=w1448:errorcluster, "Acquisition out"=w1449:refnum<class "Acquisition.lvclass">)  [unwired: 7 in]
          n559 = case shown="False" w1436 {
            tunnel: [w1458 w1503] -> w1450
            tunnel: w1449 -> [w1470 w1491]
            tunnel: w1451 -> [_ w1502]
            tunnel: w1448 -> [w1469 w1490]
            tunnel: [w1462 w1500] -> w1447
            tunnel: w1446 -> [w1463 w1498]
            tunnel: w1435 -> [_ w1496]
            tunnel: [w1460 w1501] -> w1434
            tunnel: w1433 -> [_ w1495]
            tunnel: w1427 -> [w1457 _]
            frame False {
              n560 = Tick Count (ms)() -> (millisecond timer value=w1472:u32)
              n561 = local read "time307"() -> (w1471:u32)
              n562 = call-dynamic "GetCubeDuration.vi"("error in (no error)"=w1469, "Acquisition in"=w1470) -> ("error out"=w1461:errorcluster, "Acquisition out"=w1459:refnum<class "Acquisition.lvclass">, "CubeDuration"=w1455:dbl)  [unwired: 7 in]
              n563 = Subtract(x=w1472, y=w1471) -> (x-y=w1466:u32)
              n564 = Multiply(x=w1455, y=1000.0) -> (x*y=w1453:dbl)
              n565 = To Double Precision Float(number=w1466) -> (double precision float=w1464:dbl)
              n566 = Add(x=5000.0, y=w1453) -> (x+y=w1467:dbl)
              n567 = Number To Decimal String(number=w1457) -> (decimal integer string=w1456:string)  [unwired: 1 in]
              n568 = Less?(x=w1467, y=w1464) -> (x < y?=w1465:bool)
              n569 = case shown="True" w1465 {
                tunnel: w1463 -> [w1475 w1485]
                tunnel: [w1475 w1484] -> w1462
                tunnel: [w1474 w1481] -> w1460
                tunnel: w1461 -> [w1474 w1480]
                tunnel: w1459 -> [w1473 w1483]
                tunnel: [w1473 w1482] -> w1458
                tunnel: w1456 -> [_ w1477]
                frame False {
                }
                frame True {
                  n570 = Concatenate Strings("ERROR: Acquisition Timeout. HandleObservationAsync.vi - state 328. Channel: ", w1477) -> (w1476:string)
                  n571 = call-dynamic "Write Acq_state.vi"("error in (no error)"=w1480, "Acq_state"=u32 1, "Acquisition in"=w1483) -> ("error out"=w1481:errorcluster, "Acquisition out"=w1482:refnum<class "Acquisition.lvclass">)  [unwired: 7 in]
                  n572 = Bundle By Name(cluster=w1485, "Error Msg"=w1476) -> (w1484:refnum<class "S4GUI.lvclass">)
                }
              }
            }
            frame True {
              n573 = call-dynamic "Read Channel.vi"("error in (no error)"=w1490, "Acquisition in"=w1491) -> ("error out"=w1489:errorcluster, "Channel.lvclass"=w1494:refnum<class "Channel.lvclass">, "Acquisition out"=w1492:refnum<class "Acquisition.lvclass">)  [unwired: 7 in]
              n574 = call-dynamic "Write PrevCyclesDone.vi"("error in (no error)"=w1489, "PrevCyclesDone"=w1495, "Channel in"=w1494) -> ("error out"=w1488:errorcluster, "Channel out"=w1493:refnum<class "Channel.lvclass">)  [unwired: 7 in]
              n575 = call-dynamic "Write Channel.vi"("error in (no error)"=w1488, "Channel.lvclass"=w1493, "Acquisition in"=w1492) -> ("error out"=w1486:errorcluster, "Acquisition out"=w1487:refnum<class "Acquisition.lvclass">)  [unwired: 7 in]
              n576 = case shown="False" w1496 {
                tunnel: w1502 -> [w1505 _]
                tunnel: [w1504 u32 0] -> w1497
                frame False {
                  n577 = Increment(x=w1505) -> (x+1=w1504:u32)
                }
                frame True {
                }
              }
              n578 = call-dynamic "Write Acq_state.vi"("error in (no error)"=w1486, "Acq_state"=w1497, "Acquisition in"=w1487) -> ("error out"=w1501:errorcluster, "Acquisition out"=w1503:refnum<class "Acquisition.lvclass">)  [unwired: 7 in]
              n579 = Bundle By Name(cluster=w1498, "Error Msg"="") -> (w1500:refnum<class "S4GUI.lvclass">)
            }
          }
        }
        frame 329 {
          n580 = call-dynamic "Read Channel.vi"("error in (no error)"=w1524, "Acquisition in"=w1525) -> ("error out"=w1518:errorcluster, "Channel.lvclass"=w1523:refnum<class "Channel.lvclass">, "Acquisition out"=w1510:refnum<class "Acquisition.lvclass">)  [unwired: 7 in]
          n581 = call-dynamic "Read CyclesDone.vi"("error in (no error)"=w1518, "Channel in"=w1523) -> ("error out"=w1526:errorcluster, "CyclesDone"=w1521:u32, "Channel out"=w1527:refnum<class "Channel.lvclass">)  [unwired: 7 in]
          n582 = call-dynamic "Read ciclos.vi"("error in (no error)"=w1526, "Channel in"=w1527) -> ("error out"=w1517:errorcluster, "ciclos"=w1522:u32, "Channel out"=w1516:refnum<class "Channel.lvclass">)  [unwired: 7 in]
          n583 = Subtract(x=w1522, y=w1521) -> (x-y=w1528:u32)
          n584 = Greater Than 0?(x=w1528) -> (x > 0?=w1508:bool)
          n585 = call-dynamic "Read wait_expose.vi"("error in (no error)"=w1517, "Channel in"=w1516) -> ("error out"=w1512:errorcluster, "wait_expose"=w1515:bool)  [unwired: 7 in, 1 out]
          n586 = Select(t=u32 323, s=w1515, f=u32 325 ("t")) -> (s? t:f=w1507:u32)
          n587 = case shown="False" w1508 {
            tunnel: [u32 0 ("f") w1551] -> w1514
            tunnel: w1513 -> [w1545 w1549]
            tunnel: w1512 -> [w1539 w1550]
            tunnel: [w1535 w1550] -> w1511
            tunnel: [w1534 w1549] -> w1509
            tunnel: w1507 -> [_ w1551]
            frame False {
              # "20241108:\nPassa aqui também quando é polarimetria com 1 posicao. \nNeste caso, deve recarregar SEQ antes de encerrar; então recarrega sempre aqui."
              n588 = call "Read Instrument.lvclass.vi"("error in (no error)"=w1539, "S4ACS_GUI in"=w1545) -> ("error out"=w1546:errorcluster, "Instrument.lvclass"=w1547:refnum<class "Instrument.lvclass">, "S4ACS_GUI out"=w1544:refnum<class "S4GUI.lvclass">)  [unwired: 7 in]
              n589 = call "Read WPROT.vi"("error in (no error)"=w1546, "Instrument in"=w1547) -> ("error out"=w1537:errorcluster, "Opt_Selector.lvclass"=w1541:refnum<class "Opt_Selector.lvclass">, "Instrument out"=w1543:refnum<class "Instrument.lvclass">)  [unwired: 7 in]
              n590 = call-dynamic "Read sequencia_ant.vi"("error in (no error)"=w1537, "Opt_Selector in"=w1541) -> ("error out"=w1532:errorcluster, "sequencia_ant"=w1531:u16, "Opt_Selector out"=w1533:refnum<class "Opt_Selector.lvclass">)  [unwired: 7 in]
              n591 = call-dynamic "Write sequencia.vi"("error in (no error)"=w1532, "sequencia"=w1531, "Opt_Selector in"=w1533) -> ("error out"=w1536:errorcluster, "Opt_Selector out"=w1540:refnum<class "Opt_Selector.lvclass">)  [unwired: 7 in]
              n592 = call "Write WPROT.vi"("error in (no error)"=w1536, "Opt_Selector.lvclass"=w1540, "Instrument in"=w1543) -> ("error out"=w1538:errorcluster, "Instrument out"=w1542:refnum<class "Instrument.lvclass">)  [unwired: 7 in]
              n593 = call "Write Instrument.lvclass.vi"("error in (no error)"=w1538, "Instrument.lvclass"=w1542, "S4ACS_GUI in"=w1544) -> ("error out"=w1535:errorcluster, "S4ACS_GUI out"=w1534:refnum<class "S4GUI.lvclass">)  [unwired: 7 in]
            }
            frame True {
            }
          }
          n594 = call-dynamic "Write Acq_state.vi"("error in (no error)"=w1511, "Acq_state"=w1514, "Acquisition in"=w1510) -> ("error out"=w1529:errorcluster, "Acquisition out"=w1530:refnum<class "Acquisition.lvclass">)  [unwired: 7 in]
        }
        frame 1325 {
          n595 = disable-structure shown="Enabled" {
            disable-tunnel: w1557 -> [w1573 w1601]
            disable-tunnel: w1556 -> [w1572 w1600]
            disable-tunnel: [w1565 w1596] -> w1555
            disable-tunnel: [w1559 w1597] -> w1554
            disable-tunnel: w1552 -> [_ _]
            disable-tunnel: w1553 -> [_ w1595]
            frame Disabled {
              n596 = call-dynamic "Read Channel.vi"("error in (no error)"=w1572, "Acquisition in"=w1573) -> ("error out"=w1570:errorcluster, "Channel.lvclass"=w1571:refnum<class "Channel.lvclass">, "Acquisition out"=w1567:refnum<class "Acquisition.lvclass">)  [unwired: 7 in]
              n597 = call-dynamic "Read ciclos.vi"("error in (no error)"=w1570, "Channel in"=w1571) -> ("error out"=w1562:errorcluster, "ciclos"=w1569:u32, "Channel out"=w1563:refnum<class "Channel.lvclass">)  [unwired: 7 in]
              n598 = Decrement(x=w1569) -> (x-1=w1574:u32)
              n599 = Greater Than 0?(x=w1574) -> (x > 0?=w1578:bool)
              n600 = case shown="True" w1578 {
                selector: w1578 -> [w1580 w1582]
                tunnel: w1574 -> [_ w1581]
                tunnel: [w1580 w1582] -> w1577
                tunnel: [u32 0 w1581] -> w1568
                frame False {
                }
                frame True {
                }
              }
              n601 = call-dynamic "Write ciclos.vi"("error in (no error)"=w1562, "ciclos"=w1568, "Channel in"=w1563) -> ("error out"=w1561:errorcluster, "Channel out"=w1564:refnum<class "Channel.lvclass">)  [unwired: 7 in]
              n602 = call-dynamic "Write Channel.vi"("error in (no error)"=w1561, "Channel.lvclass"=w1564, "Acquisition in"=w1567) -> ("error out"=w1560:errorcluster, "Acquisition out"=w1566:refnum<class "Acquisition.lvclass">)  [unwired: 7 in]
              n603 = Select(t=u32 323, s=w1577, f=u32 0) -> (s? t:f=w1558:u32)
              n604 = call-dynamic "Write Acq_state.vi"("error in (no error)"=w1560, "Acq_state"=w1558, "Acquisition in"=w1566) -> ("error out"=w1559:errorcluster, "Acquisition out"=w1565:refnum<class "Acquisition.lvclass">)  [unwired: 7 in]
            }
            frame Enabled {
              n605 = call-dynamic "Read Channel.vi"("error in (no error)"=w1600, "Acquisition in"=w1601) -> ("error out"=w1591:errorcluster, "Channel.lvclass"=w1593:refnum<class "Channel.lvclass">, "Acquisition out"=w1602:refnum<class "Acquisition.lvclass">)  [unwired: 7 in]
              n606 = call-dynamic "Read PrevCyclesDone.vi"("error in (no error)"=w1591, "Channel in"=w1593) -> ("error out"=w1590:errorcluster, "PrevCyclesDone"=w1589:u32, "Channel out"=w1592:refnum<class "Channel.lvclass">)  [unwired: 7 in]
              n607 = call-dynamic "Read CyclesDone.vi"("error in (no error)"=w1590, "Channel in"=w1592) -> ("error out"=w1586:errorcluster, "CyclesDone"=w1598:u32, "Channel out"=w1588:refnum<class "Channel.lvclass">)  [unwired: 7 in]
              n608 = Greater?(x=w1598, y=w1589) -> (0:w1599:bool)
              n609 = case shown="True" w1599 {
                tunnel: w1598 -> [_ w1606]
                tunnel: w1595 -> [w1605 w1612]
                tunnel: [w1605 w1611] -> w1594
                tunnel: [w1604 w1609] -> w1587
                tunnel: w1588 -> [w1604 w1610]
                tunnel: w1586 -> [w1603 w1608]
                tunnel: [w1603 w1607] -> w1585
                frame False {
                }
                frame True {
                  n610 = call-dynamic "Write PrevCyclesDone.vi"("error in (no error)"=w1608, "PrevCyclesDone"=w1606, "Channel in"=w1610) -> ("error out"=w1607:errorcluster, "Channel out"=w1609:refnum<class "Channel.lvclass">)  [unwired: 7 in]
                  n611 = Increment(x=w1612) -> (x+1=w1611:u32)
                }
              }
              n612 = call-dynamic "Write Channel.vi"("error in (no error)"=w1585, "Channel.lvclass"=w1587, "Acquisition in"=w1602) -> ("error out"=w1584:errorcluster, "Acquisition out"=w1583:refnum<class "Acquisition.lvclass">)  [unwired: 7 in]
              n613 = call-dynamic "Write Acq_state.vi"("error in (no error)"=w1584, "Acq_state"=w1594, "Acquisition in"=w1583) -> ("error out"=w1597:errorcluster, "Acquisition out"=w1596:refnum<class "Acquisition.lvclass">)  [unwired: 7 in]
            }
          }
        }
        frame 1326 {
          n614 = call-dynamic "Read Channel.vi"("error in (no error)"=w1620, "Acquisition in"=w1621) -> ("error out"=w1616:errorcluster, "Channel.lvclass"=w1619:refnum<class "Channel.lvclass">, "Acquisition out"=w1617:refnum<class "Acquisition.lvclass">)  [unwired: 7 in]
          n615 = call-dynamic "Read CyclesDone.vi"("Channel in"=w1619) -> ("error out"=w1613:errorcluster, "CyclesDone"=w1614:u32, "Channel out"=w1618:refnum<class "Channel.lvclass">)  [unwired: 8 in]
          n616 = call-dynamic "Read ciclos.vi"("error in (no error)"=w1613, "Channel in"=w1618) -> ("ciclos"=w1615:u32)  [unwired: 7 in, 2 out]
          n617 = Unbundle By Name(w1626) -> ("mode EXPOSE"=w1625:bool)
          n618 = Subtract(x=w1615, y=w1614) -> (x-y=w1632:u32)
          n619 = Select(t=u32 323, s=w1625, f=u32 325 ("t")) -> (s? t:f=w1622:u32)
          n620 = Greater Than 0?(x=w1632) -> (x > 0?=w1631:bool)
          n621 = Select(t=w1622, s=w1631, f=u32 0) -> (s? t:f=w1629:u32)
          n622 = call-dynamic "Write Acq_state.vi"("error in (no error)"=w1616, "Acq_state"=w1629, "Acquisition in"=w1617) -> ("error out"=w1627:errorcluster, "Acquisition out"=w1628:refnum<class "Acquisition.lvclass">)  [unwired: 7 in]
        }
        frame 360 {
          w1638 = u32 0 ("cyclesDone")
          # "Inicia o Ticks com\nvalor do relogio atual"
          # "Espera até 40 x 0.25s (= 10s) para\nmecanismo entrar em READY"
          # "Busca próximo valor de foco..."
          n623 = flat-sequence {
            tunnel: w1641 -> [w1668]
            tunnel: [w1668] -> w1658
            frame #0 {
              n624 = Tick Count (ms)() -> (millisecond timer value=→"time7":u32)
            }
          }
          n625 = call-dynamic "Read TelFocus.lvclass.vi"("error in (no error)"=w1658, "S4GUI in"=w1642) -> ("error out"=w1666:errorcluster, "TelFocus.lvclass"=w1667:refnum<class "TelFocus.lvclass">, "S4GUI out"=w1665:refnum<class "S4GUI.lvclass">)  [unwired: 7 in]
          n626 = call-dynamic "GetNextFocus.vi"("error in (no error)"=w1666, "TelFocus in"=w1667) -> ("error out"=w1656:errorcluster, "TelFocus out"=w1657:refnum<class "TelFocus.lvclass">)  [unwired: 8 in]
          n627 = call-dynamic "Read SecMirror.lvclass.vi"("error in (no error)"=w1656, "TelFocus in"=w1657) -> ("error out"=w1643:errorcluster, "SecMirror.lvclass"=w1644:refnum<class "SecMirror.lvclass">, "TelFocus out"=w1660:refnum<class "TelFocus.lvclass">)  [unwired: 7 in]
          n628 = call-dynamic "Read State Machine.vi"("error in (no error)"=w1643, "Device in"=w1644) -> ("error out"=w1653:errorcluster, "State Machine.lvclass"=w1655:refnum<class "State Machine.lvclass">, "Device out"=w1652:refnum<class "SecMirror.lvclass">)  [unwired: 7 in]
          n629 = call "Next State.vi"("error in (no error)"=w1653, "New_State"=1, "State Machine in"=w1655) -> ("error out"=w1650:errorcluster, "State Machine out"=w1651:refnum<class "State Machine.lvclass">)  [unwired: 7 in]
          n630 = call-dynamic "Write Timer.vi"("error in (no error)"=w1650, "Timer"=u32 40, "State Machine in"=w1651) -> ("error out"=w1647:errorcluster, "State Machine out"=w1648:refnum<class "State Machine.lvclass">)  [unwired: 7 in]
          n631 = call-dynamic "Init Ticks2.vi"("error in (no error)"=w1647, "State Machine in"=w1648) -> ("error out"=w1646:errorcluster, "State Machine out"=w1645:refnum<class "State Machine.lvclass">)  [unwired: 8 in]
          n632 = call-dynamic "Write State Machine.vi"("error in (no error)"=w1646, "State Machine.lvclass"=w1645, "Device in"=w1652) -> ("error out"=w1659:errorcluster, "Device out"=w1661:refnum<class "SecMirror.lvclass">)  [unwired: 7 in]
          n633 = call-dynamic "Write SecMirror.lvclass.vi"("error in (no error)"=w1659, "SecMirror.lvclass"=w1661, "TelFocus in"=w1660) -> ("error out"=w1663:errorcluster, "TelFocus out"=w1662:refnum<class "TelFocus.lvclass">)  [unwired: 7 in]
          n634 = call-dynamic "Write TelFocus.lvclass.vi"("error in (no error)"=w1663, "TelFocus.lvclass"=w1662, "S4GUI in"=w1665) -> ("error out"=w1635:errorcluster, "S4GUI out"=w1664:refnum<class "S4GUI.lvclass">)  [unwired: 7 in]
          n635 = Bundle By Name(cluster=w1664, "cyclesDone"=w1638, "sequesDone"=w1638) -> (w1639:refnum<class "S4GUI.lvclass">)
          n636 = Increment(x=w1640) -> (x+1=w1634:u32)
          n637 = call-dynamic "Write Acq_state.vi"("error in (no error)"=w1635, "Acq_state"=w1634, "Acquisition in"=w1637) -> ("error out"=w1633:errorcluster, "Acquisition out"=w1636:refnum<class "Acquisition.lvclass">)  [unwired: 7 in]
        }
        frame 361 {
          # "Timeout= 25s + distancia do target (cada 1000um=1s)"
          # "Espera terminar o movimento do foco do 2ndario para disparar\n a aquisição do canal."
          n638 = flat-sequence {
            tunnel: w1690 -> [w1726]
            tunnel: [w1726] -> w1706
            frame #0 {
              n639 = Tick Count (ms)() -> (millisecond timer value=w1725:u32)
              "time 8" <- w1725
              n640 = local read "time7"() -> (w1724:u32)
              n641 = Subtract(x=w1725, y=w1724) -> (x-y=→"delay 78":u32)
            }
          }
          n642 = call-dynamic "Read TelFocus.lvclass.vi"("error in (no error)"=w1706, "S4GUI in"=w1691) -> ("error out"=w1715:errorcluster, "TelFocus.lvclass"=w1716:refnum<class "TelFocus.lvclass">, "S4GUI out"=w1712:refnum<class "S4GUI.lvclass">)  [unwired: 7 in]
          n643 = call-dynamic "Read SecMirror.lvclass.vi"("error in (no error)"=w1715, "TelFocus in"=w1716) -> ("error out"=w1679:errorcluster, "SecMirror.lvclass"=w1682:refnum<class "SecMirror.lvclass">, "TelFocus out"=w1714:refnum<class "TelFocus.lvclass">)  [unwired: 7 in]
          n644 = call-dynamic "Read position.vi"("error in (no error)"=w1679, "SecMirror in"=w1682) -> ("error out"=w1688:errorcluster, "position"=w1676:i32, "SecMirror out"=w1681:refnum<class "SecMirror.lvclass">)  [unwired: 7 in]
          n645 = call-dynamic "Read target.vi"("error in (no error)"=w1688, "SecMirror in"=w1681) -> ("error out"=w1678:errorcluster, "target"=w1687:i32, "SecMirror out"=w1680:refnum<class "SecMirror.lvclass">)  [unwired: 7 in]
          n646 = Subtract(x=w1687, y=w1676) -> (x-y=w1686:i32)
          n647 = Absolute Value(x=w1686) -> (abs(x)=w1684:i32)
          n648 = call-dynamic "Read State Machine.vi"("error in (no error)"=w1678, "Device in"=w1680) -> ("error out"=w1698:errorcluster, "State Machine.lvclass"=w1701:refnum<class "State Machine.lvclass">, "Device out"=w1709:refnum<class "SecMirror.lvclass">)  [unwired: 7 in]
          n649 = To Unsigned Long Integer(number=w1684) -> (unsigned 32bit integer=w1685:u32)
          n650 = Add(x=w1685, y=u32 25000 ("period")) -> (x+y=w1677:u32)
          n651 = call-dynamic "Verif Clock 2.vi"("error in (no error)"=w1698, "period (ms)"=w1677, "State Machine in"=w1701) -> ("error out"=w1697:errorcluster, "time elapsed"=→"time elapsed 2":u32, "State Machine out"=w1700:refnum<class "State Machine.lvclass">)  [unwired: 6 in]
          n652 = call-dynamic "Read Timeout 2.vi"("error in (no error)"=w1697, "State Machine in"=w1700) -> ("error out"=w1696:errorcluster, "Timeout 2"=w1702:bool, "State Machine out"=w1699:refnum<class "State Machine.lvclass">)  [unwired: 7 in]
          n653 = call-dynamic "Read State.vi"("error in (no error)"=w1696, "State Machine in"=w1699) -> ("error out"=w1704:errorcluster, "State"=w1707:i32, "State Machine out"=w1705:refnum<class "State Machine.lvclass">)  [unwired: 7 in]
          n654 = call-dynamic "Write State Machine.vi"("error in (no error)"=w1704, "State Machine.lvclass"=w1705, "Device in"=w1709) -> ("error out"=w1708:errorcluster, "Device out"=w1710:refnum<class "SecMirror.lvclass">)  [unwired: 7 in]
          n655 = call-dynamic "Write SecMirror.lvclass.vi"("error in (no error)"=w1708, "SecMirror.lvclass"=w1710, "TelFocus in"=w1714) -> ("error out"=w1711:errorcluster, "TelFocus out"=w1713:refnum<class "TelFocus.lvclass">)  [unwired: 7 in]
          n656 = call-dynamic "Write TelFocus.lvclass.vi"("error in (no error)"=w1711, "TelFocus.lvclass"=w1713, "S4GUI in"=w1712) -> ("error out"=w1673:errorcluster, "S4GUI out"=w1695:refnum<class "S4GUI.lvclass">)  [unwired: 7 in]
          n657 = Equal To 0?(x=w1707) -> (x = 0?=w1703:bool)
          n658 = case shown="True" w1702 {
            tunnel: w1689 -> [w1718 _]
            tunnel: [w1718 u32 0 ("Obs_state")] -> w1693
            tunnel: w1695 -> [w1717 w1722]
            tunnel: [w1717 w1721] -> w1675
            frame False {
            }
            frame True {
              n659 = Bundle By Name(cluster=w1722, "Error Msg"="ERROR: moving telescope focus timeout  (S4GUI:HandleObservationAsync.vi - state 361)") -> (w1721:refnum<class "S4GUI.lvclass">)
            }
          }
          n660 = Increment(x=w1693) -> (x+1=w1692:u32)
          n661 = Select(t=w1692, s=w1703, f=w1693) -> (s? t:f=w1670:u32)
          n662 = call-dynamic "Write Acq_state.vi"("error in (no error)"=w1673, "Acq_state"=w1670, "Acquisition in"=w1674) -> ("error out"=w1671:errorcluster, "Acquisition out"=w1672:refnum<class "Acquisition.lvclass">)  [unwired: 7 in]
        }
        frame 362 {
          # "Dispara o comando para o dispositivo corrente."
          n663 = call-dynamic "Read Channel.vi"("error in (no error)"=w1736, "Acquisition in"=w1737) -> ("error out"=w1743:errorcluster, "Channel.lvclass"=w1742:refnum<class "Channel.lvclass">, "Acquisition out"=w1747:refnum<class "Acquisition.lvclass">)  [unwired: 7 in]
          n664 = call-dynamic "Read State Machine.vi"("error in (no error)"=w1743, "Device in"=w1742) -> ("error out"=w1744:errorcluster, "State Machine.lvclass"=w1746:refnum<class "State Machine.lvclass">, "Device out"=w1740:refnum<class "Channel.lvclass">)  [unwired: 7 in]
          n665 = call "Next State.vi"("error in (no error)"=w1744, "New_State"=58, "State Machine in"=w1746) -> ("error out"=w1729:errorcluster, "State Machine out"=w1730:refnum<class "State Machine.lvclass">)  [unwired: 7 in]
          n666 = call-dynamic "Write State Machine.vi"("error in (no error)"=w1729, "State Machine.lvclass"=w1730, "Device in"=w1740) -> ("error out"=w1739:errorcluster, "Device out"=w1741:refnum<class "Channel.lvclass">)  [unwired: 7 in]
          n667 = Increment(x=w1738) -> (x+1=w1735:u32)
          n668 = call-dynamic "Write Channel.vi"("error in (no error)"=w1739, "Channel.lvclass"=w1741, "Acquisition in"=w1747) -> ("error out"=w1733:errorcluster, "Acquisition out"=w1732:refnum<class "Acquisition.lvclass">)  [unwired: 7 in]
          n669 = call-dynamic "Write Acq_state.vi"("error in (no error)"=w1733, "Acq_state"=w1735, "Acquisition in"=w1732) -> ("error out"=w1728:errorcluster, "Acquisition out"=w1731:refnum<class "Acquisition.lvclass">)  [unwired: 7 in]
          n670 = flat-sequence {
            tunnel: w1728 -> [w1748]
            tunnel: [w1748] -> w1727
            frame #0 {
              n671 = Tick Count (ms)() -> (millisecond timer value=→"time9":u32)
            }
          }
        }
        frame 363 {
          # "Espera terminar a execução do comando atual \nantes de ir ao proximo passo da Observação."
          n672 = call-dynamic "Read Channel.vi"("error in (no error)"=w1766, "Acquisition in"=w1767) -> ("error out"=w1759:errorcluster, "Channel.lvclass"=w1760:refnum<class "Channel.lvclass">, "Acquisition out"=w1775:refnum<class "Acquisition.lvclass">)  [unwired: 7 in]
          n673 = call-dynamic "Read wait_expose.vi"("error in (no error)"=w1759, "Channel in"=w1760) -> ("error out"=w1757:errorcluster, "wait_expose"=w1755:bool, "Channel out"=w1758:refnum<class "Channel.lvclass">)  [unwired: 7 in]
          n674 = call-dynamic "Read State Machine.vi"("error in (no error)"=w1757, "Device in"=w1758) -> ("error out"=w1769:errorcluster, "State Machine.lvclass"=w1771:refnum<class "State Machine.lvclass">, "Device out"=w1773:refnum<class "Channel.lvclass">)  [unwired: 7 in]
          n675 = call-dynamic "Read State.vi"("error in (no error)"=w1769, "State Machine in"=w1771) -> ("error out"=w1768:errorcluster, "State"=w1751:i32, "State Machine out"=w1770:refnum<class "State Machine.lvclass">)  [unwired: 7 in]
          n676 = call-dynamic "Write State Machine.vi"("error in (no error)"=w1768, "State Machine.lvclass"=w1770, "Device in"=w1773) -> ("error out"=w1772:errorcluster, "Device out"=w1774:refnum<class "Channel.lvclass">)  [unwired: 7 in]
          n677 = Equal To 0?(x=w1751) -> (x = 0?=w1750:bool)
          n678 = call-dynamic "Write Channel.vi"("error in (no error)"=w1772, "Channel.lvclass"=w1774, "Acquisition in"=w1775) -> ("error out"=w1753:errorcluster, "Acquisition out"=w1765:refnum<class "Acquisition.lvclass">)  [unwired: 7 in]
          n679 = Increment(x=w1761) -> (x+1=w1754:u32)
          n680 = Select(t=w1754, s=w1750, f=w1761) -> (s? t:f=w1764:u32)
          n681 = call-dynamic "Write Acq_state.vi"("error in (no error)"=w1753, "Acq_state"=w1764, "Acquisition in"=w1765) -> ("error out"=w1762:errorcluster, "Acquisition out"=w1763:refnum<class "Acquisition.lvclass">)  [unwired: 7 in]
          n682 = Bundle By Name(cluster=w1752, "mode EXPOSE"=w1755) -> (w1756:refnum<class "S4GUI.lvclass">)
        }
        frame 364 {
          n683 = flat-sequence {
            tunnel: [w1791] -> w1779
            tunnel: w1780 -> [w1791]
            tunnel: [w1786] -> w1776
            frame #0 {
              n684 = local read "time9"() -> (w1787:u32)
              n685 = Tick Count (ms)() -> (millisecond timer value=w1790:u32)
              "time 10" <- w1790
              n686 = Subtract(x=w1790, y=w1787) -> (x-y=w1789:u32)
              "delay 89" <- w1789
              n687 = Greater?(x=w1789, y=u32 2000) -> (0:w1786:bool)
            }
          }
          n688 = Increment(x=w1777) -> (x+1=w1784:u32)
          n689 = Select(t=w1784, s=w1776, f=w1777) -> (s? t:f=w1785:u32)
          n690 = call-dynamic "Write Acq_state.vi"("error in (no error)"=w1779, "Acq_state"=w1785, "Acquisition in"=w1778) -> ("error out"=w1781:errorcluster, "Acquisition out"=w1782:refnum<class "Acquisition.lvclass">)  [unwired: 7 in]
        }
        frame 365 {
          # "Dispara o comando para o dispositivo corrente."
          n691 = call-dynamic "Read Channel.vi"("error in (no error)"=w1800, "Acquisition in"=w1801) -> ("error out"=w1807:errorcluster, "Channel.lvclass"=w1806:refnum<class "Channel.lvclass">, "Acquisition out"=w1811:refnum<class "Acquisition.lvclass">)  [unwired: 7 in]
          n692 = call-dynamic "Read State Machine.vi"("error in (no error)"=w1807, "Device in"=w1806) -> ("error out"=w1808:errorcluster, "State Machine.lvclass"=w1810:refnum<class "State Machine.lvclass">, "Device out"=w1804:refnum<class "Channel.lvclass">)  [unwired: 7 in]
          n693 = call "Next State.vi"("error in (no error)"=w1808, "New_State"=50, "State Machine in"=w1810) -> ("error out"=w1792:errorcluster, "State Machine out"=w1793:refnum<class "State Machine.lvclass">)  [unwired: 7 in]
          n694 = call-dynamic "Write State Machine.vi"("error in (no error)"=w1792, "State Machine.lvclass"=w1793, "Device in"=w1804) -> ("error out"=w1803:errorcluster, "Device out"=w1805:refnum<class "Channel.lvclass">)  [unwired: 7 in]
          n695 = Increment(x=w1802) -> (x+1=w1799:u32)
          n696 = call-dynamic "Write Channel.vi"("error in (no error)"=w1803, "Channel.lvclass"=w1805, "Acquisition in"=w1811) -> ("error out"=w1797:errorcluster, "Acquisition out"=w1796:refnum<class "Acquisition.lvclass">)  [unwired: 7 in]
          n697 = call-dynamic "Write Acq_state.vi"("error in (no error)"=w1797, "Acq_state"=w1799, "Acquisition in"=w1796) -> ("error out"=w1794:errorcluster, "Acquisition out"=w1795:refnum<class "Acquisition.lvclass">)  [unwired: 7 in]
        }
        frame 366 {
          # "Espera terminar a execução do comando atual \nantes de ir ao proximo passo da Observação."
          n698 = call-dynamic "Read Channel.vi"("error in (no error)"=w1829, "Acquisition in"=w1830) -> ("error out"=w1819:errorcluster, "Channel.lvclass"=w1820:refnum<class "Channel.lvclass">, "Acquisition out"=w1838:refnum<class "Acquisition.lvclass">)  [unwired: 7 in]
          n699 = call-dynamic "Read wait_expose.vi"("error in (no error)"=w1819, "Channel in"=w1820) -> ("error out"=w1817:errorcluster, "wait_expose"=w1815:bool, "Channel out"=w1818:refnum<class "Channel.lvclass">)  [unwired: 7 in]
          n700 = call-dynamic "Read State Machine.vi"("error in (no error)"=w1817, "Device in"=w1818) -> ("error out"=w1832:errorcluster, "State Machine.lvclass"=w1834:refnum<class "State Machine.lvclass">, "Device out"=w1836:refnum<class "Channel.lvclass">)  [unwired: 7 in]
          n701 = call-dynamic "Read State.vi"("error in (no error)"=w1832, "State Machine in"=w1834) -> ("error out"=w1831:errorcluster, "State"=w1823:i32, "State Machine out"=w1833:refnum<class "State Machine.lvclass">)  [unwired: 7 in]
          n702 = call-dynamic "Write State Machine.vi"("error in (no error)"=w1831, "State Machine.lvclass"=w1833, "Device in"=w1836) -> ("error out"=w1835:errorcluster, "Device out"=w1837:refnum<class "Channel.lvclass">)  [unwired: 7 in]
          n703 = Greater?(x=w1823, y=53) -> (0:w1822:bool)
          n704 = call-dynamic "Write Channel.vi"("error in (no error)"=w1835, "Channel.lvclass"=w1837, "Acquisition in"=w1838) -> ("error out"=w1813:errorcluster, "Acquisition out"=w1828:refnum<class "Acquisition.lvclass">)  [unwired: 7 in]
          n705 = Increment(x=w1821) -> (x+1=w1814:u32)
          n706 = Select(t=w1814, s=w1822, f=w1821) -> (s? t:f=w1827:u32)
          n707 = call-dynamic "Write Acq_state.vi"("error in (no error)"=w1813, "Acq_state"=w1827, "Acquisition in"=w1828) -> ("error out"=w1825:errorcluster, "Acquisition out"=w1826:refnum<class "Acquisition.lvclass">)  [unwired: 7 in]
          n708 = Bundle By Name(cluster=w1812, "mode EXPOSE"=w1815) -> (w1816:refnum<class "S4GUI.lvclass">)
        }
        frame 367 {
          # "SEQS_DONE = 0,1,2,...,n,0,1,..."
          n709 = Unbundle By Name(w1839) -> ("sequesDone"=w1848:u32, "cyclesDone"=w1843:u32)
          n710 = call-dynamic "Read Channel.vi"("error in (no error)"=w1859, "Acquisition in"=w1860) -> ("error out"=w1851:errorcluster, "Channel.lvclass"=w1852:refnum<class "Channel.lvclass">, "Acquisition out"=w1861:refnum<class "Acquisition.lvclass">)  [unwired: 7 in]
          n711 = call-dynamic "Read CyclesDone.vi"("error in (no error)"=w1851, "Channel in"=w1852) -> ("error out"=w1853:errorcluster, "CyclesDone"=w1844:u32, "Channel out"=w1854:refnum<class "Channel.lvclass">)  [unwired: 7 in]
          n712 = call-dynamic "Read SequesDone.vi"("error in (no error)"=w1853, "Channel in"=w1854) -> ("error out"=w1849:errorcluster, "SequesDone"=w1845:u32, "Channel out"=w1850:refnum<class "Channel.lvclass">)  [unwired: 6 in, 1 out]
          n713 = Not Equal?(x=w1844, y=w1843) -> (x != y?=w1841:bool)
          n714 = Not Equal?(x=w1845, y=w1848) -> (x != y?=w1842:bool)
          n715 = call-dynamic "Write Channel.vi"("error in (no error)"=w1849, "Channel.lvclass"=w1850, "Acquisition in"=w1861) -> ("error out"=w1857:errorcluster, "Acquisition out"=w1858:refnum<class "Acquisition.lvclass">)  [unwired: 7 in]
          n716 = Or(x=w1842, y=w1841) -> (x .or. y?=w1840:bool)
          n717 = case shown="True" w1840 {
            tunnel: [w1862 w1863] -> w1847
            tunnel: w1846 -> [w1862 w1864]
            tunnel: w1845 -> [_ _]
            tunnel: w1844 -> [_ _]
            frame False {
            }
            frame True {
              n718 = Increment(x=w1864) -> (x+1=w1863:u32)
            }
          }
          n719 = call-dynamic "Write Acq_state.vi"("error in (no error)"=w1857, "Acq_state"=w1847, "Acquisition in"=w1858) -> ("error out"=w1855:errorcluster, "Acquisition out"=w1856:refnum<class "Acquisition.lvclass">)  [unwired: 7 in]
        }
        frame 368 {
          n720 = Unbundle By Name(w1872) -> ("TelFocus.lvclass"=w1874:refnum<class "TelFocus.lvclass">)
          n721 = call-dynamic "VerifSteps.vi"("error in (no error)"=w1871, "TelFocus in"=w1874) -> ("error out"=w1868:errorcluster, "continua?"=w1875:bool, "TelFocus out"=w1873:refnum<class "TelFocus.lvclass">)  [unwired: 7 in]
          n722 = Bundle By Name(cluster=w1872, "TelFocus.lvclass"=w1873) -> (w1867:refnum<class "S4GUI.lvclass">)
          n723 = Select(t=u32 360, s=w1875, f=u32 0) -> (s? t:f=w1869:u32)
          n724 = call-dynamic "Write Acq_state.vi"("error in (no error)"=w1868, "Acq_state"=w1869, "Acquisition in"=w1870) -> ("error out"=w1865:errorcluster, "Acquisition out"=w1866:refnum<class "Acquisition.lvclass">)  [unwired: 7 in]
        }
        frame 400 {
          # "Estado de \"Pause\": fica parado aqui até o botão START seja pressionado."
        }
        frame 500 {
          # "Espera terminar o envio de RESUME para todos os ACS."
          # "Estado de \"Pause\": fica parado aqui até o botão RESUME seja pressionado."
          n725 = call-dynamic "VerifyAcqIdle.vi"("error in (no error)"=w1882, "S4GUI in"=w1883) -> ("error out"=w1886:errorcluster, "idle"=w1888:bool, "S4GUI out"=w1887:refnum<class "S4GUI.lvclass">)  [unwired: 6 in, 1 out]
          n726 = case shown="True" w1888 {
            tunnel: w1887 -> [w1890 w1900]
            tunnel: [w1890 w1892] -> w1885
            tunnel: w1886 -> [w1889 w1899]
            tunnel: [w1889 w1893] -> w1884
            frame False {
            }
            frame True {
              n727 = call-dynamic "LoadPrevAcqRunState.vi"("error in (no error)"=w1899, "S4GUI in"=w1900) -> ("error out"=w1894:errorcluster, "S4GUI out"=w1895:refnum<class "S4GUI.lvclass">)  [unwired: 8 in]
              n728 = Tick Count (ms)() -> (millisecond timer value=w1891:u32)
              n729 = call-dynamic "Read Obs_prevstate.vi"("error in (no error)"=w1894, "S4ACS_GUI in"=w1895) -> ("error out"=w1898:errorcluster, "Obs_prevstate"=w1896:u32, "S4ACS_GUI out"=w1897:refnum<class "S4GUI.lvclass">)  [unwired: 7 in]
              n730 = local write "time307"(w1891) -> ()
              n731 = local write "time1"(w1891) -> ()
              n732 = call-dynamic "Write Obs_state.vi"("error in (no error)"=w1898, "Obs_state"=w1896, "S4ACS_GUI in"=w1897) -> ("error out"=w1893:errorcluster, "S4ACS_GUI out"=w1892:refnum<class "S4GUI.lvclass">)  [unwired: 7 in]
            }
          }
        }
      }
    }
    frame Error {
    }
  }
  "error out" <- w5
  "S4ACS_GUI out" <- w3
  "Acquisition.lvclass Out" <- w1
